vi "RF_NCS_ThoraxAbdomen_USRP_B200.vi"() -> (2 "Resp Amp":dbl[](graph), 3 "Heart Amp":dbl[](graph), 4 "# queue 2":i32)   [LabVIEW 2016]
uses:
  <instrlib>/niUSRP/niUSRP Timestamp.ctl
  <vilib>/Utility/miscctls.llb/LVDateTimeRec.ctl
  <vilib>/sound2/lvsound2.llb/Sound File Position.ctl
  <vilib>/Analysis/3filter.llb/Filter Passband Type.ctl
  <vilib>/sound2/lvsound2.llb/Sampling Mode.ctl
  <instrlib>/niUSRP/niUSRP Configure Time Start Trigger.vi
  <vilib>/Platform/browser.llb/Open URL in Default Browser (string).vi
  <instrlib>/niUSRP/niUSRP Write Tx Data (CDB).vi
  <instrlib>/niUSRP/niUSRP Fetch Rx Data (CDB).vi
  <vilib>/Analysis/3filter.llb/Butterworth Filter (DBL).vi
  <vilib>/sound2/lvsound2.llb/Sound File Info (path).vi
  <vilib>/sound2/lvsound2.llb/Sound File Read Open.vi
  <vilib>/sound2/lvsound2.llb/Sound File Read (DBL).vi
  <vilib>/sound2/lvsound2.llb/Sound Output Write (DBL).vi
  <vilib>/Analysis/3filter.llb/Butterworth Filter (CDB).vi
  <vilib>/measure/NI_MABase.lvlib
  <vilib>/Analysis/NI_AALBase.lvlib
  <vilib>/Analysis/NI_AALPro.lvlib
panel:
  in  "SDR1\nInitPhase":i32
  in  "Flush Rx2":bool
  out "String 3":string
  out "element":dbl[][](array[numeric])
  out "appended array":dbl[][](array[numeric])
  in  "SDR2 Carrier \nfrequency (Hz)":dbl=1900000000.0
  out "String 2":string
  out "size(s)":i32[](array[numeric])
  in  "Tab Control 7":enum32{"Amp2 @50kHz", "Ph2 @50kHz"}(tab)
  out "Amp2 @50 kHz":dbl[](graph)
  out "Ph2 @50 kHz":dbl[](graph)
  in  "Tab Control 6":enum32{"Amp1 @500Hz", "Ph1 @500Hz"}(tab)
  out "Amp1 @500Hz":dbl[](graph)
  out "Ph1 @500Hz":dbl[](graph)
  out "String":string
  out "#queue 3":i32
  out "#queue 2":i32
  out "# Rx2DS_Queue":i32=1
  in  "FlushSDR2":bool
  out "error out 2":errorcluster
  in  "Tab Control 8":enum32{"Rx1", "Rx2"}(tab)
  out "IQ Graph":dbl[][](graph)
  out "IQ Graph 2":dbl[][](graph)
  in  "Tab Control 5":enum32{"Amp2 @500Hz", "Ph2 @500Hz"}(tab)
  out "Amp2 @500Hz":dbl[](graph)
  out "Ph2 @500Hz":dbl[](graph)
  in  "Tab Control 4":enum32{"Tx1", "Tx2"}(tab)
  out "Tx1 Waveform Graph":waveform(dbl)[](graph)
  out "Tx2 Waveform graph":waveform(dbl)[](graph)
  in  "Stop 2":bool
  out "Tx2 Waveform":cdb[](array[numeric])
  out "Read:Tx2 IQ Rate":dbl=5000000.0
  out "Read:Rx2 IQ Rate":dbl=5000000.0
  in  "Device2 Name":refnum<k15>="MyB200_2"
  in  "Tx2 Gain":dbl=26.0 format="%#_6f"
  in  "Rx2 Gain":dbl=20.0 format="%#_6f"
  in  "Routine 3,4":T1=2 items=["Absolute"=0, "Relative"=2]
  in  "(2b) Attn Test":T1=2 items=["Absolute"=0, "Relative"=2]
  in  "Routine 5":T1=2 items=["Absolute"=0, "Relative"=2]
  in  "OpenHTML":bool=TRUE
  in  "Play sound":u16(ring) items=["No sound", "Demo normal breathing", "Demo deep breathing", "Demo fast shallow breathing", "Demo breath hold", "Demo cough", "Demo abdomen movement", "Calibration", "Routine 1", "(2a) Calm music", "(2b) Stress test", "Routine 3/4", "Routine 5"]
  in  "Demo cough":T1=2 items=["Absolute"=0, "Relative"=2]
  in  "Demo breath-hold":T1=2 items=["Absolute"=0, "Relative"=2]
  in  "Demo abdomen":T1=2 items=["Absolute"=0, "Relative"=2]
  in  "Demo fast shallow":T1=2 items=["Absolute"=0, "Relative"=2]
  in  "Play/Stop":bool
  in  "Demo normal":T1=2 items=["Absolute"=0, "Relative"=2]
  in  "Demo deep":T1=2 items=["Absolute"=0, "Relative"=2]
  out "Next Task":string
  out "Calib 5":bool caption="Time has Elapsed"
  out "Calib 4":bool caption="Time has Elapsed"
  out "Calib 3":bool caption="Time has Elapsed"
  in  "Calibration":T1=2 items=["Absolute"=0, "Relative"=2]
  out "Calib 1":bool caption="Time has Elapsed"
  out "Current Task time":dbl(slide) scale=0.0..240.0
  in  "(2a) Calm Music":T1=2 items=["Absolute"=0, "Relative"=2]
  out "#2b":bool caption="Time has Elapsed"
  in  "Routine 1":T1=2 items=["Absolute"=0, "Relative"=2]
  in  "number of samples/ch":i32=5000
  out "#5":bool caption="Time has Elapsed"
  out "#2a":bool caption="Time has Elapsed"
  out "#4":bool caption="Time has Elapsed"
  out "#3":bool caption="Time has Elapsed"
  in  "Comments":string
  in  "Tab Control 3":enum32{"Amp Heart", "Ph Heart"}(tab)
  in  "fh 1":dbl=26.0 format="%0.2f"
  in  "fl 1":dbl=0.7 format="%0.4f"
  out "Heart Ph":dbl[](graph)
  in  "fl 3":dbl=0.7 format="%0.4f"
  in  "fh 3":dbl=26.0 format="%0.2f"
  in  "Tab Control 2":enum32{"Amp1 @50kHz", "Ph1 @50kHz"}(tab)
  out "Amp1 @50 kHz":dbl[](graph)
  out "Ph1 @50 kHz":dbl[](graph)
  in  "Tab Control":enum32{"Amp Resp", "Ph Resp"}(tab)
  in  "fl 2":dbl=15.0 format="%0.4f"
  out "Resp Ph":dbl[](graph)
  in  "fl 4":dbl=15.0 format="%0.4f"
  out "ArraySz":i32[](array[numeric])
  in  "Stop Test":bool
  out "#1":bool caption="Time has Elapsed"
  out "Elapsed Time (s)":dbl
  in  "Routine":u16(ring) items=["Not Running", "Test Run", "Routine1", "Routine2a", "Routine2b", "Routine3", "Routine4", "Routine5", "Calib1", "calib3", "Calib4", "Calib5"]
  out "Read:Tx IQ Rate":dbl=5000000.0
  out "Read:Rx IQ Rate":dbl=5000000.0
  out "date time rec":T2
  out "Total Routine Time":dbl(slide) scale=0.0..240.0
  out "Current Task":string
  in  "Case Number":string="0"
  out "CaseNum":i32=1
  out "Save":bool
  out "Flush":bool
  out "Buffer":bool
  out "Output":i32=1
  out "Ch2 Amplitude":dbl step=0.05 format="%#.6g"
  out "Ch1 Amplitude":dbl step=0.05 format="%#.6g"
  out "Dis Sampling Rate":dbl=500.0 format="%#_6p"
  in  "DownSamplingRatio 2":i32=100
  out "Sampling Rate":dbl=50000.0 format="%#_6p"
  out "aapp":dbl[][](array[numeric])
  out "IterationNum":i32=1009
  in  "DownSamplingRatio":i32=40
  out "# elements in queue":i32
  out "BW/2":dbl=1000.0
  out "# queue 1":i32
  in  "Dis1":bool=TRUE
  out "Tx1 Waveform":cdb[](array[numeric])
  in  "SDR1 Carrier\nfrequency [Hz]":dbl=1820000000.0 format="%#_6p"
  out "error out":errorcluster
  in  "Start Trigger Time":T3={"whole seconds"=1, "fractional seconds"=0.0}
  in  "Stop":bool
  in  "Channel 2\nTone Amplitude":dbl=0.25000000000000006 step=0.05 format="%#.6g"
  in  "SDR2\nTone Frequency":dbl=51000.0 format="%#_6p"
  in  "Channel 1\nTone Amplitude":dbl=0.30000000000000004 step=0.05 format="%#.6g"
  in  "SDR1 \nTone Frequency":dbl=51000.0 format="%#_6p"
  in  "Waveform Size":dbl=20000.0
  in  "Device1 Name":refnum<k15>="MyB200"
  in  "Tx1 Gain":dbl=25.0 format="%#_6f"
  in  "Tx IQ Rate":dbl=2000000.0 format="%#_6p"
  in  "Rx1 Gain 1":dbl=26.0 format="%#_6f"
  in  "Rx IQ Rate":dbl=2000000.0 format="%#_6p"
  # "User Instructions"
  # "User Information"
  # "Routine Selection"
  # "Demo \nSounds"
  # "First Tx-Rx: filtered to get heartbeat signal"
  # "Second Tx-Rx: filtered to get respiration signal"
  # "SDR1"
  # "SDR2"
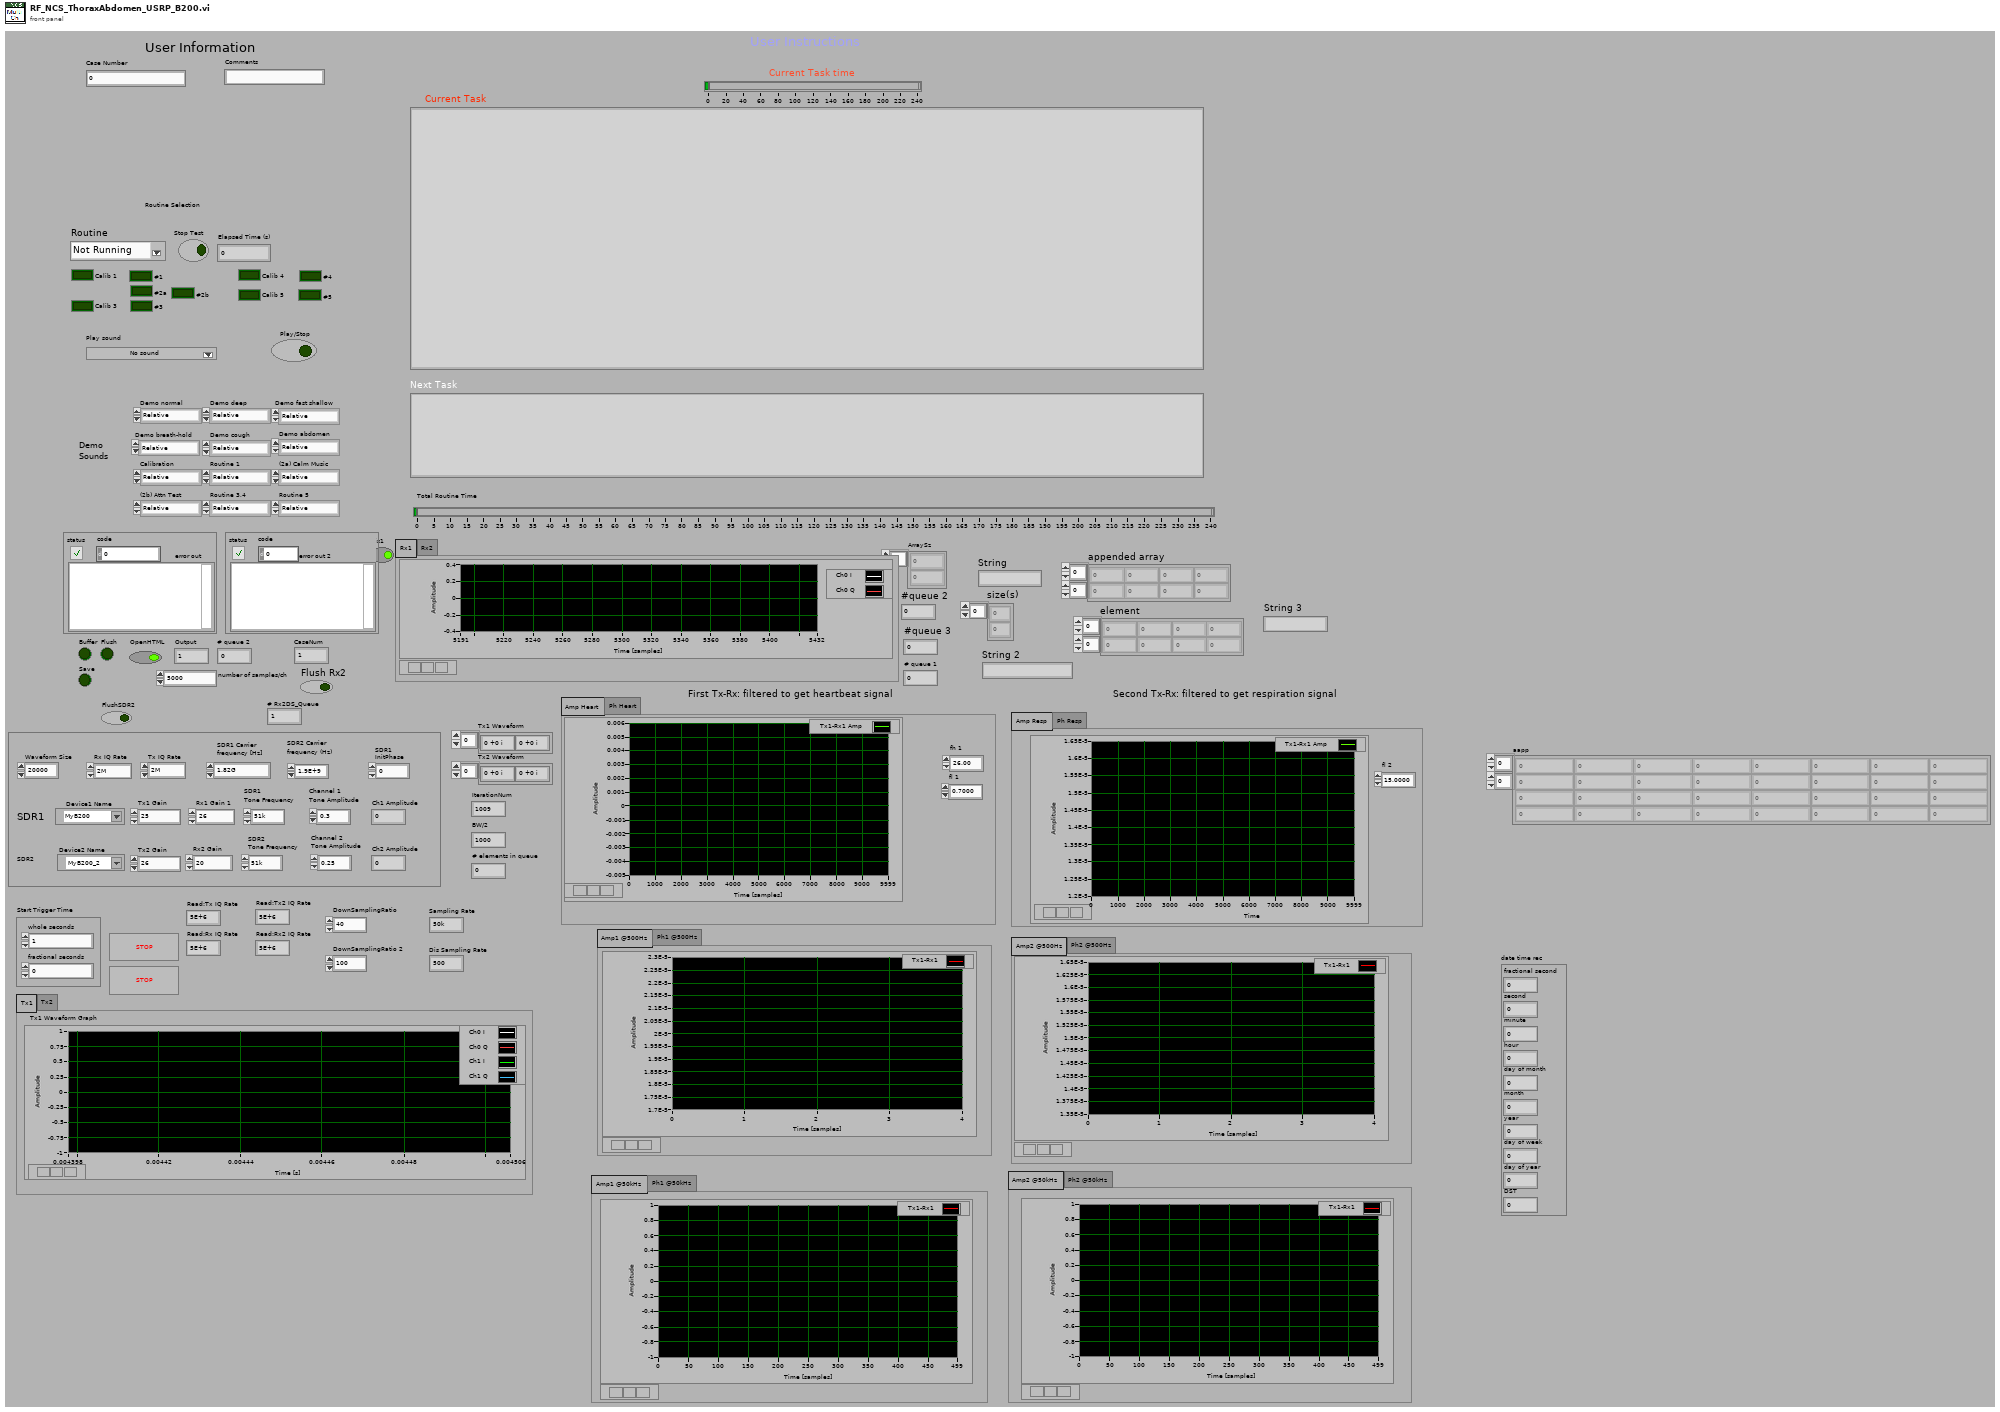
[diagram p1: front panel]
types:
  T1 = typedef "Sound File Position.ctl" = u16
  T2 = typedef "LVDateTimeRec.ctl" = cluster{"fractional second":dbl, "second":i32, "minute":i32, "hour":i32, "day of month":i32, "month":i32, "year":i32, "day of week":i32, "day of year":i32, "DST":i32}
  T3 = typedef "niUSRP Timestamp.ctl" = cluster{"whole seconds":u64, "fractional seconds":dbl}
  T4 = enum16{"Default", "Test", "Routine 1", "Routine 2a", "Routine 2b", "Routine 3", "Routine 4", "Routine 5", "Calib1", "Calib3", "Calib4", "Calib5"}
  T5 = typedef "Sampling Mode.ctl" = i32
  T6 = typedef "Sound Data Format.ctl" = cluster{"sample rate (S/s)":dbl, "number of channels":i32, "bits per sample":i32}
  T7 = typedef "Sound File Refnum.ctl" = refnum<file>
  T8 = typedef "Sound Output Task ID.ctl" = u32
  T9 = typedef "NI_AALBase.lvlib/Filter Passband Type.ctl" = enum32{"Lowpass", "Highpass", "Bandpass", "Bandstop"}
  T10 = enum16{"Default", "Test", "Routine 1", "Routine 2", "Routine 3"}
  T11 = enum16{"Default", "Test", "Routine 1", "Routine 2a", "Routine 2b", "Routine 3a", "Routine 3b", "Routine 4", "Routine 5", "Routine 6", "Routine 7", "Calib1", "Calib3", "Calib4", "Calib5", "Calib7"}
  T12 = enum16{"open", "open or create", "create or replace", "create", "open (read-only)"}
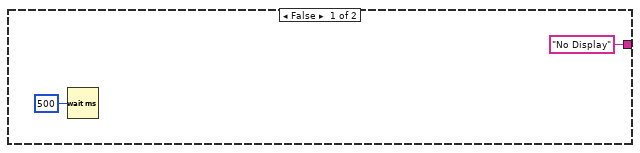
[diagram p2: hidden frame]
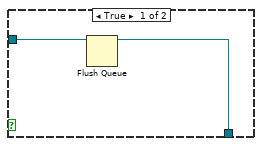
[diagram p3: hidden frame]
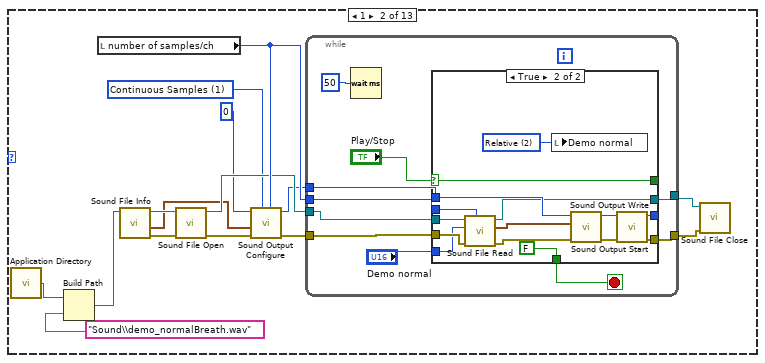
[diagram p5: hidden frame]
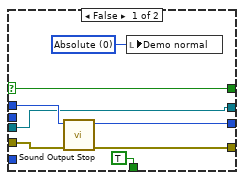
[diagram p6: hidden frame]
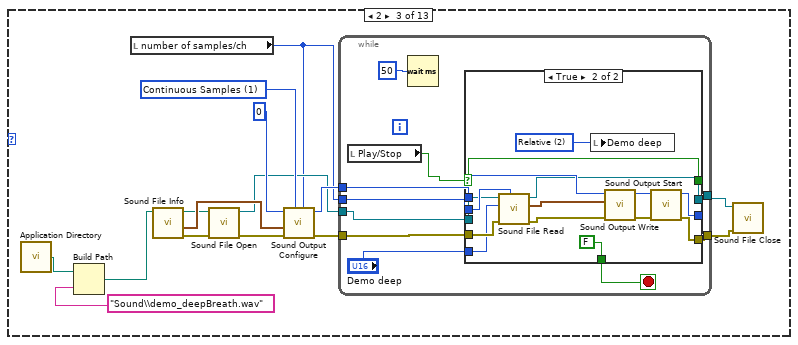
[diagram p7: hidden frame]
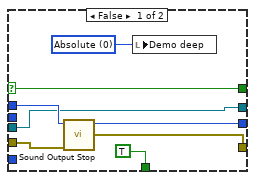
[diagram p8: hidden frame]
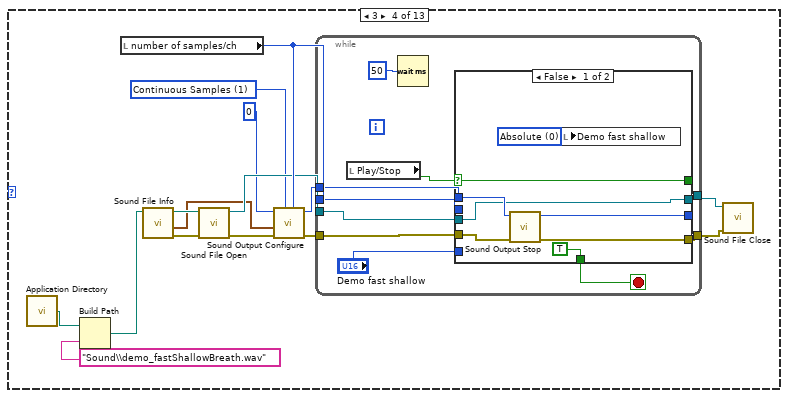
[diagram p9: hidden frame]
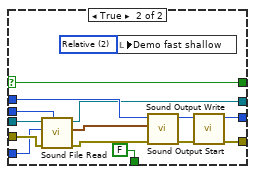
[diagram p10: hidden frame]
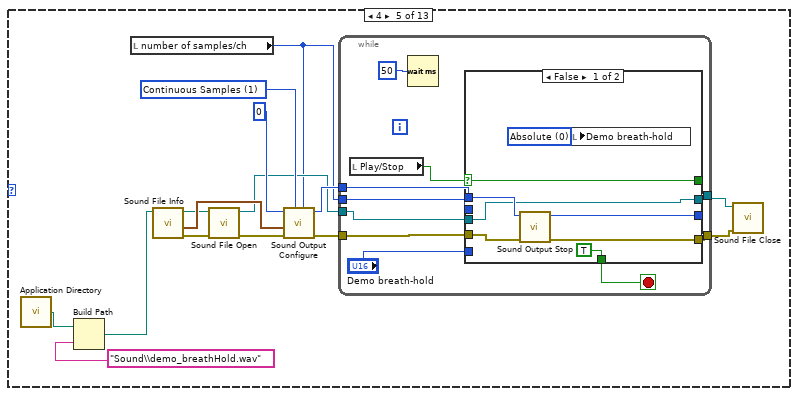
[diagram p11: hidden frame]
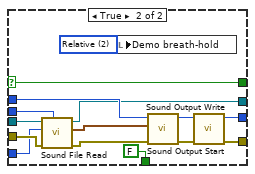
[diagram p12: hidden frame]
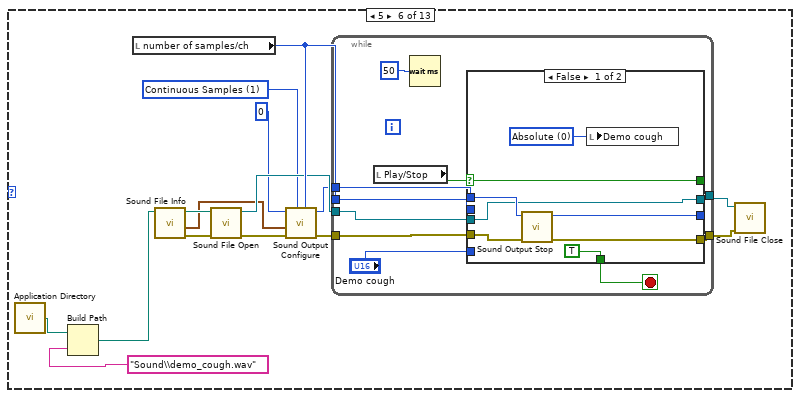
[diagram p13: hidden frame]
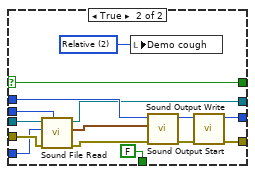
[diagram p14: hidden frame]
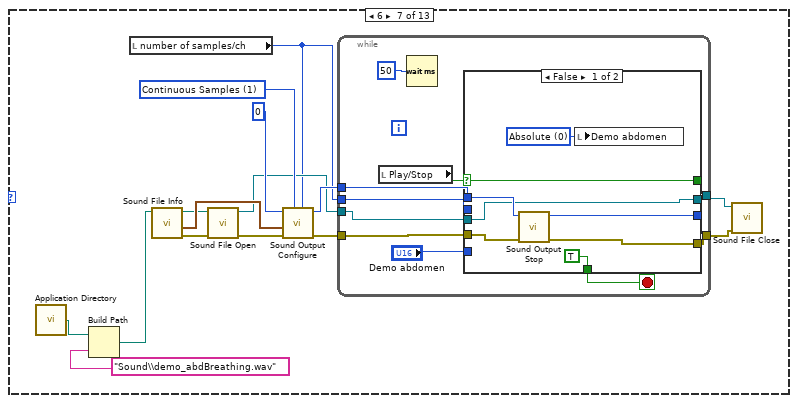
[diagram p15: hidden frame]
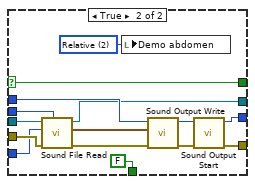
[diagram p16: hidden frame]
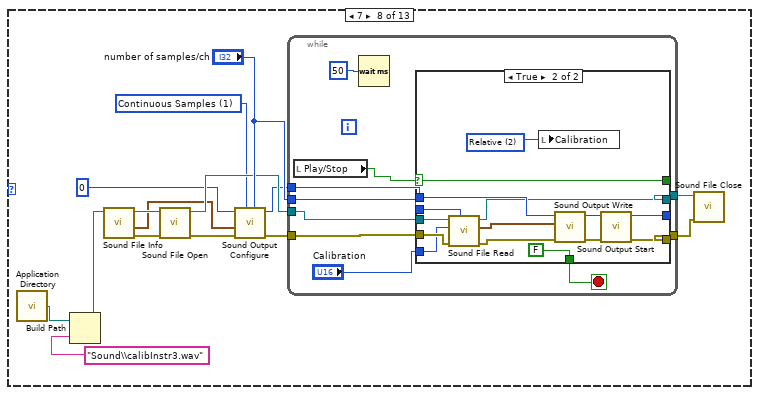
[diagram p17: hidden frame]
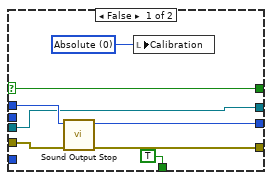
[diagram p18: hidden frame]
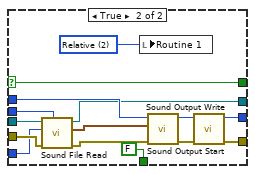
[diagram p19: hidden frame]
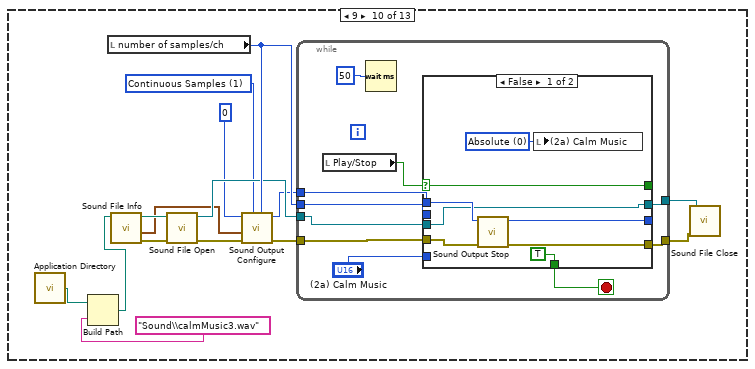
[diagram p20: hidden frame]
diagram:
  w29 = 1 items=["Now", "Next Timebase Edge"] ("apply timestamp")
  w37 = "RX2"  # Rx2 active antenna
  w95 = 0.0 ("element")
  w96 = 2000 ("dimension size")
  w103 = 4 ("dimension size")
  w130 = "RX2"  # Rx1 active antenna
  w164 = 1 items=["Now", "Next Timebase Edge"] ("apply timestamp")
  w78 = "TX1"  # Tx active antenna
  w85 = "0"  # Enabled Channels
  # "Tx2 Chain"
  # "Rx2 chain"
  # "Set the attributes \nspecific to channel 0."
  # "Set the attributes \nused by all Rx channels"
  # "Set the attributes \nspecific to Rx channel 0."
  # "Tx1 Chain"
  # "Rx1 chain"
  # "DownSamplingRatio"
  # "Set the attributes \nspecific to channel 0."
  # "Set the attributes \nused by both Rx channels"
  # "Set the attributes \nspecific to Rx channel 0."
  n1 = while {
    stop <- FALSE stop-if-true
    n2 = local read "Output"() -> (w174:i32)
    n3 = case shown="1" w174 {
      tunnel: [w179 "Channel 1\nTone Amplitude"] -> w176
      tunnel: [w179 "Channel 2\nTone Amplitude"] -> w175
      frame 0, Default {
        w179 = 0.0 ("Channel 1\nTone Amplitude")
      }
      frame 1 {
      }
    }
    "Ch1 Amplitude" <- w176
    "Ch2 Amplitude" <- w175
    n4 = Wait (ms)(milliseconds to wait=u32 50) -> ()  [unwired: 1 out]
  }
  n5 = local read "Device2 Name"() -> (w60:refnum<k15>)
  n6 = local read "Device1 Name"() -> (w169:refnum<k15>)
  n7 = call <instrlib>:"niUSRP Open Rx Session.vi"("device names"="Device2 Name") -> ("session handle out"=w59:refnum<k15>, "error out"=w58:errorcluster)  [unwired: 13 in]
  n8 = property class="niUSRP"(reference=w59, error in=w58, "Enabled Channels"=w85) -> (reference out=w57:refnum<k15>, error out=w56:errorcluster)
  n9 = call <instrlib>:"niUSRP Open Rx Session.vi"("device names"="Device1 Name") -> ("session handle out"=w163:refnum<k15>, "error out"=w162:errorcluster)  [unwired: 13 in]
  n10 = property class="niUSRP"(reference=w163, error in=w162, "Enabled Channels"=w85) -> (reference out=w161:refnum<k15>, error out=w160:errorcluster)
  n11 = call-poly <instrlib>:"niUSRP Configure Trigger.vi"("session handle"=w57, "start trigger time"="Start Trigger Time", "error in (no error)"=w56) -> ("session handle out"=w53:refnum<k15>, "error out"=w52:errorcluster)  [unwired: 11 in]
  n12 = call-poly <instrlib>:"niUSRP Configure Trigger.vi"("session handle"=w161, "start trigger time"="Start Trigger Time", "error in (no error)"=w160) -> ("session handle out"=w157:refnum<k15>, "error out"=w156:errorcluster)  [unwired: 11 in]
  n13 = property class="niUSRP"(reference=w53, error in=w52, "IQ Rate"="Rx IQ Rate") -> (reference out=w50:refnum<k15>, error out=w51:errorcluster)
  n14 = property class="niUSRP"(reference=w157, error in=w156, "IQ Rate"="Rx IQ Rate") -> (reference out=w154:refnum<k15>, error out=w155:errorcluster)
  n15 = property class="niUSRP" props=["Model"](reference=w50, error in=w51) -> (reference out=w48:refnum<k15>, error out=w49:errorcluster)  [unwired: 1 out]
  n16 = property class="niUSRP" props=["Model"](reference=w154, error in=w155) -> (reference out=w152:refnum<k15>, error out=w153:errorcluster)  [unwired: 1 out]
  n17 = property class="niUSRP"(reference=w48, error in=w49, "Carrier Frequency"="SDR2 Carrier \nfrequency (Hz)") -> (reference out=w42:refnum<k15>, error out=w41:errorcluster, "IQ Rate"=→"Read:Rx2 IQ Rate":dbl)
  n18 = property class="niUSRP"(reference=w152, error in=w153, "Carrier Frequency"="SDR1 Carrier\nfrequency [Hz]") -> (reference out=w135:refnum<k15>, error out=w134:errorcluster, "IQ Rate"=→"Read:Rx IQ Rate":dbl)
  n19 = property class="niUSRP"(reference=w42, error in=w41, "Active Channel"="0", "Gain"="Rx2 Gain", "Active Antenna"=w37) -> (reference out=w25:refnum<k15>, error out=w26:errorcluster)
  n20 = call <instrlib>:"niUSRP Open Tx Session.vi"("device names"=w60, "error in (no error)"=w26) -> ("session handle out"=w55:refnum<k15>, "error out"=w54:errorcluster)  [unwired: 12 in]
  n21 = property class="niUSRP"(reference=w55, error in=w54, "Enabled Channels"=w85) -> (reference out=w46:refnum<k15>, error out=w45:errorcluster)
  n22 = property class="niUSRP" props=["IQ Rate", "IQ Rate"](reference=w46, error in=w45, "IQ Rate"="Tx IQ Rate") -> (reference out=w35:refnum<k15>, error out=w34:errorcluster)  [unwired: 1 out]
  n23 = property class="niUSRP"(reference=w35, error in=w34, "Carrier Frequency"="SDR2 Carrier \nfrequency (Hz)") -> (reference out=w39:refnum<k15>, error out=w38:errorcluster, "IQ Rate"=w10:dbl)
  "Read:Tx2 IQ Rate" <- w10
  n24 = property class="niUSRP"(reference=w39, error in=w38, "Active Channel"="0", "Gain"="Tx2 Gain", "Active Antenna"=w78) -> (reference out=w33:refnum<k15>, error out=w32:errorcluster)
  n25 = property class="niUSRP"(reference=w135, error in=w134, "Active Channel"="0", "Gain"="Rx1 Gain 1", "Active Antenna"=w130) -> (reference out=w81:refnum<k15>, error out=w80:errorcluster)
  n26 = call <instrlib>:"niUSRP Open Tx Session.vi"("device names"=w169, "error in (no error)"=w80) -> ("session handle out"=w159:refnum<k15>, "error out"=w158:errorcluster)  [unwired: 12 in]
  n27 = property class="niUSRP"(reference=w159, error in=w158, "Enabled Channels"=w85) -> (reference out=w150:refnum<k15>, error out=w149:errorcluster)
  n28 = property class="niUSRP"(reference=w150, error in=w149, "IQ Rate"="Tx IQ Rate") -> (reference out=w87:refnum<k15>, error out=w86:errorcluster, "IQ Rate"=w148:dbl)
  n29 = property class="niUSRP"(reference=w87, error in=w86, "Carrier Frequency"="SDR1 Carrier\nfrequency [Hz]") -> (reference out=w132:refnum<k15>, error out=w131:errorcluster, "IQ Rate"=→"Read:Tx IQ Rate":dbl)
  n30 = property class="niUSRP"(reference=w132, error in=w131, "Active Channel"="0", "Gain"="Tx1 Gain", "Active Antenna"=w78) -> (reference out=w82:refnum<k15>, error out=w83:errorcluster)
  n31 = call <instrlib>:"niUSRP Commit.vi"("session handle"=w33, "error in (no error)"=w32) -> ("session handle out"=w7:refnum<k15>, "error out"=w24:errorcluster)  [unwired: 12 in]
  n32 = call <instrlib>:"niUSRP Commit.vi"("session handle"=w82, "error in (no error)"=w83) -> ("session handle out"=w171:refnum<k15>, "error out"=w172:errorcluster)  [unwired: 12 in]
  n33 = Merge Errors(w26, w24) -> (w27:errorcluster)
  n34 = call <instrlib>:"niUSRP Set Time.vi"("session handle"=w25, "apply timestamp"=w29, "timestamp"=T3 {"whole seconds"=0, "fractional seconds"=0.0}, "error in (no error)"=w27) -> ("session handle out"=w31:refnum<k15>, "error out"=w30:errorcluster)  [unwired: 10 in]
  n35 = call <instrlib>:"niUSRP Initiate.vi"("session handle"=w31, "error in (no error)"=w30) -> ("session handle out"=w11:refnum<k15>, "error out"=w1:errorcluster)  [unwired: 12 in]
  n36 = Merge Errors(w80, w172) -> (w100:errorcluster)
  n37 = local read "Waveform Size"() -> (w12:dbl)
  n38 = Initialize Array(cdb 0.0+0.0i ("element"), w12) -> (w14:cdb[])
  n39 = call <instrlib>:"niUSRP Set Time.vi"("session handle"=w81, "apply timestamp"=w164, "timestamp"=T3 {"whole seconds"=0, "fractional seconds"=0.0}, "error in (no error)"=w100) -> ("session handle out"=w166:refnum<k15>, "error out"=w165:errorcluster)  [unwired: 10 in]
  n40 = Obtain Queue(max queue size (-1, unlimited)=-1, name (unnamed)="Rx2Queue", element data type=w14) -> (queue out=w71:refnum<queue>)  [unwired: 2 in, 2 out]
  n41 = local read "Waveform Size"() -> (w90:dbl)
  n42 = call <instrlib>:"niUSRP Initiate.vi"("session handle"=w166, "error in (no error)"=w165) -> ("session handle out"=w173:refnum<k15>, "error out"=w88:errorcluster)  [unwired: 12 in]
  n43 = while {
    tunnel: w148 -> [w192]
    tunnel: w88 -> [w187]
    stop <- FALSE stop-if-true
    # "Generate I and Q waveforms."
    n44 = Wait (ms)(milliseconds to wait=u32 100) -> ()  [unwired: 1 out]
    n45 = local read "Ch1 Amplitude"() -> (w186:dbl)
    n46 = Bundle By Name(cluster=cluster{"Fs":dbl, "#s":dbl} {"Fs"=1000.0, "#s"=1000.0} ("sampling info"), "Fs"=w192, "#s"="Waveform Size") -> (w193:cluster{"Fs":dbl, "#s":dbl})
    n47 = Add(x=90.0 ("phase"), y="SDR1\nInitPhase") -> (x+y=w183:dbl)
    n48 = call <vilib>:"Sine Waveform.vi"("sampling info"=w193, "error in (no error)"=w187, "phase"=w183, "amplitude"=w186, "frequency"="SDR1 \nTone Frequency") -> ("error out"=w190:errorcluster, "signal out"=w197:waveform(dbl))  [unwired: 5 in]
    n49 = call <vilib>:"Sine Waveform.vi"("sampling info"=w193, "error in (no error)"=w187, "phase"="SDR1\nInitPhase", "amplitude"=w186, "frequency"="SDR1 \nTone Frequency") -> ("error out"=w191:errorcluster, "signal out"=w198:waveform(dbl))  [unwired: 5 in]
    n50 = Merge Errors(w190, w191) -> ()  [unwired: 1 out]
    n51 = Build Array(w197, w198) -> (→"Tx1 Waveform Graph":waveform(dbl)[])
    n52 = Unbundle By Name(w197) -> ("Y"=w196:dbl[])
    n53 = Unbundle By Name(w198) -> ("Y"=w195:dbl[])
    n54 = Re/Im To Complex(1:w195, 2:w196) -> (0:→"Tx1 Waveform":cdb[])
  }
  n55 = while {
    tunnel: w71 -> [w204]
    stop <- FALSE stop-if-true
    n56 = local read "Dis1"() -> (w203:bool)
    n57 = Wait (ms)(milliseconds to wait=u32 5) -> ()  [unwired: 1 out]
    n58 = case shown="True" w203 {
      tunnel: w204 -> [_ w211]
      tunnel: ["No Display" "Displaying Rx2 "] -> w202
      frame False {
        n59 = Wait (ms)(milliseconds to wait=u32 500) -> ()  [unwired: 1 out]
      }
      frame True {
        n60 = Preview Queue Element(queue=w211) -> (element=w213:cdb[])  [unwired: 2 in, 3 out]
        n61 = for {
          N: 1 -> [_]
          tunnel: w213 -> [w219]
          shift-right: [w216] -> w212
          shift-left: dbl[][] [] -> [w215]
          n62 = Complex To Re/Im(x + iy=w219) -> (x=w218:dbl[], y=w217:dbl[])
          n63 = Build Array (concatenate)(w215, w218, w217) -> (w216:dbl[][])
        }
        "IQ Graph 2" <- w212
      }
    }
    "String" <- w202
  }
  n64 = while {
    tunnel: w11 -> [w231]
    tunnel: w1 -> [w230]
    tunnel: [w226] -> w21
    tunnel: [w229] -> w18
    shift-right: [w222] -> _
    shift-left: w71 -> [w223]
    stop <- w225 stop-if-true
    # "Rx2"
    n65 = local read "Waveform Size"() -> (w224:dbl)
    n66 = call-poly <instrlib>:"niUSRP Fetch Rx Data (poly).vi"("session handle"=w231, "number of samples"=w224, "error in (no error)"=w230) -> ("session handle out"=w229:refnum<k15>, "data"=w220:cdb[], "timestamp"=w221:T3, "error out"=w226:errorcluster)  [unwired: 9 in]
    n67 = call <instrlib>:"niUSRP USRP Timestamp to LV Timestamp.vi"("USRP Timestamp"=w221) -> ()  [unwired: 13 in, 2 out]
    n68 = Enqueue Element(queue=w223, element=w220) -> (queue out=w222:refnum<queue>)  [unwired: 2 in, 2 out]
    n69 = Unbundle By Name(w226) -> ("status"=w228:bool)
    n70 = Or(x=w228, y="Stop 2") -> (x .or. y?=w225:bool)
  }
  n71 = while {
    tunnel: w10 -> [w241]
    tunnel: w1 -> [w232]
    stop <- FALSE stop-if-true
    # "Generate I and Q waveforms."
    n72 = local read "Waveform Size"() -> (w233:dbl)
    n73 = Wait (ms)(milliseconds to wait=u32 100) -> ()  [unwired: 1 out]
    n74 = Bundle By Name(cluster=cluster{"Fs":dbl, "#s":dbl} {"Fs"=1000.0, "#s"=1000.0} ("sampling info"), "Fs"=w241, "#s"=w233) -> (w242:cluster{"Fs":dbl, "#s":dbl})
    n75 = local read "Ch2 Amplitude"() -> (w236:dbl)
    n76 = call <vilib>:"Sine Waveform.vi"("sampling info"=w242, "error in (no error)"=w232, "phase"=90.0, "amplitude"=w236, "frequency"="SDR2\nTone Frequency") -> ("error out"=w239:errorcluster, "signal out"=w247:waveform(dbl))  [unwired: 5 in]
    n77 = call <vilib>:"Sine Waveform.vi"("sampling info"=w242, "error in (no error)"=w232, "amplitude"=w236, "frequency"="SDR2\nTone Frequency") -> ("error out"=w240:errorcluster, "signal out"=w248:waveform(dbl))  [unwired: 6 in]
    n78 = Merge Errors(w239, w240) -> ()  [unwired: 1 out]
    n79 = Build Array(w247, w248) -> (→"Tx2 Waveform graph":waveform(dbl)[])
    n80 = Unbundle By Name(w247) -> ("Y"=w246:dbl[])
    n81 = Unbundle By Name(w248) -> ("Y"=w245:dbl[])
    n82 = Re/Im To Complex(1:w245, 2:w246) -> (0:→"Tx2 Waveform":cdb[])
  }
  n83 = Initialize Array(cdb 0.0+0.0i ("element"), w90) -> (w127:cdb[])
  n84 = Obtain Queue(max queue size (-1, unlimited)=-1, name (unnamed)="Rx1Queue", element data type=w127) -> (queue out=w91:refnum<queue>)  [unwired: 2 in, 2 out]
  n85 = while {
    tunnel: w173 -> [w261]
    tunnel: w88 -> [w260]
    tunnel: [w256] -> w144
    tunnel: [w259] -> w141
    shift-right: [w252] -> _
    shift-left: w91 -> [w253]
    stop <- w255 stop-if-true
    # "Rx"
    n86 = local read "Waveform Size"() -> (w254:dbl)
    n87 = call-poly <instrlib>:"niUSRP Fetch Rx Data (poly).vi"("session handle"=w261, "number of samples"=w254, "error in (no error)"=w260) -> ("session handle out"=w259:refnum<k15>, "data"=w250:cdb[], "timestamp"=w251:T3, "error out"=w256:errorcluster)  [unwired: 9 in]
    n88 = call <instrlib>:"niUSRP USRP Timestamp to LV Timestamp.vi"("USRP Timestamp"=w251) -> ()  [unwired: 13 in, 2 out]
    n89 = Enqueue Element(queue=w253, element=w250) -> (queue out=w252:refnum<queue>)  [unwired: 2 in, 2 out]
    n90 = Unbundle By Name(w256) -> ("status"=w258:bool)
    n91 = Or(x=w258, y="Stop") -> (x .or. y?=w255:bool)
  }
  n92 = while {
    tunnel: w91 -> [w263]
    stop <- FALSE stop-if-true
    n93 = Wait (ms)(milliseconds to wait=u32 5) -> ()  [unwired: 1 out]
    n94 = case shown="True" "Dis1" {
      tunnel: w263 -> [_ w268]
      frame False {
        n95 = Wait (ms)(milliseconds to wait=u32 500) -> ()  [unwired: 1 out]
      }
      frame True {
        n96 = Preview Queue Element(queue=w268) -> (element=w270:cdb[])  [unwired: 2 in, 3 out]
        n97 = for {
          N: 1 -> [_]
          tunnel: w270 -> [w276]
          shift-right: [w273] -> w269
          shift-left: dbl[][] [] -> [w272]
          n98 = Complex To Re/Im(x + iy=w276) -> (x=w275:dbl[], y=w274:dbl[])
          n99 = Build Array (concatenate)(w272, w275, w274) -> (w273:dbl[][])
        }
        "IQ Graph" <- w269
      }
    }
  }
  n100 = while {
    tunnel: w171 -> [w284]
    tunnel: w88 -> [w283]
    tunnel: [w281] -> w146
    tunnel: [w279] -> w139
    stop <- w280 stop-if-true
    # "Tx on SDR1"
    n101 = local read "Tx1 Waveform"() -> (w277:cdb[])
    n102 = local read "Stop"() -> (w278:bool)
    n103 = call-poly <instrlib>:"niUSRP Write Tx Data (poly).vi"("session handle"=w284, "data"=w277, "end of data?"=w278, "error in (no error)"=w283) -> ("session handle out"=w279:refnum<k15>, "error out"=w281:errorcluster)  [unwired: 10 in]
    n104 = Unbundle By Name(w281) -> ("status"=w282:bool)
    n105 = Compound Arithmetic op=OR(w282, w278) -> (w280:bool)
  }
  n106 = while {
    tunnel: w7 -> [w292]
    tunnel: w1 -> [w291]
    tunnel: [w289] -> w5
    tunnel: [w287] -> w6
    stop <- w288 stop-if-true
    # "Tx on SDR2"
    n107 = local read "Tx2 Waveform"() -> (w285:cdb[])
    n108 = local read "Stop 2"() -> (w286:bool)
    n109 = call-poly <instrlib>:"niUSRP Write Tx Data (poly).vi"("session handle"=w292, "data"=w285, "end of data?"=w286, "error in (no error)"=w291) -> ("session handle out"=w287:refnum<k15>, "error out"=w289:errorcluster)  [unwired: 10 in]
    n110 = Unbundle By Name(w289) -> ("status"=w290:bool)
    n111 = Compound Arithmetic op=OR(w290, w286) -> (w288:bool)
  }
  n112 = flat-sequence {
    tunnel: [w294] -> w20
    tunnel: w21 -> [w294]
    tunnel: [w293] -> w19
    tunnel: w18 -> [w293]
    frame #0 {
      n113 = local write "Stop 2"(TRUE ("STOP")) -> ()
    }
  }
  n114 = call <instrlib>:"niUSRP Abort.vi"("session handle"=w19, "error in (no error)"=w20) -> ("session handle out"=w23:refnum<k15>, "error out"=w22:errorcluster)  [unwired: 12 in]
  n115 = flat-sequence {
    tunnel: [w297] -> w145
    tunnel: w146 -> [w297]
    tunnel: [w296] -> w140
    tunnel: w139 -> [w296]
    frame #0 {
      n116 = local write "Stop"(TRUE ("STOP")) -> ()
    }
  }
  n117 = call <instrlib>:"niUSRP Close Session.vi"("session handle"=w23, "error in (no error)"=w22) -> ("error out"=w17:errorcluster)  [unwired: 13 in]
  n118 = flat-sequence {
    tunnel: [w300] -> w143
    tunnel: w144 -> [w300]
    tunnel: [w299] -> w142
    tunnel: w141 -> [w299]
    frame #0 {
      n119 = local write "Stop"(TRUE ("STOP")) -> ()
    }
  }
  n120 = flat-sequence {
    tunnel: w17 -> [w304]
    tunnel: w2 -> [w303]
    tunnel: [w302] -> w75
    frame #0 {
      n121 = Merge Errors(w304, w303) -> (w302:errorcluster)
      n122 = local write "Stop 2"(FALSE ("STOP")) -> ()
    }
  }
  n123 = flat-sequence {
    tunnel: [w307] -> w3
    tunnel: w5 -> [w307]
    tunnel: [w306] -> w4
    tunnel: w6 -> [w306]
    frame #0 {
      n124 = local write "Stop 2"(TRUE ("STOP")) -> ()
    }
  }
  n125 = call <instrlib>:"niUSRP Abort.vi"("session handle"=w142, "error in (no error)"=w143) -> ("session handle out"=w168:refnum<k15>, "error out"=w167:errorcluster)  [unwired: 12 in]
  n126 = call <instrlib>:"niUSRP Close Session.vi"("session handle"=w168, "error in (no error)"=w167) -> ("error out"=w138:errorcluster)  [unwired: 13 in]
  n127 = while {
    stop <- FALSE stop-if-true
    n128 = Wait (ms)(milliseconds to wait=u32 50) -> ()  [unwired: 1 out]
    n129 = case shown="8" "Play sound" {
      frame 0, Default {
      }
      frame 1 {
        w315 = T5 1 items=["Finite Samples", "Continuous Samples"] ("sample mode")
        n130 = call <vilib>:"Application Directory.vi"() -> ("Application Directory"=w314:path)
        n131 = Build Path(base path=w314, name or relative path="Sound\\demo_normalBreath.wav" ("path")) -> (appended path=w312:path)
        n132 = local read "number of samples/ch"() -> (w326:i32)
        n133 = call-poly <vilib>:"Sound File Info.vi"("path"=w312) -> ("error out"=w319:errorcluster, "sound format"=w318:T6, "path out"=w320:path)  [unwired: 7 in, 1 out]
        n134 = call-poly <vilib>:"Sound File Open.vi"("error in (no error)"=w319, "path"=w320) -> ("error out"=w316:errorcluster, "sound file refnum"=w323:T7)  [unwired: 8 in]
        n135 = call <vilib>:"Sound Output Configure.vi"("number of samples/ch"=w326, "sample mode"=w315, "error in (no error)"=w316, "sound format"=w318, "device ID"=u32 0) -> ("error out"=w324:errorcluster, "task ID"=w322:T8)  [unwired: 5 in]
        n136 = while {
          tunnel: w322 -> [w336]
          tunnel: [w335] -> w321
          tunnel: w323 -> [w330]
          tunnel: w324 -> [w329]
          tunnel: w326 -> [w331]
          tunnel: [w334] -> w325
          stop <- w327 stop-if-true
          n137 = Wait (ms)(milliseconds to wait=u32 50) -> ()  [unwired: 1 out]
          n138 = case shown="True" "Play/Stop" {
            selector: "Play/Stop" -> [w341 w359]
            tunnel: w336 -> [w344 w356]
            tunnel: [w342 w358] -> w335
            tunnel: [w343 w357] -> _
            tunnel: [w341 w359] -> _
            tunnel: [w339 w353] -> w334
            tunnel: w331 -> [_ w350]
            tunnel: w330 -> [w339 w349]
            tunnel: w329 -> [w340 w348]
            tunnel: "Demo normal" -> [_ w347]
            tunnel: [TRUE FALSE] -> w327
            frame False {
              w338 = T1 0 items=["Absolute"=0, "Relative"=2] ("position mode")
              n139 = call <vilib>:"Sound Output Stop.vi"("error in (no error)"=w340, "task ID"=w344) -> ("error out"=w342:errorcluster, "task ID out"=w343:T8)  [unwired: 8 in]
              n140 = local write "Demo normal"(w338) -> ()
            }
            frame True {
              w346 = T1 2 items=["Absolute"=0, "Relative"=2] ("position mode")
              n141 = call-poly <vilib>:"Sound File Read.vi"("number of samples/ch (-1: all)"=w350, "error in (no error)"=w348, "position mode"=w347, "sound file refnum"=w349) -> ("error out"=w352:errorcluster, "data"=w351:waveform(dbl)[], "sound file refnum out"=w353:T7)  [unwired: 3 in, 2 out]
              n142 = local write "Demo normal"(w346) -> ()
              n143 = call-poly <vilib>:"Sound Output Write.vi"("error in (no error)"=w352, "data"=w351, "task ID"=w356) -> ("error out"=w354:errorcluster, "task ID out"=w355:T8)  [unwired: 7 in]
              n144 = call <vilib>:"Sound Output Start.vi"("error in (no error)"=w354, "task ID"=w355) -> ("error out"=w358:errorcluster, "task ID out"=w357:T8)  [unwired: 8 in]
            }
          }
        }
        n145 = call <vilib>:"Sound File Close.vi"("error in (no error)"=w321, "sound file refnum"=w325) -> ()  [unwired: 9 in, 1 out]
      }
      frame 2 {
        w374 = T5 1 items=["Finite Samples", "Continuous Samples"] ("sample mode")
        n146 = call <vilib>:"Application Directory.vi"() -> ("Application Directory"=w362:path)
        n147 = Build Path(base path=w362, name or relative path="Sound\\demo_deepBreath.wav" ("path")) -> (appended path=w360:path)
        n148 = local read "number of samples/ch"() -> (w363:i32)
        n149 = call-poly <vilib>:"Sound File Info.vi"("path"=w360) -> ("error out"=w370:errorcluster, "sound format"=w371:T6, "path out"=w369:path)  [unwired: 7 in, 1 out]
        n150 = call-poly <vilib>:"Sound File Open.vi"("error in (no error)"=w370, "path"=w369) -> ("error out"=w373:errorcluster, "sound file refnum"=w366:T7)  [unwired: 8 in]
        n151 = call <vilib>:"Sound Output Configure.vi"("number of samples/ch"=w363, "sample mode"=w374, "error in (no error)"=w373, "sound format"=w371, "device ID"=u32 0) -> ("error out"=w365:errorcluster, "task ID"=w367:T8)  [unwired: 5 in]
        n152 = while {
          tunnel: w367 -> [w384]
          tunnel: [w383] -> w368
          tunnel: w366 -> [w379]
          tunnel: w365 -> [w378]
          tunnel: w363 -> [w380]
          tunnel: [w382] -> w364
          stop <- w376 stop-if-true
          n153 = local read "Play/Stop"() -> (w375:bool)
          n154 = Wait (ms)(milliseconds to wait=u32 50) -> ()  [unwired: 1 out]
          n155 = case shown="True" w375 {
            selector: w375 -> [w389 w407]
            tunnel: w384 -> [w392 w404]
            tunnel: [w390 w406] -> w383
            tunnel: [w391 w405] -> _
            tunnel: [w389 w407] -> _
            tunnel: [w387 w401] -> w382
            tunnel: w380 -> [_ w398]
            tunnel: w379 -> [w387 w397]
            tunnel: w378 -> [w388 w396]
            tunnel: "Demo deep" -> [_ w395]
            tunnel: [TRUE FALSE] -> w376
            frame False {
              w386 = T1 0 items=["Absolute"=0, "Relative"=2] ("position mode")
              n156 = call <vilib>:"Sound Output Stop.vi"("error in (no error)"=w388, "task ID"=w392) -> ("error out"=w390:errorcluster, "task ID out"=w391:T8)  [unwired: 8 in]
              n157 = local write "Demo deep"(w386) -> ()
            }
            frame True {
              w394 = T1 2 items=["Absolute"=0, "Relative"=2] ("position mode")
              n158 = call-poly <vilib>:"Sound File Read.vi"("number of samples/ch (-1: all)"=w398, "error in (no error)"=w396, "position mode"=w395, "sound file refnum"=w397) -> ("error out"=w400:errorcluster, "data"=w399:waveform(dbl)[], "sound file refnum out"=w401:T7)  [unwired: 3 in, 2 out]
              n159 = local write "Demo deep"(w394) -> ()
              n160 = call-poly <vilib>:"Sound Output Write.vi"("error in (no error)"=w400, "data"=w399, "task ID"=w404) -> ("error out"=w402:errorcluster, "task ID out"=w403:T8)  [unwired: 7 in]
              n161 = call <vilib>:"Sound Output Start.vi"("error in (no error)"=w402, "task ID"=w403) -> ("error out"=w406:errorcluster, "task ID out"=w405:T8)  [unwired: 8 in]
            }
          }
        }
        n162 = call <vilib>:"Sound File Close.vi"("error in (no error)"=w368, "sound file refnum"=w364) -> ()  [unwired: 9 in, 1 out]
      }
      frame 3 {
        w411 = T5 1 items=["Finite Samples", "Continuous Samples"] ("sample mode")
        n163 = call <vilib>:"Application Directory.vi"() -> ("Application Directory"=w410:path)
        n164 = Build Path(base path=w410, name or relative path="Sound\\demo_fastShallowBreath.wav" ("path")) -> (appended path=w408:path)
        n165 = local read "number of samples/ch"() -> (w422:i32)
        n166 = call-poly <vilib>:"Sound File Info.vi"("path"=w408) -> ("error out"=w415:errorcluster, "sound format"=w414:T6, "path out"=w416:path)  [unwired: 7 in, 1 out]
        n167 = call-poly <vilib>:"Sound File Open.vi"("error in (no error)"=w415, "path"=w416) -> ("error out"=w412:errorcluster, "sound file refnum"=w419:T7)  [unwired: 8 in]
        n168 = call <vilib>:"Sound Output Configure.vi"("number of samples/ch"=w422, "sample mode"=w411, "error in (no error)"=w412, "sound format"=w414, "device ID"=u32 0) -> ("error out"=w420:errorcluster, "task ID"=w418:T8)  [unwired: 5 in]
        n169 = while {
          tunnel: w418 -> [w432]
          tunnel: [w431] -> w417
          tunnel: w419 -> [w427]
          tunnel: w420 -> [w426]
          tunnel: w422 -> [w428]
          tunnel: [w430] -> w421
          stop <- w424 stop-if-true
          n170 = local read "Play/Stop"() -> (w423:bool)
          n171 = Wait (ms)(milliseconds to wait=u32 50) -> ()  [unwired: 1 out]
          n172 = case shown="False" w423 {
            selector: w423 -> [w437 w455]
            tunnel: w432 -> [w440 w452]
            tunnel: [w438 w454] -> w431
            tunnel: [w439 w453] -> _
            tunnel: [w437 w455] -> _
            tunnel: [w435 w449] -> w430
            tunnel: w428 -> [_ w446]
            tunnel: w427 -> [w435 w445]
            tunnel: w426 -> [w436 w444]
            tunnel: "Demo fast shallow" -> [_ w443]
            tunnel: [TRUE FALSE] -> w424
            frame False {
              w434 = T1 0 items=["Absolute"=0, "Relative"=2] ("position mode")
              n173 = call <vilib>:"Sound Output Stop.vi"("error in (no error)"=w436, "task ID"=w440) -> ("error out"=w438:errorcluster, "task ID out"=w439:T8)  [unwired: 8 in]
              n174 = local write "Demo fast shallow"(w434) -> ()
            }
            frame True {
              w442 = T1 2 items=["Absolute"=0, "Relative"=2] ("position mode")
              n175 = call-poly <vilib>:"Sound File Read.vi"("number of samples/ch (-1: all)"=w446, "error in (no error)"=w444, "position mode"=w443, "sound file refnum"=w445) -> ("error out"=w448:errorcluster, "data"=w447:waveform(dbl)[], "sound file refnum out"=w449:T7)  [unwired: 3 in, 2 out]
              n176 = local write "Demo fast shallow"(w442) -> ()
              n177 = call-poly <vilib>:"Sound Output Write.vi"("error in (no error)"=w448, "data"=w447, "task ID"=w452) -> ("error out"=w450:errorcluster, "task ID out"=w451:T8)  [unwired: 7 in]
              n178 = call <vilib>:"Sound Output Start.vi"("error in (no error)"=w450, "task ID"=w451) -> ("error out"=w454:errorcluster, "task ID out"=w453:T8)  [unwired: 8 in]
            }
          }
        }
        n179 = call <vilib>:"Sound File Close.vi"("error in (no error)"=w417, "sound file refnum"=w421) -> ()  [unwired: 9 in, 1 out]
      }
      frame 4 {
        w470 = T5 1 items=["Finite Samples", "Continuous Samples"] ("sample mode")
        n180 = call <vilib>:"Application Directory.vi"() -> ("Application Directory"=w458:path)
        n181 = Build Path(base path=w458, name or relative path="Sound\\demo_breathHold.wav" ("path")) -> (appended path=w456:path)
        n182 = local read "number of samples/ch"() -> (w459:i32)
        n183 = call-poly <vilib>:"Sound File Info.vi"("path"=w456) -> ("error out"=w466:errorcluster, "sound format"=w467:T6, "path out"=w465:path)  [unwired: 7 in, 1 out]
        n184 = call-poly <vilib>:"Sound File Open.vi"("error in (no error)"=w466, "path"=w465) -> ("error out"=w469:errorcluster, "sound file refnum"=w462:T7)  [unwired: 8 in]
        n185 = call <vilib>:"Sound Output Configure.vi"("number of samples/ch"=w459, "sample mode"=w470, "error in (no error)"=w469, "sound format"=w467, "device ID"=u32 0) -> ("error out"=w461:errorcluster, "task ID"=w463:T8)  [unwired: 5 in]
        n186 = while {
          tunnel: w463 -> [w480]
          tunnel: [w479] -> w464
          tunnel: w462 -> [w475]
          tunnel: w461 -> [w474]
          tunnel: w459 -> [w476]
          tunnel: [w478] -> w460
          stop <- w472 stop-if-true
          n187 = local read "Play/Stop"() -> (w471:bool)
          n188 = Wait (ms)(milliseconds to wait=u32 50) -> ()  [unwired: 1 out]
          n189 = case shown="False" w471 {
            selector: w471 -> [w485 w503]
            tunnel: w480 -> [w488 w500]
            tunnel: [w486 w502] -> w479
            tunnel: [w487 w501] -> _
            tunnel: [w485 w503] -> _
            tunnel: [w483 w497] -> w478
            tunnel: w476 -> [_ w494]
            tunnel: w475 -> [w483 w493]
            tunnel: w474 -> [w484 w492]
            tunnel: "Demo breath-hold" -> [_ w491]
            tunnel: [TRUE FALSE] -> w472
            frame False {
              w482 = T1 0 items=["Absolute"=0, "Relative"=2] ("position mode")
              n190 = call <vilib>:"Sound Output Stop.vi"("error in (no error)"=w484, "task ID"=w488) -> ("error out"=w486:errorcluster, "task ID out"=w487:T8)  [unwired: 8 in]
              n191 = local write "Demo breath-hold"(w482) -> ()
            }
            frame True {
              w490 = T1 2 items=["Absolute"=0, "Relative"=2] ("position mode")
              n192 = call-poly <vilib>:"Sound File Read.vi"("number of samples/ch (-1: all)"=w494, "error in (no error)"=w492, "position mode"=w491, "sound file refnum"=w493) -> ("error out"=w496:errorcluster, "data"=w495:waveform(dbl)[], "sound file refnum out"=w497:T7)  [unwired: 3 in, 2 out]
              n193 = local write "Demo breath-hold"(w490) -> ()
              n194 = call-poly <vilib>:"Sound Output Write.vi"("error in (no error)"=w496, "data"=w495, "task ID"=w500) -> ("error out"=w498:errorcluster, "task ID out"=w499:T8)  [unwired: 7 in]
              n195 = call <vilib>:"Sound Output Start.vi"("error in (no error)"=w498, "task ID"=w499) -> ("error out"=w502:errorcluster, "task ID out"=w501:T8)  [unwired: 8 in]
            }
          }
        }
        n196 = call <vilib>:"Sound File Close.vi"("error in (no error)"=w464, "sound file refnum"=w460) -> ()  [unwired: 9 in, 1 out]
      }
      frame 5 {
        w507 = T5 1 items=["Finite Samples", "Continuous Samples"] ("sample mode")
        n197 = call <vilib>:"Application Directory.vi"() -> ("Application Directory"=w506:path)
        n198 = Build Path(base path=w506, name or relative path="Sound\\demo_cough.wav" ("path")) -> (appended path=w504:path)
        n199 = local read "number of samples/ch"() -> (w518:i32)
        n200 = call-poly <vilib>:"Sound File Info.vi"("path"=w504) -> ("error out"=w511:errorcluster, "sound format"=w510:T6, "path out"=w512:path)  [unwired: 7 in, 1 out]
        n201 = call-poly <vilib>:"Sound File Open.vi"("error in (no error)"=w511, "path"=w512) -> ("error out"=w508:errorcluster, "sound file refnum"=w515:T7)  [unwired: 8 in]
        n202 = call <vilib>:"Sound Output Configure.vi"("number of samples/ch"=w518, "sample mode"=w507, "error in (no error)"=w508, "sound format"=w510, "device ID"=u32 0) -> ("error out"=w516:errorcluster, "task ID"=w514:T8)  [unwired: 5 in]
        n203 = while {
          tunnel: w514 -> [w528]
          tunnel: [w527] -> w513
          tunnel: w515 -> [w523]
          tunnel: w516 -> [w522]
          tunnel: w518 -> [w524]
          tunnel: [w526] -> w517
          stop <- w520 stop-if-true
          n204 = local read "Play/Stop"() -> (w519:bool)
          n205 = Wait (ms)(milliseconds to wait=u32 50) -> ()  [unwired: 1 out]
          n206 = case shown="False" w519 {
            selector: w519 -> [w533 w551]
            tunnel: w528 -> [w536 w548]
            tunnel: [w534 w550] -> w527
            tunnel: [w535 w549] -> _
            tunnel: [w533 w551] -> _
            tunnel: [w531 w545] -> w526
            tunnel: w524 -> [_ w542]
            tunnel: w523 -> [w531 w541]
            tunnel: w522 -> [w532 w540]
            tunnel: "Demo cough" -> [_ w539]
            tunnel: [TRUE FALSE] -> w520
            frame False {
              w530 = T1 0 items=["Absolute"=0, "Relative"=2] ("position mode")
              n207 = call <vilib>:"Sound Output Stop.vi"("error in (no error)"=w532, "task ID"=w536) -> ("error out"=w534:errorcluster, "task ID out"=w535:T8)  [unwired: 8 in]
              n208 = local write "Demo cough"(w530) -> ()
            }
            frame True {
              w538 = T1 2 items=["Absolute"=0, "Relative"=2] ("position mode")
              n209 = call-poly <vilib>:"Sound File Read.vi"("number of samples/ch (-1: all)"=w542, "error in (no error)"=w540, "position mode"=w539, "sound file refnum"=w541) -> ("error out"=w544:errorcluster, "data"=w543:waveform(dbl)[], "sound file refnum out"=w545:T7)  [unwired: 3 in, 2 out]
              n210 = local write "Demo cough"(w538) -> ()
              n211 = call-poly <vilib>:"Sound Output Write.vi"("error in (no error)"=w544, "data"=w543, "task ID"=w548) -> ("error out"=w546:errorcluster, "task ID out"=w547:T8)  [unwired: 7 in]
              n212 = call <vilib>:"Sound Output Start.vi"("error in (no error)"=w546, "task ID"=w547) -> ("error out"=w550:errorcluster, "task ID out"=w549:T8)  [unwired: 8 in]
            }
          }
        }
        n213 = call <vilib>:"Sound File Close.vi"("error in (no error)"=w513, "sound file refnum"=w517) -> ()  [unwired: 9 in, 1 out]
      }
      frame 6 {
        w566 = T5 1 items=["Finite Samples", "Continuous Samples"] ("sample mode")
        n214 = call <vilib>:"Application Directory.vi"() -> ("Application Directory"=w554:path)
        n215 = Build Path(base path=w554, name or relative path="Sound\\demo_abdBreathing.wav" ("path")) -> (appended path=w552:path)
        n216 = local read "number of samples/ch"() -> (w555:i32)
        n217 = call-poly <vilib>:"Sound File Info.vi"("path"=w552) -> ("error out"=w562:errorcluster, "sound format"=w563:T6, "path out"=w561:path)  [unwired: 7 in, 1 out]
        n218 = call-poly <vilib>:"Sound File Open.vi"("error in (no error)"=w562, "path"=w561) -> ("error out"=w565:errorcluster, "sound file refnum"=w558:T7)  [unwired: 8 in]
        n219 = call <vilib>:"Sound Output Configure.vi"("number of samples/ch"=w555, "sample mode"=w566, "error in (no error)"=w565, "sound format"=w563, "device ID"=u32 0) -> ("error out"=w557:errorcluster, "task ID"=w559:T8)  [unwired: 5 in]
        n220 = while {
          tunnel: w559 -> [w576]
          tunnel: [w575] -> w560
          tunnel: w558 -> [w571]
          tunnel: w557 -> [w570]
          tunnel: w555 -> [w572]
          tunnel: [w574] -> w556
          stop <- w567 stop-if-true
          n221 = local read "Play/Stop"() -> (w568:bool)
          n222 = Wait (ms)(milliseconds to wait=u32 50) -> ()  [unwired: 1 out]
          n223 = case shown="False" w568 {
            selector: w568 -> [w581 w599]
            tunnel: w576 -> [w584 w596]
            tunnel: [w582 w598] -> w575
            tunnel: [w583 w597] -> _
            tunnel: [w581 w599] -> _
            tunnel: [w579 w593] -> w574
            tunnel: w572 -> [_ w590]
            tunnel: w571 -> [w579 w589]
            tunnel: w570 -> [w580 w588]
            tunnel: "Demo abdomen" -> [_ w587]
            tunnel: [TRUE FALSE] -> w567
            frame False {
              w578 = T1 0 items=["Absolute"=0, "Relative"=2] ("position mode")
              n224 = call <vilib>:"Sound Output Stop.vi"("error in (no error)"=w580, "task ID"=w584) -> ("error out"=w582:errorcluster, "task ID out"=w583:T8)  [unwired: 8 in]
              n225 = local write "Demo abdomen"(w578) -> ()
            }
            frame True {
              w586 = T1 2 items=["Absolute"=0, "Relative"=2] ("position mode")
              n226 = call-poly <vilib>:"Sound File Read.vi"("number of samples/ch (-1: all)"=w590, "error in (no error)"=w588, "position mode"=w587, "sound file refnum"=w589) -> ("error out"=w592:errorcluster, "data"=w591:waveform(dbl)[], "sound file refnum out"=w593:T7)  [unwired: 3 in, 2 out]
              n227 = local write "Demo abdomen"(w586) -> ()
              n228 = call-poly <vilib>:"Sound Output Write.vi"("error in (no error)"=w592, "data"=w591, "task ID"=w596) -> ("error out"=w594:errorcluster, "task ID out"=w595:T8)  [unwired: 7 in]
              n229 = call <vilib>:"Sound Output Start.vi"("error in (no error)"=w594, "task ID"=w595) -> ("error out"=w598:errorcluster, "task ID out"=w597:T8)  [unwired: 8 in]
            }
          }
        }
        n230 = call <vilib>:"Sound File Close.vi"("error in (no error)"=w560, "sound file refnum"=w556) -> ()  [unwired: 9 in, 1 out]
      }
      frame 7 {
        w603 = T5 1 items=["Finite Samples", "Continuous Samples"] ("sample mode")
        n231 = call <vilib>:"Application Directory.vi"() -> ("Application Directory"=w602:path)
        n232 = Build Path(base path=w602, name or relative path="Sound\\calibInstr3.wav" ("path")) -> (appended path=w600:path)
        n233 = call-poly <vilib>:"Sound File Info.vi"("path"=w600) -> ("error out"=w607:errorcluster, "sound format"=w606:T6, "path out"=w608:path)  [unwired: 7 in, 1 out]
        n234 = call-poly <vilib>:"Sound File Open.vi"("error in (no error)"=w607, "path"=w608) -> ("error out"=w604:errorcluster, "sound file refnum"=w611:T7)  [unwired: 8 in]
        n235 = call <vilib>:"Sound Output Configure.vi"("number of samples/ch"="number of samples/ch", "sample mode"=w603, "error in (no error)"=w604, "sound format"=w606, "device ID"=u32 0) -> ("error out"=w612:errorcluster, "task ID"=w610:T8)  [unwired: 5 in]
        n236 = while {
          tunnel: w610 -> [w624]
          tunnel: [w623] -> w609
          tunnel: w611 -> [w619]
          tunnel: w612 -> [w618]
          tunnel: "number of samples/ch" -> [w620]
          tunnel: [w622] -> w613
          stop <- w615 stop-if-true
          n237 = local read "Play/Stop"() -> (w616:bool)
          n238 = Wait (ms)(milliseconds to wait=u32 50) -> ()  [unwired: 1 out]
          n239 = case shown="True" w616 {
            selector: w616 -> [w629 w647]
            tunnel: w624 -> [w632 w644]
            tunnel: [w630 w646] -> w623
            tunnel: [w631 w645] -> _
            tunnel: [w629 w647] -> _
            tunnel: [w627 w641] -> w622
            tunnel: w620 -> [_ w638]
            tunnel: w619 -> [w627 w637]
            tunnel: w618 -> [w628 w636]
            tunnel: "Calibration" -> [_ w635]
            tunnel: [TRUE FALSE] -> w615
            frame False {
              w626 = T1 0 items=["Absolute"=0, "Relative"=2] ("position mode")
              n240 = call <vilib>:"Sound Output Stop.vi"("error in (no error)"=w628, "task ID"=w632) -> ("error out"=w630:errorcluster, "task ID out"=w631:T8)  [unwired: 8 in]
              n241 = local write "Calibration"(w626) -> ()
            }
            frame True {
              w634 = T1 2 items=["Absolute"=0, "Relative"=2] ("position mode")
              n242 = call-poly <vilib>:"Sound File Read.vi"("number of samples/ch (-1: all)"=w638, "error in (no error)"=w636, "position mode"=w635, "sound file refnum"=w637) -> ("error out"=w640:errorcluster, "data"=w639:waveform(dbl)[], "sound file refnum out"=w641:T7)  [unwired: 3 in, 2 out]
              n243 = local write "Calibration"(w634) -> ()
              n244 = call-poly <vilib>:"Sound Output Write.vi"("error in (no error)"=w640, "data"=w639, "task ID"=w644) -> ("error out"=w642:errorcluster, "task ID out"=w643:T8)  [unwired: 7 in]
              n245 = call <vilib>:"Sound Output Start.vi"("error in (no error)"=w642, "task ID"=w643) -> ("error out"=w646:errorcluster, "task ID out"=w645:T8)  [unwired: 8 in]
            }
          }
        }
        n246 = call <vilib>:"Sound File Close.vi"("error in (no error)"=w609, "sound file refnum"=w613) -> ()  [unwired: 9 in, 1 out]
      }
      frame 8 {
        w651 = T5 1 items=["Finite Samples", "Continuous Samples"] ("sample mode")
        n247 = call <vilib>:"Application Directory.vi"() -> ("Application Directory"=w649:path)
        n248 = Build Path(base path=w649, name or relative path="Sound\\NCS_massStudy_Instr_v3b_routine1.wav" ("path")) -> (appended path=w650:path)
        n249 = local read "number of samples/ch"() -> (w662:i32)
        n250 = call-poly <vilib>:"Sound File Info.vi"("path"=w650) -> ("error out"=w655:errorcluster, "sound format"=w654:T6, "path out"=w656:path)  [unwired: 7 in, 1 out]
        n251 = call-poly <vilib>:"Sound File Open.vi"("error in (no error)"=w655, "path"=w656) -> ("error out"=w652:errorcluster, "sound file refnum"=w659:T7)  [unwired: 8 in]
        n252 = call <vilib>:"Sound Output Configure.vi"("number of samples/ch"=w662, "sample mode"=w651, "error in (no error)"=w652, "sound format"=w654, "device ID"=u32 0) -> ("error out"=w660:errorcluster, "task ID"=w658:T8)  [unwired: 5 in]
        n253 = while {
          tunnel: w658 -> [w672]
          tunnel: [w671] -> w657
          tunnel: w659 -> [w667]
          tunnel: w660 -> [w666]
          tunnel: w662 -> [w668]
          tunnel: [w670] -> w661
          stop <- w663 stop-if-true
          n254 = local read "Play/Stop"() -> (w664:bool)
          n255 = Wait (ms)(milliseconds to wait=u32 50) -> ()  [unwired: 1 out]
          n256 = case shown="False" w664 {
            selector: w664 -> [w677 w695]
            tunnel: w672 -> [w680 w692]
            tunnel: [w678 w694] -> w671
            tunnel: [w679 w693] -> _
            tunnel: [w677 w695] -> _
            tunnel: [w675 w689] -> w670
            tunnel: w668 -> [_ w686]
            tunnel: w667 -> [w675 w685]
            tunnel: w666 -> [w676 w684]
            tunnel: "Routine 1" -> [_ w683]
            tunnel: [TRUE FALSE] -> w663
            frame False {
              w674 = T1 0 items=["Absolute"=0, "Relative"=2] ("position mode")
              n257 = call <vilib>:"Sound Output Stop.vi"("error in (no error)"=w676, "task ID"=w680) -> ("error out"=w678:errorcluster, "task ID out"=w679:T8)  [unwired: 8 in]
              n258 = local write "Routine 1"(w674) -> ()
            }
            frame True {
              w682 = T1 2 items=["Absolute"=0, "Relative"=2] ("position mode")
              n259 = call-poly <vilib>:"Sound File Read.vi"("number of samples/ch (-1: all)"=w686, "error in (no error)"=w684, "position mode"=w683, "sound file refnum"=w685) -> ("error out"=w688:errorcluster, "data"=w687:waveform(dbl)[], "sound file refnum out"=w689:T7)  [unwired: 3 in, 2 out]
              n260 = local write "Routine 1"(w682) -> ()
              n261 = call-poly <vilib>:"Sound Output Write.vi"("error in (no error)"=w688, "data"=w687, "task ID"=w692) -> ("error out"=w690:errorcluster, "task ID out"=w691:T8)  [unwired: 7 in]
              n262 = call <vilib>:"Sound Output Start.vi"("error in (no error)"=w690, "task ID"=w691) -> ("error out"=w694:errorcluster, "task ID out"=w693:T8)  [unwired: 8 in]
            }
          }
        }
        n263 = call <vilib>:"Sound File Close.vi"("error in (no error)"=w657, "sound file refnum"=w661) -> ()  [unwired: 9 in, 1 out]
      }
      frame 9 {
        w699 = T5 1 items=["Finite Samples", "Continuous Samples"] ("sample mode")
        n264 = call <vilib>:"Application Directory.vi"() -> ("Application Directory"=w698:path)
        n265 = Build Path(base path=w698, name or relative path="Sound\\calmMusic3.wav" ("path")) -> (appended path=w696:path)
        n266 = local read "number of samples/ch"() -> (w710:i32)
        n267 = call-poly <vilib>:"Sound File Info.vi"("path"=w696) -> ("error out"=w703:errorcluster, "sound format"=w702:T6, "path out"=w704:path)  [unwired: 7 in, 1 out]
        n268 = call-poly <vilib>:"Sound File Open.vi"("error in (no error)"=w703, "path"=w704) -> ("error out"=w700:errorcluster, "sound file refnum"=w707:T7)  [unwired: 8 in]
        n269 = call <vilib>:"Sound Output Configure.vi"("number of samples/ch"=w710, "sample mode"=w699, "error in (no error)"=w700, "sound format"=w702, "device ID"=u32 0) -> ("error out"=w708:errorcluster, "task ID"=w706:T8)  [unwired: 5 in]
        n270 = while {
          tunnel: w706 -> [w720]
          tunnel: [w719] -> w705
          tunnel: w707 -> [w715]
          tunnel: w708 -> [w714]
          tunnel: w710 -> [w716]
          tunnel: [w718] -> w709
          stop <- w711 stop-if-true
          n271 = local read "Play/Stop"() -> (w712:bool)
          n272 = Wait (ms)(milliseconds to wait=u32 50) -> ()  [unwired: 1 out]
          n273 = case shown="False" w712 {
            selector: w712 -> [w725 w743]
            tunnel: w720 -> [w728 w740]
            tunnel: [w726 w742] -> w719
            tunnel: [w727 w741] -> _
            tunnel: [w725 w743] -> _
            tunnel: [w723 w737] -> w718
            tunnel: w716 -> [_ w734]
            tunnel: w715 -> [w723 w733]
            tunnel: w714 -> [w724 w732]
            tunnel: "(2a) Calm Music" -> [_ w731]
            tunnel: [TRUE FALSE] -> w711
            frame False {
              w722 = T1 0 items=["Absolute"=0, "Relative"=2] ("position mode")
              n274 = call <vilib>:"Sound Output Stop.vi"("error in (no error)"=w724, "task ID"=w728) -> ("error out"=w726:errorcluster, "task ID out"=w727:T8)  [unwired: 8 in]
              n275 = local write "(2a) Calm Music"(w722) -> ()
            }
            frame True {
              w730 = T1 2 items=["Absolute"=0, "Relative"=2] ("position mode")
              n276 = call-poly <vilib>:"Sound File Read.vi"("number of samples/ch (-1: all)"=w734, "error in (no error)"=w732, "position mode"=w731, "sound file refnum"=w733) -> ("error out"=w736:errorcluster, "data"=w735:waveform(dbl)[], "sound file refnum out"=w737:T7)  [unwired: 3 in, 2 out]
              n277 = local write "(2a) Calm Music"(w730) -> ()
              n278 = call-poly <vilib>:"Sound Output Write.vi"("error in (no error)"=w736, "data"=w735, "task ID"=w740) -> ("error out"=w738:errorcluster, "task ID out"=w739:T8)  [unwired: 7 in]
              n279 = call <vilib>:"Sound Output Start.vi"("error in (no error)"=w738, "task ID"=w739) -> ("error out"=w742:errorcluster, "task ID out"=w741:T8)  [unwired: 8 in]
            }
          }
        }
        n280 = call <vilib>:"Sound File Close.vi"("error in (no error)"=w705, "sound file refnum"=w709) -> ()  [unwired: 9 in, 1 out]
      }
      frame 10 {
        w758 = T5 1 items=["Finite Samples", "Continuous Samples"] ("sample mode")
        n281 = call <vilib>:"Application Directory.vi"() -> ("Application Directory"=w746:path)
        n282 = Build Path(base path=w746, name or relative path="Sound\\attentionTestInstr.wav" ("path")) -> (appended path=w745:path)
        n283 = local read "number of samples/ch"() -> (w747:i32)
        n284 = call-poly <vilib>:"Sound File Info.vi"("path"=w745) -> ("error out"=w754:errorcluster, "sound format"=w755:T6, "path out"=w753:path)  [unwired: 7 in, 1 out]
        n285 = call-poly <vilib>:"Sound File Open.vi"("error in (no error)"=w754, "path"=w753) -> ("error out"=w757:errorcluster, "sound file refnum"=w750:T7)  [unwired: 8 in]
        n286 = call <vilib>:"Sound Output Configure.vi"("number of samples/ch"=w747, "sample mode"=w758, "error in (no error)"=w757, "sound format"=w755, "device ID"=u32 0) -> ("error out"=w749:errorcluster, "task ID"=w751:T8)  [unwired: 5 in]
        n287 = while {
          tunnel: w751 -> [w768]
          tunnel: [w767] -> w752
          tunnel: w750 -> [w763]
          tunnel: w749 -> [w762]
          tunnel: w747 -> [w764]
          tunnel: [w766] -> w748
          stop <- w759 stop-if-true
          n288 = local read "Play/Stop"() -> (w760:bool)
          n289 = Wait (ms)(milliseconds to wait=u32 50) -> ()  [unwired: 1 out]
          n290 = case shown="False" w760 {
            selector: w760 -> [w773 w791]
            tunnel: w768 -> [w776 w788]
            tunnel: [w774 w790] -> w767
            tunnel: [w775 w789] -> _
            tunnel: [w773 w791] -> _
            tunnel: [w771 w785] -> w766
            tunnel: w764 -> [_ w782]
            tunnel: w763 -> [w771 w781]
            tunnel: w762 -> [w772 w780]
            tunnel: "(2b) Attn Test" -> [_ w779]
            tunnel: [TRUE FALSE] -> w759
            frame False {
              w770 = T1 0 items=["Absolute"=0, "Relative"=2] ("position mode")
              n291 = call <vilib>:"Sound Output Stop.vi"("error in (no error)"=w772, "task ID"=w776) -> ("error out"=w774:errorcluster, "task ID out"=w775:T8)  [unwired: 8 in]
              n292 = local write "(2b) Attn Test"(w770) -> ()
            }
            frame True {
              w778 = T1 2 items=["Absolute"=0, "Relative"=2] ("position mode")
              n293 = call-poly <vilib>:"Sound File Read.vi"("number of samples/ch (-1: all)"=w782, "error in (no error)"=w780, "position mode"=w779, "sound file refnum"=w781) -> ("error out"=w784:errorcluster, "data"=w783:waveform(dbl)[], "sound file refnum out"=w785:T7)  [unwired: 3 in, 2 out]
              n294 = local write "(2b) Attn Test"(w778) -> ()
              n295 = call-poly <vilib>:"Sound Output Write.vi"("error in (no error)"=w784, "data"=w783, "task ID"=w788) -> ("error out"=w786:errorcluster, "task ID out"=w787:T8)  [unwired: 7 in]
              n296 = call <vilib>:"Sound Output Start.vi"("error in (no error)"=w786, "task ID"=w787) -> ("error out"=w790:errorcluster, "task ID out"=w789:T8)  [unwired: 8 in]
            }
          }
        }
        n297 = call <vilib>:"Sound File Close.vi"("error in (no error)"=w752, "sound file refnum"=w748) -> ()  [unwired: 9 in, 1 out]
      }
      frame 11 {
        w806 = T5 1 items=["Finite Samples", "Continuous Samples"] ("sample mode")
        n298 = call <vilib>:"Application Directory.vi"() -> ("Application Directory"=w794:path)
        n299 = Build Path(base path=w794, name or relative path="Sound\\NCS_massStudy_Instr_v3_routine3_4.wav" ("path")) -> (appended path=w792:path)
        n300 = local read "number of samples/ch"() -> (w795:i32)
        n301 = call-poly <vilib>:"Sound File Info.vi"("path"=w792) -> ("error out"=w802:errorcluster, "sound format"=w803:T6, "path out"=w801:path)  [unwired: 7 in, 1 out]
        n302 = call-poly <vilib>:"Sound File Open.vi"("error in (no error)"=w802, "path"=w801) -> ("error out"=w805:errorcluster, "sound file refnum"=w798:T7)  [unwired: 8 in]
        n303 = call <vilib>:"Sound Output Configure.vi"("number of samples/ch"=w795, "sample mode"=w806, "error in (no error)"=w805, "sound format"=w803, "device ID"=u32 0) -> ("error out"=w797:errorcluster, "task ID"=w799:T8)  [unwired: 5 in]
        n304 = while {
          tunnel: w799 -> [w816]
          tunnel: [w815] -> w800
          tunnel: w798 -> [w811]
          tunnel: w797 -> [w810]
          tunnel: w795 -> [w812]
          tunnel: [w814] -> w796
          stop <- w807 stop-if-true
          n305 = local read "Play/Stop"() -> (w808:bool)
          n306 = Wait (ms)(milliseconds to wait=u32 50) -> ()  [unwired: 1 out]
          n307 = case shown="False" w808 {
            selector: w808 -> [w821 w839]
            tunnel: w816 -> [w824 w836]
            tunnel: [w822 w838] -> w815
            tunnel: [w823 w837] -> _
            tunnel: [w821 w839] -> _
            tunnel: [w819 w833] -> w814
            tunnel: w812 -> [_ w830]
            tunnel: w811 -> [w819 w829]
            tunnel: w810 -> [w820 w828]
            tunnel: "Routine 3,4" -> [_ w827]
            tunnel: [TRUE FALSE] -> w807
            frame False {
              w818 = T1 0 items=["Absolute"=0, "Relative"=2] ("position mode")
              n308 = call <vilib>:"Sound Output Stop.vi"("error in (no error)"=w820, "task ID"=w824) -> ("error out"=w822:errorcluster, "task ID out"=w823:T8)  [unwired: 8 in]
              n309 = local write "Routine 3,4"(w818) -> ()
            }
            frame True {
              w826 = T1 2 items=["Absolute"=0, "Relative"=2] ("position mode")
              n310 = call-poly <vilib>:"Sound File Read.vi"("number of samples/ch (-1: all)"=w830, "error in (no error)"=w828, "position mode"=w827, "sound file refnum"=w829) -> ("error out"=w832:errorcluster, "data"=w831:waveform(dbl)[], "sound file refnum out"=w833:T7)  [unwired: 3 in, 2 out]
              n311 = local write "Routine 3,4"(w826) -> ()
              n312 = call-poly <vilib>:"Sound Output Write.vi"("error in (no error)"=w832, "data"=w831, "task ID"=w836) -> ("error out"=w834:errorcluster, "task ID out"=w835:T8)  [unwired: 7 in]
              n313 = call <vilib>:"Sound Output Start.vi"("error in (no error)"=w834, "task ID"=w835) -> ("error out"=w838:errorcluster, "task ID out"=w837:T8)  [unwired: 8 in]
            }
          }
        }
        n314 = call <vilib>:"Sound File Close.vi"("error in (no error)"=w800, "sound file refnum"=w796) -> ()  [unwired: 9 in, 1 out]
      }
      frame 12 {
        w844 = T5 1 items=["Finite Samples", "Continuous Samples"] ("sample mode")
        n315 = call <vilib>:"Application Directory.vi"() -> ("Application Directory"=w842:path)
        n316 = Build Path(base path=w842, name or relative path="Sound\\NCS_massStudy_Instr_v3_routine5.wav" ("path")) -> (appended path=w840:path)
        n317 = local read "number of samples/ch"() -> (w843:i32)
        n318 = call-poly <vilib>:"Sound File Info.vi"("path"=w840) -> ("error out"=w848:errorcluster, "sound format"=w847:T6, "path out"=w849:path)  [unwired: 7 in, 1 out]
        n319 = call-poly <vilib>:"Sound File Open.vi"("error in (no error)"=w848, "path"=w849) -> ("error out"=w845:errorcluster, "sound file refnum"=w852:T7)  [unwired: 8 in]
        n320 = call <vilib>:"Sound Output Configure.vi"("number of samples/ch"=w843, "sample mode"=w844, "error in (no error)"=w845, "sound format"=w847, "device ID"=u32 0) -> ("error out"=w853:errorcluster, "task ID"=w851:T8)  [unwired: 5 in]
        n321 = while {
          tunnel: w851 -> [w864]
          tunnel: [w863] -> w850
          tunnel: w852 -> [w859]
          tunnel: w853 -> [w858]
          tunnel: w843 -> [w860]
          tunnel: [w862] -> w854
          stop <- w855 stop-if-true
          n322 = local read "Play/Stop"() -> (w856:bool)
          n323 = Wait (ms)(milliseconds to wait=u32 50) -> ()  [unwired: 1 out]
          n324 = case shown="False" w856 {
            selector: w856 -> [w869 w887]
            tunnel: w864 -> [w872 w884]
            tunnel: [w870 w886] -> w863
            tunnel: [w871 w885] -> _
            tunnel: [w869 w887] -> _
            tunnel: [w867 w881] -> w862
            tunnel: w860 -> [_ w878]
            tunnel: w859 -> [w867 w877]
            tunnel: w858 -> [w868 w876]
            tunnel: "Routine 5" -> [_ w875]
            tunnel: [TRUE FALSE] -> w855
            frame False {
              w866 = T1 0 items=["Absolute"=0, "Relative"=2] ("position mode")
              n325 = call <vilib>:"Sound Output Stop.vi"("error in (no error)"=w868, "task ID"=w872) -> ("error out"=w870:errorcluster, "task ID out"=w871:T8)  [unwired: 8 in]
              n326 = local write "Routine 5"(w866) -> ()
            }
            frame True {
              w874 = T1 2 items=["Absolute"=0, "Relative"=2] ("position mode")
              n327 = call-poly <vilib>:"Sound File Read.vi"("number of samples/ch (-1: all)"=w878, "error in (no error)"=w876, "position mode"=w875, "sound file refnum"=w877) -> ("error out"=w880:errorcluster, "data"=w879:waveform(dbl)[], "sound file refnum out"=w881:T7)  [unwired: 3 in, 2 out]
              n328 = local write "Routine 5"(w874) -> ()
              n329 = call-poly <vilib>:"Sound Output Write.vi"("error in (no error)"=w880, "data"=w879, "task ID"=w884) -> ("error out"=w882:errorcluster, "task ID out"=w883:T8)  [unwired: 7 in]
              n330 = call <vilib>:"Sound Output Start.vi"("error in (no error)"=w882, "task ID"=w883) -> ("error out"=w886:errorcluster, "task ID out"=w885:T8)  [unwired: 8 in]
            }
          }
        }
        n331 = call <vilib>:"Sound File Close.vi"("error in (no error)"=w850, "sound file refnum"=w854) -> ()  [unwired: 9 in, 1 out]
      }
    }
  }
  n332 = call <instrlib>:"niUSRP Close Session.vi"("session handle"=w140, "error in (no error)"=w145) -> ("error out"=w137:errorcluster)  [unwired: 13 in]
  n333 = flat-sequence {
    tunnel: w138 -> [w890]
    tunnel: w137 -> [w889]
    tunnel: [w888] -> w76
    frame #0 {
      n334 = Merge Errors(w890, w889) -> (w888:errorcluster)
      n335 = local write "Stop"(FALSE ("STOP")) -> ()
    }
  }
  n336 = call <instrlib>:"niUSRP Close Session.vi"("session handle"=w4, "error in (no error)"=w3) -> ("error out"=w2:errorcluster)  [unwired: 13 in]
  n337 = local read "Rx IQ Rate"() -> (w107:dbl)
  n338 = Divide(x=2000.0, y=2.0) -> (x/y=→"BW/2":dbl)
  n339 = local read "Waveform Size"() -> (w119:dbl)
  n340 = Divide(x=w107, y="DownSamplingRatio") -> (x/y=→"Sampling Rate":dbl)
  n341 = Divide(x=w119, y="DownSamplingRatio") -> (x/y=w102:dbl)
  n342 = Initialize Array(0.0 ("element"), w103, w102) -> (w120:dbl[][])
  n343 = Initialize Array(0.0 ("element"), w103, w102) -> (w109:dbl[][])
  n344 = Obtain Queue "Display Queue"(name (unnamed)="DispQueue", element data type=w120) -> (queue out=w89:refnum<queue>)  [unwired: 3 in, 2 out]
  n345 = Obtain Queue "Saving Queue"(name (unnamed)="SaveBuffer", element data type=w109) -> (queue out=w108:refnum<queue>)  [unwired: 3 in, 2 out]
  n346 = local read "Rx IQ Rate"() -> (w72:dbl)
  n347 = local read "SDR1 \nTone Frequency"() -> (w97:dbl)
  n348 = local read "DownSamplingRatio"() -> (w65:i32)
  n349 = local read "Waveform Size"() -> (w74:dbl)
  n350 = local read "Waveform Size"() -> (w66:dbl)
  n351 = Divide(x=w66, y=w65) -> (x/y=w64:dbl)
  n352 = local read "SDR2\nTone Frequency"() -> (w73:dbl)
  n353 = Initialize Array(0.0 ("element"), 2 ("dimension size"), w64) -> (w69:dbl[][])
  n354 = Obtain Queue(max queue size (-1, unlimited)=-1, name (unnamed)="Rx2DS_Queue", element data type=w69) -> (queue out=w62:refnum<queue>)  [unwired: 2 in, 2 out]
  n355 = while {
    tunnel: w91 -> [w936]
    tunnel: w108 -> [w925]
    tunnel: w74 -> [w920]
    tunnel: w97 -> [w907]
    tunnel: w72 -> [w919]
    tunnel: w89 -> [w906]
    tunnel: w62 -> [w899]
    stop <- FALSE stop-if-true
    # "The order is changed to amp1 - amp2 - ph1 - ph2"
    # "Downsampling the NCS signal"
    # "Getting the amplitude and phase from I and Q"
    # "Rx 1 - Tx 1"
    # "Tx1 to Rx1 QueInd_0"
    # "100 times"
    n356 = call "NCS_IQ_OneTx.vi"("Coerced IQ rate"=w919, "Waveform Size"=w920, "Channel 0\nTone Frequency"=w907, "Channel 0\nTone Amplitude"=1) -> ("IQ waveform array"=w897:cdb[])  [unwired: 4 in, 2 out]
    n357 = Dequeue Element(queue=w936) -> (element=w905:cdb[])  [unwired: 2 in, 3 out]
    n358 = Get Queue Status(queue=w936) -> (# elements in queue=→"# queue 1":i32)  [unwired: 2 in, 7 out]
    n359 = local read "SDR1 \nTone Frequency"() -> (w933:dbl)
    n360 = local read "BW/2"() -> (w928:dbl)
    n361 = local read "Rx IQ Rate"() -> (w924:dbl)
    n362 = Get Queue Status(queue=w899) -> (queue out=w898:refnum<queue>, # elements in queue=→"# Rx2DS_Queue":i32)  [unwired: 2 in, 6 out]
    n363 = case shown="True" "Flush Rx2" {
      tunnel: [w943 w946] -> w895
      tunnel: [w941 w946] -> w894
      tunnel: w898 -> [w940 w951]
      tunnel: ["Dequeing Rx2" "Flushing Rx2"] -> w893
      frame False {
        n364 = Dequeue Element(queue=w940) -> (element=w939:dbl[][])  [unwired: 2 in, 3 out]
        "element" <- w939
        n365 = Index Array(array=w939, index (row)=0 ("index")) -> (element=w943:dbl[])  [unwired: 1 in]
        n366 = Index Array(array=w939, index (row)=1) -> (element=w941:dbl[])  [unwired: 1 in]
      }
      frame True {
        n367 = Flush Queue(queue=w951) -> ()  [unwired: 1 in, 3 out]
        n368 = local read "DownSamplingRatio"() -> (w948:i32)
        n369 = local read "Waveform Size"() -> (w949:dbl)
        n370 = Divide(x=w949, y=w948) -> (x/y=w947:dbl)
        n371 = Initialize Array(0.0, w947) -> (w946:dbl[])
      }
    }
    "String 3" <- w893
    n372 = Subtract(x=w933, y=w928) -> (x-y=w934:dbl)
    n373 = Add(x=w933, y=w928) -> (x+y=w935:dbl)
    n374 = Complex To Polar(r * e^(i*theta)=w897) -> (theta=w916:dbl[])  [unwired: 1 out]
    n375 = call-poly <vilib>:"Butterworth Filter.vi"("init/cont (init:F)"=TRUE, "order"=2, "filter type"=Filter_Passband_Type."Bandpass", "low cutoff freq: fl"=w934, "high cutoff freq: fh"=w935, "sampling freq: fs"=w924, "X"=w905) -> ("Filtered X"=w930:cdb[])  [unwired: 1 in, 1 out]
    n376 = Complex To Polar(r * e^(i*theta)=w930) -> (r=w927:dbl[], theta=w915:dbl[])
    n377 = Subtract(x=w915, y=w916) -> (x-y=w918:dbl[])
    n378 = call <vilib>:"Unwrap Phase.vi"("phase unit"=1 ("y"), "Phase"=w918) -> ("Unwrapped Phase"=w913:dbl[])  [unwired: 8 in, 1 out]
    n379 = local read "DownSamplingRatio"() -> (w909:i32)
    n380 = local read "Waveform Size"() -> (w923:dbl)
    n381 = Divide(x=w923, y=w909) -> (x/y=w912:dbl)
    n382 = Reshape Array(w927, w912, w909) -> (w914:dbl[][])
    n383 = Reshape Array(w913, w912, w909) -> (w911:dbl[][])
    n384 = for {
      tunnel: w914 -> [w964] mode=indexing
      tunnel: [w963] -> w926 mode=indexing
      tunnel: w911 -> [w962] mode=indexing
      tunnel: [w961] -> w910 mode=indexing
      n385 = Add Array Elements(numeric array=w964) -> (sum=w963:dbl)
      n386 = Add Array Elements(numeric array=w962) -> (sum=w961:dbl)
    }
    n387 = Divide(x=w926, y=w909) -> (x/y=w903:dbl[])
    n388 = Divide(x=w910, y=w909) -> (x/y=w902:dbl[])
    n389 = Build Array(w903, w895, w902, w894) -> (w904:dbl[][])
    n390 = disable-structure shown="Enabled" {
      disable-tunnel: w903 -> [w955 _]
      disable-tunnel: w902 -> [w954 _]
      disable-tunnel: w895 -> [w953 _]
      disable-tunnel: w894 -> [w952 _]
      frame Disabled {
        "Amp1 @50 kHz" <- w955
        "Ph1 @50 kHz" <- w954
        "Ph2 @50 kHz" <- w952
        "Amp2 @50 kHz" <- w953
      }
      frame Enabled {
      }
    }
    n391 = Array Size(array=w904) -> (size(s)=→"ArraySz":i32[])
    n392 = local read "Flush"() -> (w921:bool)
    n393 = local read "Buffer"() -> (w922:bool)
    n394 = Enqueue Element(queue=w906, element=w904) -> ()  [unwired: 2 in, 3 out]
    n395 = case shown="True" w922 {
      tunnel: w925 -> [w957 w960]
      tunnel: w904 -> [_ w959]
      tunnel: w921 -> [w956 _]
      frame False {
        n396 = case shown="False" w956 {
          tunnel: w957 -> [_ w958]
          frame False {
          }
          frame True {
            n397 = Flush Queue(queue=w958) -> ()  [unwired: 1 in, 3 out]
          }
        }
      }
      frame True {
        n398 = Enqueue Element(queue=w960, element=w959) -> ()  [unwired: 2 in, 3 out]
      }
    }
  }
  n399 = while {
    tunnel: w74 -> [w980]
    tunnel: w73 -> [w978]
    tunnel: w72 -> [w977]
    tunnel: w71 -> [w971]
    shift-right: [w969] -> _
    shift-left: w62 -> [w974]
    stop <- FALSE stop-if-true
    # "Rx 2 - Tx 2"
    # "Tx2 to Rx2 QueInd_0"
    # "100 times"
    n400 = call "NCS_IQ_OneTx.vi"("Coerced IQ rate"=w977, "Waveform Size"=w980, "Channel 0\nTone Frequency"=w978, "Channel 0\nTone Amplitude"=1) -> ("IQ waveform array"=w968:cdb[])  [unwired: 4 in, 2 out]
    n401 = Get Queue Status(queue=w971) -> (# elements in queue=→"#queue 3":i32)  [unwired: 2 in, 7 out]
    n402 = Dequeue Element(queue=w971) -> (element=w1003:cdb[])  [unwired: 2 in, 3 out]
    n403 = local read "SDR2\nTone Frequency"() -> (w983:dbl)
    n404 = local read "BW/2"() -> (w988:dbl)
    n405 = local read "Rx IQ Rate"() -> (w991:dbl)
    n406 = Subtract(x=w983, y=w988) -> (x-y=w982:dbl)
    n407 = Add(x=w983, y=w988) -> (x+y=w981:dbl)
    n408 = Complex To Polar(r * e^(i*theta)=w968) -> (theta=w995:dbl[])  [unwired: 1 out]
    n409 = call-poly <vilib>:"Butterworth Filter.vi"("init/cont (init:F)"=TRUE, "order"=2, "filter type"=Filter_Passband_Type."Bandpass", "low cutoff freq: fl"=w982, "high cutoff freq: fh"=w981, "sampling freq: fs"=w991, "X"=w1003) -> ("Filtered X"=w986:cdb[])  [unwired: 1 in, 1 out]
    n410 = Complex To Polar(r * e^(i*theta)=w986) -> (r=w989:dbl[], theta=w996:dbl[])
    n411 = Subtract(x=w996, y=w995) -> (x-y=w993:dbl[])
    n412 = call <vilib>:"Unwrap Phase.vi"("phase unit"=1 ("y"), "Phase"=w993) -> ("Unwrapped Phase"=w998:dbl[])  [unwired: 8 in, 1 out]
    n413 = local read "DownSamplingRatio"() -> (w1002:i32)
    n414 = local read "Waveform Size"() -> (w992:dbl)
    n415 = Divide(x=w992, y=w1002) -> (x/y=w999:dbl)
    n416 = Reshape Array(w989, w999, w1002) -> (w997:dbl[][])
    n417 = Reshape Array(w998, w999, w1002) -> (w1000:dbl[][])
    n418 = for {
      tunnel: w997 -> [w1013] mode=indexing
      tunnel: [w1012] -> w990 mode=indexing
      tunnel: w1000 -> [w1011] mode=indexing
      tunnel: [w1010] -> w1001 mode=indexing
      n419 = Add Array Elements(numeric array=w1013) -> (sum=w1012:dbl)
      n420 = Add Array Elements(numeric array=w1011) -> (sum=w1010:dbl)
    }
    n421 = Divide(x=w990, y=w1002) -> (x/y=w973:dbl[])
    n422 = Divide(x=w1001, y=w1002) -> (x/y=w972:dbl[])
    n423 = Build Array(w973, w972) -> (w967:dbl[][])
    "appended array" <- w967
    n424 = Array Size(array=w967) -> (size(s)=→"size(s)":i32[])
    n425 = case shown="False" "FlushSDR2" {
      tunnel: w974 -> [w1005 w1008]
      tunnel: w967 -> [_ w1009]
      tunnel: [w1004 w1006] -> w969
      frame True {
        n426 = Flush Queue(queue=w1005) -> (queue out=w1004:refnum<queue>)  [unwired: 1 in, 2 out]
      }
      frame False {
        n427 = Get Queue Status(queue=w1008) -> (# elements in queue=→"#queue 2":i32)  [unwired: 2 in, 7 out]
        n428 = Enqueue Element(queue=w1008, element=w1009) -> (queue out=w1006:refnum<queue>)  [unwired: 2 in, 2 out]
      }
    }
    "String 2" <- "Reading Rx2data"
  }
  n429 = while {
    shift-right: [w1021] -> _
    shift-left: T4."Default" -> [w1022]
    stop <- FALSE stop-if-true
    n430 = case shown="7" w1022 {
      tunnel: ["Routine" w1039 w1062 w1147 w1172 w1209 w1296 w1384 w1470 w1539 w1608 w1677] -> w1021
      tunnel: [0 1 2 3 4 5 6 7 8 9 10 11] -> w1020
      tunnel: [w1026 w1037 w1056 w1141 w1166 w1200 w1287 w1373 w1461 w1530 w1599 w1668] -> w1018
      tunnel: [w1029 w1044 w1052 "Relaxation phase.." "Perform the online attention test." w1198 w1286 w1374 w1460 w1529 w1598 w1667] -> w1019
      tunnel: [w1027 w1045 w1057 w1144 w1169 w1205 w1292 w1380 w1466 w1535 w1604 w1673] -> w1017
      tunnel: [w1026 w1037 w1053 w1141 w1166 w1199 w1285 w1375 w1459 w1528 w1597 w1666] -> w1016
      tunnel: ["" "" w1050 "" "" w1197 w1284 w1372 w1458 w1527 w1596 w1665] -> w1014
      frame 0, Default {
        w1029 = "Wait for instructions."  # Default
        w1026 = 0.0
        # "Waiting - intermediate state"
        n431 = Seconds To Date/Time(time stamp (now)=0.0) -> (date time rec=w1027:T2)  [unwired: 1 in]
        "Output" <- 0 ("Output")
        "Buffer" <- FALSE
        "Flush" <- FALSE ("Flush")
        "Save" <- FALSE ("Save")
      }
      frame 1 {
        w1037 = 0.0
        w1044 = "This is Test run. \nPress STOP TEST to exit and return to default."  # Default
        # "Test"
        n432 = Seconds To Date/Time(time stamp (now)=0.0) -> (date time rec=w1045:T2)  [unwired: 1 in]
        n433 = local write "Output"(1) -> ()
        n434 = local write "Buffer"(FALSE ("Buffer")) -> ()
        n435 = local write "Flush"(FALSE ("Flush")) -> ()
        n436 = local write "Save"(FALSE ("Save")) -> ()
        n437 = case shown="True" "Stop Test" {
          tunnel: [T10."Test" w1049] -> w1039
          frame False {
          }
          frame True {
            w1049 = T11."Default"
            n438 = local write "Routine"(w1049) -> ()
          }
        }
      }
      frame 2 {
        w1059 = 380.0  # Routine Time
        # "Routine 1"
        n439 = property on="Total Routine Time" class="Slide (strict)"("Scale.Maximum"=w1059) -> ()  [unwired: 2 in, 2 out]
        n440 = call "Elapsed Time5"("Time Target (s)"=w1059, "Auto Reset"=FALSE) -> ("Get Start Time (s)"=w1058:dbl, "Elapsed Time (s)"=w1056:dbl, "Time has Elapsed"=w1060:bool)  [unwired: 10 in, 5 out]
        "#1" <- w1060
        n441 = Seconds To Date/Time(time stamp (now)=w1058) -> (date time rec=w1057:T2)  [unwired: 1 in]
        n442 = Not(x=w1060) -> (.not. x?=w1063:bool)
        n443 = script code="t = [0,120,124,130,134,140,144,150,154,160,164,170,174,...\n       180,180.75,181.5,182.25,183,183.75,184.5,185.25,186,186.75,187.5,188.25,189,189.75,190.5,191.25,192,...\n       192.75,193.5,194.25,195,195.75,196.5,197.25,198,198.75,199.5,200.25,201,201.75,202.5,203.25,204,204.75,205.5,...\n       206.25,207,207.75,208.5,209.25,210,...\n        240,260,280,300,...\n        320,330,333,337,347,350,354,364,367,371,380];\n\nevent = [0,1,2,1,2,1,2,1,2,1,2,1,2,...\n               3,4,3,4,3,4,3,4,3,4,3,4,3,4,3,4,3,4,3,4,3,4,3,4,3,4,3,4,3,4,3,4,3,4,3,4,3,4,3,4,0,...\n               7,0,7,0,...\n               0,12,13,0,12,13,0,12,13,0,14];\n\nfor i = 2:length(t)\n    if ((x>=t(i-1)) &&  (x<t(i)))\n        y = event(i-1);\n        yNext = event(i);\n        dt = t(i) - t(i-1);\n        break;\n    end\nend"("x"=w1056) -> ("y"=w1051:dbl, "dt"=w1054:dbl, "yNext"=w1055:dbl)  [unwired: 1 in, 1 out]
        n444 = case shown="False" w1063 {
          tunnel: [w1122 w1134] -> w1062
          frame False {
            n445 = flat-sequence {
              tunnel: [w1130] -> w1122
              frame #0 {
                n446 = local write "Buffer"(FALSE ("Buffer")) -> ()
                n447 = local write "Play/Stop"(FALSE ("Play/Stop")) -> ()
              }
              frame #1 {
                n448 = local write "Output"(0 ("Output")) -> ()
                n449 = local write "Save"(TRUE ("Save")) -> ()
              }
              frame #2 {
                n450 = Wait (ms)(milliseconds to wait=u32 500) -> ()  [unwired: 1 out]
              }
              frame #3 {
                n451 = local write "Flush"(TRUE ("Flush")) -> ()
              }
              frame #4 {
                w1129 = u16 0 items=["No sound", "Demo deep breathing", "Demo fast shallow breathing", "Demo slow shallow breathing", "Demo breath hold", "Demo cough/ laugh", "Demo abdomen movement", "Calibration", "Routine 1", "Routine 3", "Routine 4/5/7", "Calm music"] ("Play sound")
                w1130 = u16 0 items=["Default"] ("Protocol")
                n452 = local write "Flush"(FALSE ("Flush")) -> ()
                n453 = local write "Save"(FALSE ("Save")) -> ()
                n454 = local write "Play sound"(w1129) -> ()
                n455 = local write "Routine"(w1130) -> ()
              }
            }
          }
          frame True {
            w1133 = u16 8 items=["No sound", "Demo normal breathing", "Demo deep breathing", "Demo fast shallow breathing", "Demo breath hold", "Demo cough", "Demo abdomen movement", "Calibration", "Routine 1", "(2a)Calm music", "(2b)Stress test", "Routine 3/4", "Routine 5", ""] ("Play sound")
            n456 = local write "Play sound"(w1133) -> ()
            n457 = flat-sequence {
              tunnel: [T4."Routine 1"] -> w1134
              frame #0 {
                n458 = local write "Output"(1 ("Open")) -> ()
                n459 = local write "Play/Stop"(TRUE ("Play/Stop")) -> ()
              }
              frame #1 {
                n460 = local write "Buffer"(TRUE ("Buffer")) -> ()
              }
              frame #2 {
              }
            }
          }
        }
        n461 = case shown="0, Default" w1051 {
          tunnel: ["\nPerform normal breathing. " "Inhale a slow deep breath." "\nExhale slowly." "Quick inhale.\n\n\n\nIf you cannot sustain for long, resume normal breathing." "\nQuick exhale.\n\n\nIf you cannot sustain for long, resume normal breathing." "Slow shallow inhale.\n\n\n\nIf you cannot sustain for long, resume normal breathing." "\nSlow exhale.\n\n\nIf you cannot sustain for long, resume normal breathing." "Exhale the current breath  and HOLD.\n\n\nIf you cannot sustain for long, resume normal breathing." "Perform voluntary coughing \n" "Perform voluntary laugh\n\n" "Read aloud the following text in between the lines:\n-----------------------------------------------------------------------\nFour score and seven years ago our fathers brought forth on this continent, a new nation, conceived in Liberty, and dedicated to the proposition that all men are created equal… That this nation, under God, shall have a new birth of freedom-and that government of the people, by the people, for the people, shall not perish from the earth.\n\n-----------------------------------------------------------------------\nWhen finished, take a deep breath and open mouth say \"Ah\" (like doctor checking your throat).\nPerform normal breathing until next instruction." "Exhale current breath and HOLD. Push abdomen inwards." "Relax abdomen back to normal and keep holding breath."] -> w1052
          frame 0, Default {
          }
          frame 1 {
          }
          frame 2 {
          }
          frame 3 {
          }
          frame 4 {
          }
          frame 5 {
          }
          frame 6 {
          }
          frame 7 {
          }
          frame 8 {
          }
          frame 9 {
          }
          frame 10 {
          }
          frame 12 {
          }
          frame 13 {
          }
        }
        n462 = case shown="0, Default" w1055 {
          tunnel: ["\nPerform normal breathing." "Inhale a slow deep breath." "\nExhale slowly." "Quick inhale.\n\n\n\nIf you cannot sustain for long, resume normal breathing." "\nQuick exhale.\n\n\nIf you cannot sustain for long, resume normal breathing." "Slow shallow inhale.\n\n\n\nIf you cannot sustain for long, resume normal breathing." "\nSlow exhale.\n\n\nIf you cannot sustain for long, resume normal breathing." "Exhale the current breath  and HOLD.\n\n\nIf you cannot sustain for long, resume normal breathing." "Perform voluntary coughing \n" "Perform voluntary laugh\n\n" "Read aloud the following text in between the lines:\n-----------------------------------------------------------------------\nFour score and seven years ago our fathers brought forth on this continent, a new nation, conceived in Liberty, and dedicated to the proposition that all men are created equal… That this nation, under God, shall have a new birth of freedom-and that government of the people, by the people, for the people, shall not perish from the earth.\n\n-----------------------------------------------------------------------\nWhen finished, take a deep breath and open mouth say \"Ah\" (like doctor checking your throat).\nPerform normal breathing until next instruction." "Exhale current breath and HOLD. Push abdomen inwards." "Relax abdomen back to normal and keep holding breath." "Wait for next routine!"] -> w1050
          frame 0, Default {
          }
          frame 1 {
          }
          frame 2 {
          }
          frame 3 {
          }
          frame 4 {
          }
          frame 5 {
          }
          frame 6 {
          }
          frame 7 {
          }
          frame 8 {
          }
          frame 9 {
          }
          frame 10 {
          }
          frame 12 {
          }
          frame 13 {
          }
          frame 14 {
          }
        }
        n463 = case shown="2" w1051 {
          tunnel: w1054 -> [w1067 w1069 w1071 w1073 w1075 w1077 w1079 w1081 w1083 w1085 w1087 w1089 w1091 w1094]
          tunnel: [w1066 w1068 w1070 w1072 w1074 w1076 w1078 w1080 w1082 w1084 w1086 w1088 w1090 w1093] -> w1053
          frame 1 {
            n464 = property on="Current Task time" class="Slide (strict)"("Scale.Maximum"=w1067) -> ()  [unwired: 2 in, 2 out]
            n465 = call "Elapsed Time11"("Time Target (s)"=w1067) -> ("Elapsed Time (s)"=w1066:dbl)  [unwired: 11 in, 7 out]
            n466 = property on="Current Task time" class="Slide (strict)"("Scale.Minimum"=0.0 ("Scale.Range:Minimum")) -> ()  [unwired: 2 in, 2 out]
          }
          frame 2 {
            n467 = property on="Current Task time" class="Slide (strict)"("Scale.Maximum"=w1069) -> ()  [unwired: 2 in, 2 out]
            n468 = call "Elapsed Time12"("Time Target (s)"=w1069) -> ("Elapsed Time (s)"=w1068:dbl)  [unwired: 11 in, 7 out]
          }
          frame 3 {
            n469 = property on="Current Task time" class="Slide (strict)"("Scale.Maximum"=w1071) -> ()  [unwired: 2 in, 2 out]
            n470 = call "Elapsed Time13"("Time Target (s)"=w1071) -> ("Elapsed Time (s)"=w1070:dbl)  [unwired: 11 in, 7 out]
          }
          frame 4 {
            n471 = property on="Current Task time" class="Slide (strict)"("Scale.Maximum"=w1073) -> ()  [unwired: 2 in, 2 out]
            n472 = call "Elapsed Time14"("Time Target (s)"=w1073) -> ("Elapsed Time (s)"=w1072:dbl)  [unwired: 11 in, 7 out]
          }
          frame 5 {
            n473 = property on="Current Task time" class="Slide (strict)"("Scale.Maximum"=w1075) -> ()  [unwired: 2 in, 2 out]
            n474 = call "Elapsed Time15"("Time Target (s)"=w1075) -> ("Elapsed Time (s)"=w1074:dbl)  [unwired: 11 in, 7 out]
          }
          frame 6 {
            n475 = property on="Current Task time" class="Slide (strict)"("Scale.Maximum"=w1077) -> ()  [unwired: 2 in, 2 out]
            n476 = call "Elapsed Time16"("Time Target (s)"=w1077) -> ("Elapsed Time (s)"=w1076:dbl)  [unwired: 11 in, 7 out]
          }
          frame 7 {
            n477 = property on="Current Task time" class="Slide (strict)"("Scale.Maximum"=w1079) -> ()  [unwired: 2 in, 2 out]
            n478 = call "Elapsed Time17"("Time Target (s)"=w1079) -> ("Elapsed Time (s)"=w1078:dbl)  [unwired: 11 in, 7 out]
          }
          frame 8 {
            n479 = property on="Current Task time" class="Slide (strict)"("Scale.Maximum"=w1081) -> ()  [unwired: 2 in, 2 out]
            n480 = call "Elapsed Time18"("Time Target (s)"=w1081) -> ("Elapsed Time (s)"=w1080:dbl)  [unwired: 11 in, 7 out]
          }
          frame 9 {
            n481 = property on="Current Task time" class="Slide (strict)"("Scale.Maximum"=w1083) -> ()  [unwired: 2 in, 2 out]
            n482 = call "Elapsed Time19"("Time Target (s)"=w1083) -> ("Elapsed Time (s)"=w1082:dbl)  [unwired: 11 in, 7 out]
          }
          frame 10 {
            n483 = property on="Current Task time" class="Slide (strict)"("Scale.Maximum"=w1085) -> ()  [unwired: 2 in, 2 out]
            n484 = call "Elapsed Time20"("Time Target (s)"=w1085) -> ("Elapsed Time (s)"=w1084:dbl)  [unwired: 11 in, 7 out]
          }
          frame 11 {
            n485 = property on="Current Task time" class="Slide (strict)"("Scale.Maximum"=w1087) -> ()  [unwired: 2 in, 2 out]
            n486 = call "Elapsed Time21"("Time Target (s)"=w1087) -> ("Elapsed Time (s)"=w1086:dbl)  [unwired: 11 in, 7 out]
          }
          frame 12 {
            n487 = property on="Current Task time" class="Slide (strict)"("Scale.Maximum"=w1089) -> ()  [unwired: 2 in, 2 out]
            n488 = call "Elapsed Time22"("Time Target (s)"=w1089) -> ("Elapsed Time (s)"=w1088:dbl)  [unwired: 11 in, 7 out]
          }
          frame 13 {
            n489 = property on="Current Task time" class="Slide (strict)"("Scale.Maximum"=w1091) -> ()  [unwired: 2 in, 2 out]
            n490 = call "Elapsed Time23"("Time Target (s)"=w1091) -> ("Elapsed Time (s)"=w1090:dbl)  [unwired: 11 in, 7 out]
          }
          frame 0, Default {
            n491 = property on="Current Task time" class="Slide (strict)"("Scale.Maximum"=w1094) -> ()  [unwired: 2 in, 2 out]
            n492 = call "Elapsed Time24"("Time Target (s)"=w1094) -> ("Elapsed Time (s)"=w1093:dbl)  [unwired: 11 in, 7 out]
            n493 = property on="Current Task time" class="Slide (strict)"("Scale.Minimum"=0.0 ("Scale.Range:Minimum")) -> ()  [unwired: 2 in, 2 out]
          }
        }
      }
      frame 3 {
        w1140 = 120.0  # Routine Time
        # "Routine 2a: Attention test - calm"
        n494 = property on="Total Routine Time" class="Slide (strict)"("Scale.Maximum"=w1140) -> ()  [unwired: 2 in, 2 out]
        n495 = property on="Current Task time" class="Slide (strict)"("Scale.Maximum"=w1140) -> ()  [unwired: 2 in, 2 out]
        n496 = call "Elapsed Time7"("Time Target (s)"=w1140, "Auto Reset"=FALSE ("Timer Reset")) -> ("Get Start Time (s)"=w1143:dbl, "Elapsed Time (s)"=w1141:dbl, "Time has Elapsed"=w1145:bool)  [unwired: 10 in, 5 out]
        "#2a" <- w1145
        n497 = Seconds To Date/Time(time stamp (now)=w1143) -> (date time rec=w1144:T2)  [unwired: 1 in]
        n498 = Not(x=w1145) -> (.not. x?=w1148:bool)
        n499 = case shown="False" w1148 {
          tunnel: [w1150 w1159] -> w1147
          frame False {
            n500 = flat-sequence {
              tunnel: [w1156] -> w1150
              frame #0 {
                n501 = local write "Buffer"(FALSE ("Buffer")) -> ()
              }
              frame #1 {
                n502 = local write "Output"(0 ("Output")) -> ()
                n503 = local write "Save"(TRUE ("Save")) -> ()
              }
              frame #2 {
                n504 = Wait (ms)(milliseconds to wait=u32 500) -> ()  [unwired: 1 out]
              }
              frame #3 {
                n505 = local write "Flush"(TRUE ("Flush")) -> ()
              }
              frame #4 {
                w1156 = enum16{"Default"}."Default"
                n506 = local write "Flush"(FALSE ("Flush")) -> ()
                n507 = local write "Save"(FALSE ("Save")) -> ()
                n508 = local write "Routine"(w1156) -> ()
              }
            }
          }
          frame True {
            n509 = flat-sequence {
              tunnel: [T4."Routine 2a"] -> w1159
              frame #0 {
                n510 = local write "Output"(1 ("Open")) -> ()
                n511 = local write "Play/Stop"(TRUE ("PlayMusic")) -> ()
              }
              frame #1 {
                n512 = local write "Buffer"(TRUE ("Buffer")) -> ()
              }
              frame #2 {
              }
            }
          }
        }
      }
      frame 4 {
        w1165 = 400.0  # Routine Time
        # "Routine 2b: Attention/Stress test"
        n513 = property on="Total Routine Time" class="Slide (strict)"("Scale.Maximum"=w1165) -> ()  [unwired: 2 in, 2 out]
        n514 = property on="Current Task time" class="Slide (strict)"("Scale.Maximum"=w1165) -> ()  [unwired: 2 in, 2 out]
        n515 = call "Elapsed Time9"("Time Target (s)"=w1165, "Auto Reset"=FALSE ("Timer Reset")) -> ("Get Start Time (s)"=w1168:dbl, "Elapsed Time (s)"=w1166:dbl, "Time has Elapsed"=w1170:bool)  [unwired: 10 in, 5 out]
        "#2b" <- w1170
        n516 = Seconds To Date/Time(time stamp (now)=w1168) -> (date time rec=w1169:T2)  [unwired: 1 in]
        n517 = Not(x=w1170) -> (.not. x?=w1173:bool)
        n518 = case shown="True" w1173 {
          tunnel: [w1175 w1187] -> w1172
          frame False {
            n519 = flat-sequence {
              tunnel: [w1182] -> w1175
              frame #0 {
                n520 = local write "Buffer"(FALSE ("Buffer")) -> ()
                n521 = local write "Play/Stop"(FALSE ("Play/Stop")) -> ()
              }
              frame #1 {
                n522 = local write "Output"(0 ("Output")) -> ()
                n523 = local write "Save"(TRUE ("Save")) -> ()
              }
              frame #2 {
                n524 = Wait (ms)(milliseconds to wait=u32 500) -> ()  [unwired: 1 out]
              }
              frame #3 {
                n525 = local write "Flush"(TRUE ("Flush")) -> ()
              }
              frame #4 {
                w1182 = enum16{"Default"}."Default"
                n526 = local write "Flush"(FALSE ("Flush")) -> ()
                n527 = local write "Save"(FALSE ("Save")) -> ()
                n528 = local write "Routine"(w1182) -> ()
              }
            }
          }
          frame True {
            w1185 = u16 10 items=["No sound", "Demo normal breathing", "Demo deep breathing", "Demo fast shallow breathing", "Demo breath hold", "Demo cough", "Demo abdomen movement", "Calibration", "Routine 1", "(2a)Calm music", "(2b)Stress test", "Routine 3/4", "Routine 5", ""] ("Play sound")
            n529 = local write "Play sound"(w1185) -> ()
            n530 = flat-sequence {
              tunnel: "OpenHTML" -> [w1189]
              tunnel: [T4."Routine 2b"] -> w1187
              frame #0 {
                n531 = And(x=TRUE, y=w1189) -> (x .and. y?=w1191:bool)
                n532 = case shown="True" w1191 {
                  frame False {
                  }
                  frame True {
                    n533 = local write "OpenHTML"(FALSE ("OpenHTML")) -> ()
                    n534 = call-poly <vilib>:"Open URL in Default Browser.vi"("URL"="\"E:\\NCS\\HumanStudyMarch2019\\StressTest\\mackworth\\vigilanceTest.html\"") -> ()  [unwired: 5 in, 2 out]
                  }
                }
                n535 = local write "Play/Stop"(TRUE ("Play/Stop")) -> ()
                n536 = local write "Output"(1 ("Open")) -> ()
              }
              frame #1 {
                n537 = local write "Buffer"(TRUE ("Buffer")) -> ()
              }
              frame #2 {
              }
            }
          }
        }
      }
      frame 5 {
        w1206 = 320.0  # Routine Time
        # "Routine 3: Lying on bed in supine"
        n538 = property on="Total Routine Time" class="Slide (strict)"("Scale.Maximum"=w1206) -> ()  [unwired: 2 in, 2 out]
        n539 = call "Elapsed Time"("Time Target (s)"=w1206, "Auto Reset"=FALSE ("Timer Reset")) -> ("Get Start Time (s)"=w1204:dbl, "Elapsed Time (s)"=w1200:dbl, "Time has Elapsed"=w1207:bool)  [unwired: 10 in, 5 out]
        "#3" <- w1207
        n540 = Seconds To Date/Time(time stamp (now)=w1204) -> (date time rec=w1205:T2)  [unwired: 1 in]
        n541 = Not(x=w1207) -> (.not. x?=w1210:bool)
        n542 = script code="t = [0,120,124,130,134,140,144,150,154,160,164,170,174,...\n       180,180.75,181.5,182.25,183,183.75,184.5,185.25,186,186.75,187.5,188.25,189,189.75,190.5,191.25,192,...\n       192.75,193.5,194.25,195,195.75,196.5,197.25,198,198.75,199.5,200.25,201,201.75,202.5,203.25,204,204.75,205.5,...\n       206.25,207,207.75,208.5,209.25,210,...\n        240,260,280,300,...\n        320];\n\nevent = [0,1,2,1,2,1,2,1,2,1,2,1,2,...\n               3,4,3,4,3,4,3,4,3,4,3,4,3,4,3,4,3,4,3,4,3,4,3,4,3,4,3,4,3,4,3,4,3,4,3,4,3,4,3,4,0,...\n               7,0,7,0,...\n               14];\n\nfor i = 2:length(t)\n    if ((x>=t(i-1)) &&  (x<t(i)))\n        y = event(i-1);\n        yNext = event(i);\n        dt = t(i) - t(i-1);\n        break;\n    end\nend"("x"=w1200) -> ("y"=w1201:dbl, "dt"=w1202:dbl, "yNext"=w1203:dbl)  [unwired: 1 in, 1 out]
        n543 = case shown="True" w1210 {
          tunnel: [w1267 w1279] -> w1209
          frame False {
            n544 = flat-sequence {
              tunnel: [w1275] -> w1267
              frame #0 {
                n545 = local write "Buffer"(FALSE ("Buffer")) -> ()
                n546 = local write "Play/Stop"(FALSE ("PlayInstr")) -> ()
              }
              frame #1 {
                n547 = local write "Output"(0 ("Output")) -> ()
                n548 = local write "Save"(TRUE ("Save")) -> ()
              }
              frame #2 {
                n549 = Wait (ms)(milliseconds to wait=u32 500) -> ()  [unwired: 1 out]
              }
              frame #3 {
                n550 = local write "Flush"(TRUE ("Flush")) -> ()
              }
              frame #4 {
                w1274 = u16 0 items=["No sound", "Demo deep breathing", "Demo fast shallow breathing", "Demo slow shallow breathing", "Demo breath hold", "Demo cough/ laugh", "Demo abdomen movement", "Calibration", "Routine 1", "Routine 3", "Routine 4/5/7", "Calm music"] ("Play sound")
                w1275 = enum16{"Default"}."Default"
                n551 = local write "Flush"(FALSE ("Flush")) -> ()
                n552 = local write "Save"(FALSE ("Save")) -> ()
                n553 = local write "Play sound"(w1274) -> ()
                n554 = local write "Routine"(w1275) -> ()
              }
            }
          }
          frame True {
            w1278 = u16 11 items=["No sound", "Demo normal breathing", "Demo deep breathing", "Demo fast shallow breathing", "Demo breath hold", "Demo cough", "Demo abdomen movement", "Calibration", "Routine 1", "(2a)Calm music", "(2b)Stress test", "Routine 3/4", "Routine 5", ""] ("Play sound")
            n555 = local write "Play sound"(w1278) -> ()
            n556 = flat-sequence {
              tunnel: [T4."Routine 3"] -> w1279
              frame #0 {
                n557 = local write "Output"(1 ("Open")) -> ()
                n558 = local write "Play/Stop"(TRUE ("PlayInstruction")) -> ()
              }
              frame #1 {
                n559 = local write "Buffer"(TRUE ("Buffer")) -> ()
              }
              frame #2 {
              }
            }
          }
        }
        n560 = case shown="0, Default" w1201 {
          tunnel: ["\nPerform normal breathing." "Inhale a slow deep breath." "\nExhale slowly." "Quick inhale.\n\n\n\nIf you cannot sustain for long, resume normal breathing." "\nQuick exhale.\n\n\nIf you cannot sustain for long, resume normal breathing." "Slow shallow inhale.\n\n\n\nIf you cannot sustain for long, resume normal breathing." "\nSlow exhale.\n\n\nIf you cannot sustain for long, resume normal breathing." "Exhale the current breath  and HOLD.\n\n\nIf you cannot sustain for long, resume normal breathing." "Perform voluntary coughing \n" "Perform voluntary laugh\n\n" "Read aloud the following text in between the lines:\n-----------------------------------------------------------------------\nFour score and seven years ago our fathers brought forth on this continent, a new nation, conceived in Liberty, and dedicated to the proposition that all men are created equal… That this nation, under God, shall have a new birth of freedom-and that government of the people, by the people, for the people, shall not perish from the earth.\n\n-----------------------------------------------------------------------\nWhen finished, take a deep breath and open mouth say \"Ah\" (like doctor checking your throat).\nPerform normal breathing until next instruction." "Exhale current breath and HOLD. Push abdomen inwards." "Relax abdomen back to normal and keep holding breath."] -> w1198
          frame 0, Default {
          }
          frame 1 {
          }
          frame 2 {
          }
          frame 3 {
          }
          frame 4 {
          }
          frame 5 {
          }
          frame 6 {
          }
          frame 7 {
          }
          frame 8 {
          }
          frame 9 {
          }
          frame 10 {
          }
          frame 12 {
          }
          frame 13 {
          }
        }
        n561 = case shown="14" w1203 {
          tunnel: ["\nPerform normal breathing." "Inhale a slow deep breath." "\nExhale slowly." "Quick inhale.\n\n\n\nIf you cannot sustain for long, resume normal breathing." "\nQuick exhale.\n\n\nIf you cannot sustain for long, resume normal breathing." "Slow shallow inhale.\n\n\n\nIf you cannot sustain for long, resume normal breathing." "\nSlow exhale.\n\n\nIf you cannot sustain for long, resume normal breathing." "Exhale the current breath  and HOLD.\n\n\nIf you cannot sustain for long, resume normal breathing." "Perform voluntary coughing \n" "Perform voluntary laugh\n\n" "Read aloud the following text in between the lines:\n-----------------------------------------------------------------------\nFour score and seven years ago our fathers brought forth on this continent, a new nation, conceived in Liberty, and dedicated to the proposition that all men are created equal… That this nation, under God, shall have a new birth of freedom-and that government of the people, by the people, for the people, shall not perish from the earth.\n\n-----------------------------------------------------------------------\nWhen finished, take a deep breath and open mouth say \"Ah\" (like doctor checking your throat).\nPerform normal breathing until next instruction." "Exhale current breath and HOLD. Push abdomen inwards." "Relax abdomen back to normal and keep holding breath." "Wait for next routine!"] -> w1197
          frame 0, Default {
          }
          frame 1 {
          }
          frame 2 {
          }
          frame 3 {
          }
          frame 4 {
          }
          frame 5 {
          }
          frame 6 {
          }
          frame 7 {
          }
          frame 8 {
          }
          frame 9 {
          }
          frame 10 {
          }
          frame 12 {
          }
          frame 13 {
          }
          frame 14 {
          }
        }
        n562 = case shown="5" w1201 {
          tunnel: w1202 -> [w1213 w1215 w1217 w1219 w1221 w1223 w1225 w1227 w1229 w1231 w1233 w1235 w1237 w1239]
          tunnel: [w1212 w1214 w1216 w1218 w1220 w1222 w1224 w1226 w1228 w1230 w1232 w1234 w1236 w1238] -> w1199
          frame 1 {
            n563 = property on="Current Task time" class="Slide (strict)"("Scale.Maximum"=w1213) -> ()  [unwired: 2 in, 2 out]
            n564 = call "Elapsed Time34"("Time Target (s)"=w1213) -> ("Elapsed Time (s)"=w1212:dbl)  [unwired: 11 in, 7 out]
          }
          frame 2 {
            n565 = property on="Current Task time" class="Slide (strict)"("Scale.Maximum"=w1215) -> ()  [unwired: 2 in, 2 out]
            n566 = call "Elapsed Time35"("Time Target (s)"=w1215) -> ("Elapsed Time (s)"=w1214:dbl)  [unwired: 11 in, 7 out]
          }
          frame 3 {
            n567 = property on="Current Task time" class="Slide (strict)"("Scale.Maximum"=w1217) -> ()  [unwired: 2 in, 2 out]
            n568 = call "Elapsed Time36"("Time Target (s)"=w1217) -> ("Elapsed Time (s)"=w1216:dbl)  [unwired: 11 in, 7 out]
          }
          frame 4 {
            n569 = property on="Current Task time" class="Slide (strict)"("Scale.Maximum"=w1219) -> ()  [unwired: 2 in, 2 out]
            n570 = call "Elapsed Time37"("Time Target (s)"=w1219) -> ("Elapsed Time (s)"=w1218:dbl)  [unwired: 11 in, 7 out]
          }
          frame 5 {
            n571 = property on="Current Task time" class="Slide (strict)"("Scale.Maximum"=w1221) -> ()  [unwired: 2 in, 2 out]
            n572 = call "Elapsed Time38"("Time Target (s)"=w1221) -> ("Elapsed Time (s)"=w1220:dbl)  [unwired: 11 in, 7 out]
          }
          frame 6 {
            n573 = property on="Current Task time" class="Slide (strict)"("Scale.Maximum"=w1223) -> ()  [unwired: 2 in, 2 out]
            n574 = call "Elapsed Time39"("Time Target (s)"=w1223) -> ("Elapsed Time (s)"=w1222:dbl)  [unwired: 11 in, 7 out]
          }
          frame 7 {
            n575 = property on="Current Task time" class="Slide (strict)"("Scale.Maximum"=w1225) -> ()  [unwired: 2 in, 2 out]
            n576 = call "Elapsed Time40"("Time Target (s)"=w1225) -> ("Elapsed Time (s)"=w1224:dbl)  [unwired: 11 in, 7 out]
          }
          frame 8 {
            n577 = property on="Current Task time" class="Slide (strict)"("Scale.Maximum"=w1227) -> ()  [unwired: 2 in, 2 out]
            n578 = call "Elapsed Time41"("Time Target (s)"=w1227) -> ("Elapsed Time (s)"=w1226:dbl)  [unwired: 11 in, 7 out]
          }
          frame 9 {
            n579 = property on="Current Task time" class="Slide (strict)"("Scale.Maximum"=w1229) -> ()  [unwired: 2 in, 2 out]
            n580 = call "Elapsed Time42"("Time Target (s)"=w1229) -> ("Elapsed Time (s)"=w1228:dbl)  [unwired: 11 in, 7 out]
          }
          frame 10 {
            n581 = property on="Current Task time" class="Slide (strict)"("Scale.Maximum"=w1231) -> ()  [unwired: 2 in, 2 out]
            n582 = call "Elapsed Time43"("Time Target (s)"=w1231) -> ("Elapsed Time (s)"=w1230:dbl)  [unwired: 11 in, 7 out]
          }
          frame 11 {
            n583 = property on="Current Task time" class="Slide (strict)"("Scale.Maximum"=w1233) -> ()  [unwired: 2 in, 2 out]
            n584 = call "Elapsed Time44"("Time Target (s)"=w1233) -> ("Elapsed Time (s)"=w1232:dbl)  [unwired: 11 in, 7 out]
          }
          frame 12 {
            n585 = property on="Current Task time" class="Slide (strict)"("Scale.Maximum"=w1235) -> ()  [unwired: 2 in, 2 out]
            n586 = call "Elapsed Time45"("Time Target (s)"=w1235) -> ("Elapsed Time (s)"=w1234:dbl)  [unwired: 11 in, 7 out]
          }
          frame 13 {
            n587 = property on="Current Task time" class="Slide (strict)"("Scale.Maximum"=w1237) -> ()  [unwired: 2 in, 2 out]
            n588 = call "Elapsed Time122"("Time Target (s)"=w1237) -> ("Elapsed Time (s)"=w1236:dbl)  [unwired: 11 in, 7 out]
          }
          frame 0, Default {
            n589 = property on="Current Task time" class="Slide (strict)"("Scale.Maximum"=w1239) -> ()  [unwired: 2 in, 2 out]
            n590 = call "Elapsed Time123"("Time Target (s)"=w1239) -> ("Elapsed Time (s)"=w1238:dbl)  [unwired: 11 in, 7 out]
          }
        }
      }
      frame 6 {
        w1293 = 320.0  # Routine Time
        # "Routine 4: Lying on bed turned"
        n591 = property on="Total Routine Time" class="Slide (strict)"("Scale.Maximum"=w1293) -> ()  [unwired: 2 in, 2 out]
        n592 = call "Elapsed Time2"("Time Target (s)"=w1293, "Auto Reset"=FALSE ("Timer Reset")) -> ("Get Start Time (s)"=w1291:dbl, "Elapsed Time (s)"=w1287:dbl, "Time has Elapsed"=w1294:bool)  [unwired: 10 in, 5 out]
        "#4" <- w1294
        n593 = Seconds To Date/Time(time stamp (now)=w1291) -> (date time rec=w1292:T2)  [unwired: 1 in]
        n594 = Not(x=w1294) -> (.not. x?=w1297:bool)
        n595 = script code="t = [0,120,124,130,134,140,144,150,154,160,164,170,174,...\n       180,180.75,181.5,182.25,183,183.75,184.5,185.25,186,186.75,187.5,188.25,189,189.75,190.5,191.25,192,...\n       192.75,193.5,194.25,195,195.75,196.5,197.25,198,198.75,199.5,200.25,201,201.75,202.5,203.25,204,204.75,205.5,...\n       206.25,207,207.75,208.5,209.25,210,...\n        240,260,280,300,...\n        320];\n\nevent = [0,1,2,1,2,1,2,1,2,1,2,1,2,...\n               3,4,3,4,3,4,3,4,3,4,3,4,3,4,3,4,3,4,3,4,3,4,3,4,3,4,3,4,3,4,3,4,3,4,3,4,3,4,3,4,0,...\n               7,0,7,0,...\n               14];\n\nfor i = 2:length(t)\n    if ((x>=t(i-1)) &&  (x<t(i)))\n        y = event(i-1);\n        yNext = event(i);\n        dt = t(i) - t(i-1);\n        break;\n    end\nend"("x"=w1287) -> ("y"=w1288:dbl, "dt"=w1289:dbl, "yNext"=w1290:dbl)  [unwired: 1 in, 1 out]
        n596 = case shown="True" w1297 {
          tunnel: [w1354 w1366] -> w1296
          frame False {
            n597 = flat-sequence {
              tunnel: [w1362] -> w1354
              frame #0 {
                n598 = local write "Buffer"(FALSE ("Buffer")) -> ()
                n599 = local write "Play/Stop"(FALSE ("PlayInstruction")) -> ()
              }
              frame #1 {
                n600 = local write "Output"(0 ("Output")) -> ()
                n601 = local write "Save"(TRUE ("Save")) -> ()
              }
              frame #2 {
                n602 = Wait (ms)(milliseconds to wait=u32 500) -> ()  [unwired: 1 out]
              }
              frame #3 {
                n603 = local write "Flush"(TRUE ("Flush")) -> ()
              }
              frame #4 {
                w1361 = u16 0 items=["No sound", "Demo deep breathing", "Demo fast shallow breathing", "Demo slow shallow breathing", "Demo breath hold", "Demo cough/ laugh", "Demo abdomen movement", "Calibration", "Routine 1", "Routine 3", "Routine 4/5/7", "Calm music"] ("Play sound")
                w1362 = enum16{"Default"}."Default"
                n604 = local write "Flush"(FALSE ("Flush")) -> ()
                n605 = local write "Save"(FALSE ("Save")) -> ()
                n606 = local write "Play sound"(w1361) -> ()
                n607 = local write "Routine"(w1362) -> ()
              }
            }
          }
          frame True {
            w1365 = u16 11 items=["No sound", "Demo normal breathing", "Demo deep breathing", "Demo fast shallow breathing", "Demo breath hold", "Demo cough", "Demo abdomen movement", "Calibration", "Routine 1", "(2a)Calm music", "(2b)Stress test", "Routine 3/4", "Routine 5", ""] ("Play sound")
            n608 = local write "Play sound"(w1365) -> ()
            n609 = flat-sequence {
              tunnel: [T4."Routine 4"] -> w1366
              frame #0 {
                n610 = local write "Output"(1 ("Open")) -> ()
                n611 = local write "Play/Stop"(TRUE ("PlayInstruction")) -> ()
              }
              frame #1 {
                n612 = local write "Buffer"(TRUE ("Buffer")) -> ()
              }
              frame #2 {
              }
            }
          }
        }
        n613 = case shown="0, Default" w1288 {
          tunnel: ["\nPerform normal breathing." "Inhale a slow deep breath." "\nExhale slowly." "Quick inhale.\n\n\n\nIf you cannot sustain for long, resume normal breathing." "\nQuick exhale.\n\n\nIf you cannot sustain for long, resume normal breathing." "Slow shallow inhale.\n\n\n\nIf you cannot sustain for long, resume normal breathing." "\nSlow exhale.\n\n\nIf you cannot sustain for long, resume normal breathing." "Exhale the current breath  and HOLD.\n\n\nIf you cannot sustain for long, resume normal breathing." "Perform voluntary coughing \n" "Perform voluntary laugh\n\n" "Read aloud the following text in between the lines:\n-----------------------------------------------------------------------\nFour score and seven years ago our fathers brought forth on this continent, a new nation, conceived in Liberty, and dedicated to the proposition that all men are created equal… That this nation, under God, shall have a new birth of freedom-and that government of the people, by the people, for the people, shall not perish from the earth.\n\n-----------------------------------------------------------------------\nWhen finished, take a deep breath and open mouth say \"Ah\" (like doctor checking your throat).\nPerform normal breathing until next instruction." "Exhale current breath and HOLD. Push abdomen inwards." "Relax abdomen back to normal and keep holding breath."] -> w1286
          frame 0, Default {
          }
          frame 1 {
          }
          frame 2 {
          }
          frame 3 {
          }
          frame 4 {
          }
          frame 5 {
          }
          frame 6 {
          }
          frame 7 {
          }
          frame 8 {
          }
          frame 9 {
          }
          frame 10 {
          }
          frame 12 {
          }
          frame 13 {
          }
        }
        n614 = case shown="14" w1290 {
          tunnel: ["\nPerform normal breathing." "Inhale a slow deep breath." "\nExhale slowly." "Quick inhale.\n\n\n\nIf you cannot sustain for long, resume normal breathing." "\nQuick exhale.\n\n\nIf you cannot sustain for long, resume normal breathing." "Slow shallow inhale.\n\n\n\nIf you cannot sustain for long, resume normal breathing." "\nSlow exhale.\n\n\nIf you cannot sustain for long, resume normal breathing." "Exhale the current breath  and HOLD.\n\n\nIf you cannot sustain for long, resume normal breathing." "Perform voluntary coughing \n" "Perform voluntary laugh\n\n" "Read aloud the following text in between the lines:\n-----------------------------------------------------------------------\nFour score and ...\n-----------------------------------------------------------------------\nWhen finished, take a deep breath and open mouth say \"Ah\" (like doctor checking your throat).\nPerform normal breathing until next instruction." "Exhale current breath and HOLD. Push abdomen inwards." "Relax abdomen back to normal and keep holding breath." "Wait for next routine!"] -> w1284
          frame 0, Default {
          }
          frame 1 {
          }
          frame 2 {
          }
          frame 3 {
          }
          frame 4 {
          }
          frame 5 {
          }
          frame 6 {
          }
          frame 7 {
          }
          frame 8 {
          }
          frame 9 {
          }
          frame 10 {
          }
          frame 12 {
          }
          frame 13 {
          }
          frame 14 {
          }
        }
        n615 = case shown="0, Default" w1288 {
          tunnel: w1289 -> [w1300 w1302 w1304 w1306 w1308 w1310 w1312 w1314 w1316 w1318 w1320 w1322 w1324 w1326]
          tunnel: [w1299 w1301 w1303 w1305 w1307 w1309 w1311 w1313 w1315 w1317 w1319 w1321 w1323 w1325] -> w1285
          frame 1 {
            n616 = property on="Current Task time" class="Slide (strict)"("Scale.Maximum"=w1300) -> ()  [unwired: 2 in, 2 out]
            n617 = call "Elapsed Time46"("Time Target (s)"=w1300) -> ("Elapsed Time (s)"=w1299:dbl)  [unwired: 11 in, 7 out]
          }
          frame 2 {
            n618 = property on="Current Task time" class="Slide (strict)"("Scale.Maximum"=w1302) -> ()  [unwired: 2 in, 2 out]
            n619 = call "Elapsed Time47"("Time Target (s)"=w1302) -> ("Elapsed Time (s)"=w1301:dbl)  [unwired: 11 in, 7 out]
          }
          frame 3 {
            n620 = property on="Current Task time" class="Slide (strict)"("Scale.Maximum"=w1304) -> ()  [unwired: 2 in, 2 out]
            n621 = call "Elapsed Time48"("Time Target (s)"=w1304) -> ("Elapsed Time (s)"=w1303:dbl)  [unwired: 11 in, 7 out]
          }
          frame 4 {
            n622 = property on="Current Task time" class="Slide (strict)"("Scale.Maximum"=w1306) -> ()  [unwired: 2 in, 2 out]
            n623 = call "Elapsed Time49"("Time Target (s)"=w1306) -> ("Elapsed Time (s)"=w1305:dbl)  [unwired: 11 in, 7 out]
          }
          frame 5 {
            n624 = property on="Current Task time" class="Slide (strict)"("Scale.Maximum"=w1308) -> ()  [unwired: 2 in, 2 out]
            n625 = call "Elapsed Time50"("Time Target (s)"=w1308) -> ("Elapsed Time (s)"=w1307:dbl)  [unwired: 11 in, 7 out]
          }
          frame 6 {
            n626 = property on="Current Task time" class="Slide (strict)"("Scale.Maximum"=w1310) -> ()  [unwired: 2 in, 2 out]
            n627 = call "Elapsed Time51"("Time Target (s)"=w1310) -> ("Elapsed Time (s)"=w1309:dbl)  [unwired: 11 in, 7 out]
          }
          frame 7 {
            n628 = property on="Current Task time" class="Slide (strict)"("Scale.Maximum"=w1312) -> ()  [unwired: 2 in, 2 out]
            n629 = call "Elapsed Time52"("Time Target (s)"=w1312) -> ("Elapsed Time (s)"=w1311:dbl)  [unwired: 11 in, 7 out]
          }
          frame 8 {
            n630 = property on="Current Task time" class="Slide (strict)"("Scale.Maximum"=w1314) -> ()  [unwired: 2 in, 2 out]
            n631 = call "Elapsed Time53"("Time Target (s)"=w1314) -> ("Elapsed Time (s)"=w1313:dbl)  [unwired: 11 in, 7 out]
          }
          frame 9 {
            n632 = property on="Current Task time" class="Slide (strict)"("Scale.Maximum"=w1316) -> ()  [unwired: 2 in, 2 out]
            n633 = call "Elapsed Time54"("Time Target (s)"=w1316) -> ("Elapsed Time (s)"=w1315:dbl)  [unwired: 11 in, 7 out]
          }
          frame 10 {
            n634 = property on="Current Task time" class="Slide (strict)"("Scale.Maximum"=w1318) -> ()  [unwired: 2 in, 2 out]
            n635 = call "Elapsed Time55"("Time Target (s)"=w1318) -> ("Elapsed Time (s)"=w1317:dbl)  [unwired: 11 in, 7 out]
          }
          frame 11 {
            n636 = property on="Current Task time" class="Slide (strict)"("Scale.Maximum"=w1320) -> ()  [unwired: 2 in, 2 out]
            n637 = call "Elapsed Time56"("Time Target (s)"=w1320) -> ("Elapsed Time (s)"=w1319:dbl)  [unwired: 11 in, 7 out]
          }
          frame 12 {
            n638 = property on="Current Task time" class="Slide (strict)"("Scale.Maximum"=w1322) -> ()  [unwired: 2 in, 2 out]
            n639 = call "Elapsed Time57"("Time Target (s)"=w1322) -> ("Elapsed Time (s)"=w1321:dbl)  [unwired: 11 in, 7 out]
          }
          frame 13 {
            n640 = property on="Current Task time" class="Slide (strict)"("Scale.Maximum"=w1324) -> ()  [unwired: 2 in, 2 out]
            n641 = call "Elapsed Time124"("Time Target (s)"=w1324) -> ("Elapsed Time (s)"=w1323:dbl)  [unwired: 11 in, 7 out]
          }
          frame 0, Default {
            n642 = property on="Current Task time" class="Slide (strict)"("Scale.Maximum"=w1326) -> ()  [unwired: 2 in, 2 out]
            n643 = call "Elapsed Time125"("Time Target (s)"=w1326) -> ("Elapsed Time (s)"=w1325:dbl)  [unwired: 11 in, 7 out]
          }
        }
      }
      frame 7 {
        w1381 = 240.0  # Routine Time
        # "Routine 5: In car seat"
        n644 = property on="Total Routine Time" class="Slide (strict)"("Scale.Maximum"=w1381) -> ()  [unwired: 2 in, 2 out]
        n645 = call "Elapsed Time8"("Time Target (s)"=w1381, "Reset"=FALSE) -> ("Get Start Time (s)"=w1379:dbl, "Elapsed Time (s)"=w1373:dbl, "Time has Elapsed"=w1382:bool)  [unwired: 10 in, 5 out]
        "#5" <- w1382
        n646 = Seconds To Date/Time(time stamp (now)=w1379) -> (date time rec=w1380:T2)  [unwired: 1 in]
        n647 = Not(x=w1382) -> (.not. x?=w1385:bool)
        n648 = script code="t = [0,120,124,130,134,140,144,150,154,160,164,170,174,...\n       180,180.75,181.5,182.25,183,183.75,184.5,185.25,186,186.75,187.5,188.25,189,189.75,190.5,191.25,192,...\n       192.75,193.5,194.25,195,195.75,196.5,197.25,198,198.75,199.5,200.25,201,201.75,202.5,203.25,204,204.75,205.5,...\n       206.25,207,207.75,208.5,209.25,210,...\n        240];\n\nevent = [0,1,2,1,2,1,2,1,2,1,2,1,2,...\n               3,4,3,4,3,4,3,4,3,4,3,4,3,4,3,4,3,4,3,4,3,4,3,4,3,4,3,4,3,4,3,4,3,4,3,4,3,4,3,4,0,...\n               14];\n\nfor i = 2:length(t)\n    if ((x>=t(i-1)) &&  (x<t(i)))\n        y = event(i-1);\n        yNext = event(i);\n        dt = t(i) - t(i-1);\n        break;\n    end\nend"("x"=w1373) -> ("y"=w1376:dbl, "dt"=w1377:dbl, "yNext"=w1378:dbl)  [unwired: 1 in, 1 out]
        n649 = case shown="True" w1385 {
          tunnel: [w1441 w1453] -> w1384
          frame False {
            n650 = flat-sequence {
              tunnel: [w1449] -> w1441
              frame #0 {
                n651 = local write "Buffer"(FALSE ("Buffer")) -> ()
                n652 = local write "Play/Stop"(FALSE ("PlayInstr")) -> ()
              }
              frame #1 {
                n653 = local write "Output"(0 ("Output")) -> ()
                n654 = local write "Save"(TRUE ("Save")) -> ()
              }
              frame #2 {
                n655 = Wait (ms)(milliseconds to wait=u32 500) -> ()  [unwired: 1 out]
              }
              frame #3 {
                n656 = local write "Flush"(TRUE ("Flush")) -> ()
              }
              frame #4 {
                w1448 = u16 0 items=["No sound", "Demo deep breathing", "Demo fast shallow breathing", "Demo slow shallow breathing", "Demo breath hold", "Demo cough/ laugh", "Demo abdomen movement", "Calibration", "Routine 1", "Routine 3", "Routine 4/5/7", "Calm music"] ("Play sound")
                w1449 = enum16{"Default"}."Default"
                n657 = local write "Flush"(FALSE ("Flush")) -> ()
                n658 = local write "Save"(FALSE ("Save")) -> ()
                n659 = local write "Play sound"(w1448) -> ()
                n660 = local write "Routine"(w1449) -> ()
              }
            }
          }
          frame True {
            w1452 = u16 12 items=["No sound", "Demo normal breathing", "Demo deep breathing", "Demo fast shallow breathing", "Demo breath hold", "Demo cough", "Demo abdomen movement", "Calibration", "Routine 1", "(2a)Calm music", "(2b)Stress test", "Routine 3/4", "Routine 5"] ("Play sound")
            n661 = local write "Play sound"(w1452) -> ()
            n662 = flat-sequence {
              tunnel: [T4."Routine 5"] -> w1453
              frame #0 {
                n663 = local write "Output"(1 ("Open")) -> ()
                n664 = local write "Play/Stop"(TRUE ("PlayInstr")) -> ()
              }
              frame #1 {
                n665 = local write "Buffer"(TRUE ("Buffer")) -> ()
              }
              frame #2 {
              }
            }
          }
        }
        n666 = case shown="0, Default" w1376 {
          tunnel: ["\nPerform normal breathing." "Inhale a slow deep breath." "\nExhale slowly." "Quick inhale.\n\n\n\nIf you cannot sustain for long, resume normal breathing." "\nQuick exhale.\n\n\nIf you cannot sustain for long, resume normal breathing." "Slow shallow inhale.\n\n\n\nIf you cannot sustain for long, resume normal breathing." "\nSlow exhale.\n\n\nIf you cannot sustain for long, resume normal breathing." "Exhale the current breath  and HOLD.\n\n\nIf you cannot sustain for long, resume normal breathing." "Perform voluntary coughing \n" "Perform voluntary laugh\n\n" "Read aloud the following text in between the lines:\n-----------------------------------------------------------------------\nFour score and seven years ago our fathers brought forth on this continent, a new nation, conceived in Liberty, and dedicated to the proposition that all men are created equal… That this nation, under God, shall have a new birth of freedom-and that government of the people, by the people, for the people, shall not perish from the earth.\n\n-----------------------------------------------------------------------\nWhen finished, take a deep breath and open mouth say \"Ah\" (like doctor checking your throat).\nPerform normal breathing until next instruction." "Exhale current breath and HOLD. Push abdomen inwards." "Relax abdomen back to normal and keep holding breath."] -> w1374
          frame 0, Default {
          }
          frame 1 {
          }
          frame 2 {
          }
          frame 3 {
          }
          frame 4 {
          }
          frame 5 {
          }
          frame 6 {
          }
          frame 7 {
          }
          frame 8 {
          }
          frame 9 {
          }
          frame 10 {
          }
          frame 12 {
          }
          frame 13 {
          }
        }
        n667 = case shown="0, Default" w1378 {
          tunnel: ["\nPerform normal breathing." "Inhale a slow deep breath." "\nExhale slowly." "Quick inhale.\n\n\n\nIf you cannot sustain for long, resume normal breathing." "\nQuick exhale.\n\n\nIf you cannot sustain for long, resume normal breathing." "Slow shallow inhale.\n\n\n\nIf you cannot sustain for long, resume normal breathing." "\nSlow exhale.\n\n\nIf you cannot sustain for long, resume normal breathing." "Exhale the current breath  and HOLD.\n\n\nIf you cannot sustain for long, resume normal breathing." "Perform voluntary coughing \n" "Perform voluntary laugh\n\n" "Read aloud the following text in between the lines:\n-----------------------------------------------------------------------\nFour score and ...\n-----------------------------------------------------------------------\nWhen finished, take a deep breath and open mouth say \"Ah\" (like doctor checking your throat).\nPerform normal breathing until next instruction." "Exhale current breath and HOLD. Push abdomen inwards." "Relax abdomen back to normal and keep holding breath." "Study Completed!"] -> w1372
          frame 0, Default {
          }
          frame 1 {
          }
          frame 2 {
          }
          frame 3 {
          }
          frame 4 {
          }
          frame 5 {
          }
          frame 6 {
          }
          frame 7 {
          }
          frame 8 {
          }
          frame 9 {
          }
          frame 10 {
          }
          frame 12 {
          }
          frame 13 {
          }
          frame 14 {
          }
        }
        n668 = case shown="0, Default" w1376 {
          tunnel: w1377 -> [w1387 w1389 w1391 w1393 w1395 w1397 w1399 w1401 w1403 w1405 w1407 w1409 w1411 w1413]
          tunnel: [w1386 w1388 w1390 w1392 w1394 w1396 w1398 w1400 w1402 w1404 w1406 w1408 w1410 w1412] -> w1375
          frame 1 {
            n669 = property on="Current Task time" class="Slide (strict)"("Scale.Maximum"=w1387) -> ()  [unwired: 2 in, 2 out]
            n670 = call "Elapsed Time58"("Time Target (s)"=w1387) -> ("Elapsed Time (s)"=w1386:dbl)  [unwired: 11 in, 7 out]
          }
          frame 2 {
            n671 = property on="Current Task time" class="Slide (strict)"("Scale.Maximum"=w1389) -> ()  [unwired: 2 in, 2 out]
            n672 = call "Elapsed Time59"("Time Target (s)"=w1389) -> ("Elapsed Time (s)"=w1388:dbl)  [unwired: 11 in, 7 out]
          }
          frame 3 {
            n673 = property on="Current Task time" class="Slide (strict)"("Scale.Maximum"=w1391) -> ()  [unwired: 2 in, 2 out]
            n674 = call "Elapsed Time60"("Time Target (s)"=w1391) -> ("Elapsed Time (s)"=w1390:dbl)  [unwired: 11 in, 7 out]
          }
          frame 4 {
            n675 = property on="Current Task time" class="Slide (strict)"("Scale.Maximum"=w1393) -> ()  [unwired: 2 in, 2 out]
            n676 = call "Elapsed Time61"("Time Target (s)"=w1393) -> ("Elapsed Time (s)"=w1392:dbl)  [unwired: 11 in, 7 out]
          }
          frame 5 {
            n677 = property on="Current Task time" class="Slide (strict)"("Scale.Maximum"=w1395) -> ()  [unwired: 2 in, 2 out]
            n678 = call "Elapsed Time62"("Time Target (s)"=w1395) -> ("Elapsed Time (s)"=w1394:dbl)  [unwired: 11 in, 7 out]
          }
          frame 6 {
            n679 = property on="Current Task time" class="Slide (strict)"("Scale.Maximum"=w1397) -> ()  [unwired: 2 in, 2 out]
            n680 = call "Elapsed Time63"("Time Target (s)"=w1397) -> ("Elapsed Time (s)"=w1396:dbl)  [unwired: 11 in, 7 out]
          }
          frame 7 {
            n681 = property on="Current Task time" class="Slide (strict)"("Scale.Maximum"=w1399) -> ()  [unwired: 2 in, 2 out]
            n682 = call "Elapsed Time64"("Time Target (s)"=w1399) -> ("Elapsed Time (s)"=w1398:dbl)  [unwired: 11 in, 7 out]
          }
          frame 8 {
            n683 = property on="Current Task time" class="Slide (strict)"("Scale.Maximum"=w1401) -> ()  [unwired: 2 in, 2 out]
            n684 = call "Elapsed Time65"("Time Target (s)"=w1401) -> ("Elapsed Time (s)"=w1400:dbl)  [unwired: 11 in, 7 out]
          }
          frame 9 {
            n685 = property on="Current Task time" class="Slide (strict)"("Scale.Maximum"=w1403) -> ()  [unwired: 2 in, 2 out]
            n686 = call "Elapsed Time66"("Time Target (s)"=w1403) -> ("Elapsed Time (s)"=w1402:dbl)  [unwired: 11 in, 7 out]
          }
          frame 10 {
            n687 = property on="Current Task time" class="Slide (strict)"("Scale.Maximum"=w1405) -> ()  [unwired: 2 in, 2 out]
            n688 = call "Elapsed Time67"("Time Target (s)"=w1405) -> ("Elapsed Time (s)"=w1404:dbl)  [unwired: 11 in, 7 out]
          }
          frame 11 {
            n689 = property on="Current Task time" class="Slide (strict)"("Scale.Maximum"=w1407) -> ()  [unwired: 2 in, 2 out]
            n690 = call "Elapsed Time68"("Time Target (s)"=w1407) -> ("Elapsed Time (s)"=w1406:dbl)  [unwired: 11 in, 7 out]
          }
          frame 12 {
            n691 = property on="Current Task time" class="Slide (strict)"("Scale.Maximum"=w1409) -> ()  [unwired: 2 in, 2 out]
            n692 = call "Elapsed Time69"("Time Target (s)"=w1409) -> ("Elapsed Time (s)"=w1408:dbl)  [unwired: 11 in, 7 out]
          }
          frame 13 {
            n693 = property on="Current Task time" class="Slide (strict)"("Scale.Maximum"=w1411) -> ()  [unwired: 2 in, 2 out]
            n694 = call "Elapsed Time126"("Time Target (s)"=w1411) -> ("Elapsed Time (s)"=w1410:dbl)  [unwired: 11 in, 7 out]
          }
          frame 0, Default {
            n695 = property on="Current Task time" class="Slide (strict)"("Scale.Maximum"=w1413) -> ()  [unwired: 2 in, 2 out]
            n696 = call "Elapsed Time127"("Time Target (s)"=w1413) -> ("Elapsed Time (s)"=w1412:dbl)  [unwired: 11 in, 7 out]
          }
        }
      }
      frame 8 {
        w1467 = 35.0  # Routine Time
        # "Calibration Routine 1"
        n697 = property on="Total Routine Time" class="Slide (strict)"("Scale.Maximum"=w1467) -> ()  [unwired: 2 in, 2 out]
        n698 = call "Elapsed Time71"("Time Target (s)"=w1467, "Auto Reset"=FALSE ("Timer Reset")) -> ("Get Start Time (s)"=w1465:dbl, "Elapsed Time (s)"=w1461:dbl, "Time has Elapsed"=w1468:bool)  [unwired: 10 in, 5 out]
        "Calib 1" <- w1468
        n699 = Seconds To Date/Time(time stamp (now)=w1465) -> (date time rec=w1466:T2)  [unwired: 1 in]
        n700 = Not(x=w1468) -> (.not. x?=w1471:bool)
        n701 = script code="t = [0,20,23,27.5,30.5,35];\n\nevent = [0,1,2,1,2,14];\n\nfor i = 2:length(t)\n    if ((x>=t(i-1)) &&  (x<t(i)))\n        y = event(i-1);\n        yNext = event(i);\n        dt = t(i) - t(i-1);\n        break;\n    end\nend"("x"=w1461) -> ("y"=w1462:dbl, "dt"=w1463:dbl, "yNext"=w1464:dbl)  [unwired: 1 in, 1 out]
        n702 = case shown="True" w1471 {
          tunnel: [w1510 w1522] -> w1470
          frame False {
            n703 = flat-sequence {
              tunnel: [w1518] -> w1510
              frame #0 {
                n704 = local write "Buffer"(FALSE ("Buffer")) -> ()
                n705 = local write "Play/Stop"(FALSE ("Play\nCalibration")) -> ()
              }
              frame #1 {
                n706 = local write "Output"(0 ("Output")) -> ()
                n707 = local write "Save"(TRUE ("Save")) -> ()
              }
              frame #2 {
                n708 = Wait (ms)(milliseconds to wait=u32 500) -> ()  [unwired: 1 out]
              }
              frame #3 {
                n709 = local write "Flush"(TRUE ("Flush")) -> ()
              }
              frame #4 {
                w1517 = u16 0 items=["No sound", "Demo deep breathing", "Demo fast shallow breathing", "Demo slow shallow breathing", "Demo breath hold", "Demo cough/ laugh", "Demo abdomen movement", "Calibration", "Routine 1", "Routine 3", "Routine 4/5/7", "Calm music"] ("Play sound")
                w1518 = enum16{"Default"}."Default"
                n710 = local write "Flush"(FALSE ("Flush")) -> ()
                n711 = local write "Save"(FALSE ("Save")) -> ()
                n712 = local write "Routine"(w1518) -> ()
                n713 = local write "Play sound"(w1517) -> ()
              }
            }
          }
          frame True {
            w1521 = u16 7 items=["No sound", "Demo normal breathing", "Demo deep breathing", "Demo fast shallow breathing", "Demo breath hold", "Demo cough", "Demo abdomen movement", "Calibration", "Routine 1", "(2a)Calm music", "(2b)Stress test", "Routine 3/4", "Routine 5", ""] ("Play sound")
            n714 = local write "Play sound"(w1521) -> ()
            n715 = flat-sequence {
              tunnel: [T4."Calib1"] -> w1522
              frame #0 {
                n716 = local write "Play/Stop"(TRUE ("Play\nCalibration")) -> ()
                n717 = local write "Output"(1 ("Open")) -> ()
              }
              frame #1 {
                n718 = local write "Buffer"(TRUE ("Buffer")) -> ()
              }
              frame #2 {
              }
            }
          }
        }
        n719 = case shown="0, Default" w1462 {
          tunnel: ["\nPerform normal breathing." "Inhale a slow deep breath." "\nExhale slowly." "Quick inhale.\n\n\n\nIf you cannot sustain for long, resume normal breathing." "\nQuick exhale.\n\n\nIf you cannot sustain for long, resume normal breathing." "Slow shallow inhale.\n\n\n\nIf you cannot sustain for long, resume normal breathing." "\nSlow exhale.\n\n\nIf you cannot sustain for long, resume normal breathing." "Exhale the current breath  and HOLD.\n\n\nIf you cannot sustain for long, resume normal breathing." "Perform voluntary coughing \n" "Perform voluntary laugh\n\n" "Read aloud the following text in between the lines:\n-----------------------------------------------------------------------\nFour score and seven years ago our fathers brought forth on this continent, a new nation, conceived in Liberty, and dedicated to the proposition that all men are created equal… That this nation, under God, shall have a new birth of freedom-and that government of the people, by the people, for the people, shall not perish from the earth.\n\n-----------------------------------------------------------------------\nWhen finished, take a deep breath and open mouth say \"Ah\" (like doctor checking your throat).\nPerform normal breathing until next instruction." "Exhale current breath and HOLD. Push abdomen inwards." "Relax abdomen back to normal and keep holding breath."] -> w1460
          frame 0, Default {
          }
          frame 1 {
          }
          frame 2 {
          }
          frame 3 {
          }
          frame 4 {
          }
          frame 5 {
          }
          frame 6 {
          }
          frame 7 {
          }
          frame 8 {
          }
          frame 9 {
          }
          frame 10 {
          }
          frame 12 {
          }
          frame 13 {
          }
        }
        n720 = case shown="14" w1464 {
          tunnel: ["\nPerform normal breathing." "Inhale a slow deep breath." "\nExhale slowly." "Quick inhale.\n\n\n\nIf you cannot sustain for long, resume normal breathing." "\nQuick exhale.\n\n\nIf you cannot sustain for long, resume normal breathing." "Slow shallow inhale.\n\n\n\nIf you cannot sustain for long, resume normal breathing." "\nSlow exhale.\n\n\nIf you cannot sustain for long, resume normal breathing." "Exhale the current breath  and HOLD.\n\n\nIf you cannot sustain for long, resume normal breathing." "Perform voluntary coughing \n" "Perform voluntary laugh\n\n" "Read aloud the following text in between the lines:\n-----------------------------------------------------------------------\nFour score and ...\n-----------------------------------------------------------------------\nWhen finished, take a deep breath and open mouth say \"Ah\" (like doctor checking your throat).\nPerform normal breathing until next instruction." "Exhale current breath and HOLD. Push abdomen inwards." "Relax abdomen back to normal and keep holding breath." "Wait for next routine. Please do not move."] -> w1458
          frame 0, Default {
          }
          frame 1 {
          }
          frame 2 {
          }
          frame 3 {
          }
          frame 4 {
          }
          frame 5 {
          }
          frame 6 {
          }
          frame 7 {
          }
          frame 8 {
          }
          frame 9 {
          }
          frame 10 {
          }
          frame 12 {
          }
          frame 13 {
          }
          frame 14 {
          }
        }
        n721 = case shown="0, Default" w1462 {
          tunnel: w1463 -> [w1474 w1476 w1478 w1480 w1482]
          tunnel: [w1473 w1475 w1477 w1479 w1481] -> w1459
          frame 1 {
            n722 = property on="Current Task time" class="Slide (strict)"("Scale.Maximum"=w1474) -> ()  [unwired: 2 in, 2 out]
            n723 = call "Elapsed Time72"("Time Target (s)"=w1474) -> ("Elapsed Time (s)"=w1473:dbl)  [unwired: 11 in, 7 out]
          }
          frame 2 {
            n724 = property on="Current Task time" class="Slide (strict)"("Scale.Maximum"=w1476) -> ()  [unwired: 2 in, 2 out]
            n725 = call "Elapsed Time73"("Time Target (s)"=w1476) -> ("Elapsed Time (s)"=w1475:dbl)  [unwired: 11 in, 7 out]
          }
          frame 3 {
            n726 = property on="Current Task time" class="Slide (strict)"("Scale.Maximum"=w1478) -> ()  [unwired: 2 in, 2 out]
            n727 = call "Elapsed Time74"("Time Target (s)"=w1478) -> ("Elapsed Time (s)"=w1477:dbl)  [unwired: 11 in, 7 out]
          }
          frame 4 {
            n728 = property on="Current Task time" class="Slide (strict)"("Scale.Maximum"=w1480) -> ()  [unwired: 2 in, 2 out]
            n729 = call "Elapsed Time75"("Time Target (s)"=w1480) -> ("Elapsed Time (s)"=w1479:dbl)  [unwired: 11 in, 7 out]
          }
          frame 0, Default {
            n730 = property on="Current Task time" class="Slide (strict)"("Scale.Maximum"=w1482) -> ()  [unwired: 2 in, 2 out]
            n731 = call "Elapsed Time134"("Time Target (s)"=w1482) -> ("Elapsed Time (s)"=w1481:dbl)  [unwired: 11 in, 7 out]
          }
        }
      }
      frame 9 {
        w1536 = 35.0  # Routine Time
        # "Calibration Routine 3"
        n732 = property on="Total Routine Time" class="Slide (strict)"("Scale.Maximum"=w1536) -> ()  [unwired: 2 in, 2 out]
        n733 = call "Elapsed Time76"("Time Target (s)"=w1536, "Auto Reset"=FALSE ("Timer Reset")) -> ("Get Start Time (s)"=w1534:dbl, "Elapsed Time (s)"=w1530:dbl, "Time has Elapsed"=w1537:bool)  [unwired: 10 in, 5 out]
        "Calib 3" <- w1537
        n734 = Seconds To Date/Time(time stamp (now)=w1534) -> (date time rec=w1535:T2)  [unwired: 1 in]
        n735 = Not(x=w1537) -> (.not. x?=w1540:bool)
        n736 = script code="t = [0,20,23,27.5,30.5,35];\n\nevent = [0,1,2,1,2,14];\n\nfor i = 2:length(t)\n    if ((x>=t(i-1)) &&  (x<t(i)))\n        y = event(i-1);\n        yNext = event(i);\n        dt = t(i) - t(i-1);\n        break;\n    end\nend"("x"=w1530) -> ("y"=w1531:dbl, "dt"=w1532:dbl, "yNext"=w1533:dbl)  [unwired: 1 in, 1 out]
        n737 = case shown="True" w1540 {
          tunnel: [w1579 w1591] -> w1539
          frame False {
            n738 = flat-sequence {
              tunnel: [w1587] -> w1579
              frame #0 {
                n739 = local write "Buffer"(FALSE ("Buffer")) -> ()
                n740 = local write "Play/Stop"(FALSE ("Play\nCalibration")) -> ()
              }
              frame #1 {
                n741 = local write "Output"(0 ("Output")) -> ()
                n742 = local write "Save"(TRUE ("Save")) -> ()
              }
              frame #2 {
                n743 = Wait (ms)(milliseconds to wait=u32 500) -> ()  [unwired: 1 out]
              }
              frame #3 {
                n744 = local write "Flush"(TRUE ("Flush")) -> ()
              }
              frame #4 {
                w1586 = u16 0 items=["No sound", "Demo deep breathing", "Demo fast shallow breathing", "Demo slow shallow breathing", "Demo breath hold", "Demo cough/ laugh", "Demo abdomen movement", "Calibration", "Routine 1", "Routine 3", "Routine 4/5/7", "Calm music"] ("Play sound")
                w1587 = enum16{"Default"}."Default"
                n745 = local write "Flush"(FALSE ("Flush")) -> ()
                n746 = local write "Save"(FALSE ("Save")) -> ()
                n747 = local write "Routine"(w1587) -> ()
                n748 = local write "Play sound"(w1586) -> ()
              }
            }
          }
          frame True {
            w1590 = u16 7 items=["No sound", "Demo normal breathing", "Demo deep breathing", "Demo fast shallow breathing", "Demo breath hold", "Demo cough", "Demo abdomen movement", "Calibration", "Routine 1", "(2a)Calm music", "(2b)Stress test", "Routine 3/4", "Routine 5", ""] ("Play sound")
            n749 = local write "Play sound"(w1590) -> ()
            n750 = flat-sequence {
              tunnel: [T4."Calib3"] -> w1591
              frame #0 {
                n751 = local write "Output"(1 ("Open")) -> ()
                n752 = local write "Play/Stop"(TRUE ("Play\nCalibration")) -> ()
              }
              frame #1 {
                n753 = local write "Buffer"(TRUE ("Buffer")) -> ()
              }
              frame #2 {
              }
            }
          }
        }
        n754 = case shown="0, Default" w1531 {
          tunnel: ["\nPerform normal breathing." "Inhale a slow deep breath." "\nExhale slowly." "Quick inhale.\n\n\n\nIf you cannot sustain for long, resume normal breathing." "\nQuick exhale.\n\n\nIf you cannot sustain for long, resume normal breathing." "Slow shallow inhale.\n\n\n\nIf you cannot sustain for long, resume normal breathing." "\nSlow exhale.\n\n\nIf you cannot sustain for long, resume normal breathing." "Exhale the current breath  and HOLD.\n\n\nIf you cannot sustain for long, resume normal breathing." "Perform voluntary coughing \n" "Perform voluntary laugh\n\n" "Read aloud the following text in between the lines:\n-----------------------------------------------------------------------\nFour score and seven years ago our fathers brought forth on this continent, a new nation, conceived in Liberty, and dedicated to the proposition that all men are created equal… That this nation, under God, shall have a new birth of freedom-and that government of the people, by the people, for the people, shall not perish from the earth.\n\n-----------------------------------------------------------------------\nWhen finished, take a deep breath and open mouth say \"Ah\" (like doctor checking your throat).\nPerform normal breathing until next instruction." "Exhale current breath and HOLD. Push abdomen inwards." "Relax abdomen back to normal and keep holding breath."] -> w1529
          frame 0, Default {
          }
          frame 1 {
          }
          frame 2 {
          }
          frame 3 {
          }
          frame 4 {
          }
          frame 5 {
          }
          frame 6 {
          }
          frame 7 {
          }
          frame 8 {
          }
          frame 9 {
          }
          frame 10 {
          }
          frame 12 {
          }
          frame 13 {
          }
        }
        n755 = case shown="14" w1533 {
          tunnel: ["\nPerform normal breathing." "Inhale a slow deep breath." "\nExhale slowly." "Quick inhale.\n\n\n\nIf you cannot sustain for long, resume normal breathing." "\nQuick exhale.\n\n\nIf you cannot sustain for long, resume normal breathing." "Slow shallow inhale.\n\n\n\nIf you cannot sustain for long, resume normal breathing." "\nSlow exhale.\n\n\nIf you cannot sustain for long, resume normal breathing." "Exhale the current breath  and HOLD.\n\n\nIf you cannot sustain for long, resume normal breathing." "Perform voluntary coughing \n" "Perform voluntary laugh\n\n" "Read aloud the following text in between the lines:\n-----------------------------------------------------------------------\nFour score and ...\n-----------------------------------------------------------------------\nWhen finished, take a deep breath and open mouth say \"Ah\" (like doctor checking your throat).\nPerform normal breathing until next instruction." "Exhale current breath and HOLD. Push abdomen inwards." "Relax abdomen back to normal and keep holding breath." "Wait for next routine. Please do not move."] -> w1527
          frame 0, Default {
          }
          frame 1 {
          }
          frame 2 {
          }
          frame 3 {
          }
          frame 4 {
          }
          frame 5 {
          }
          frame 6 {
          }
          frame 7 {
          }
          frame 8 {
          }
          frame 9 {
          }
          frame 10 {
          }
          frame 12 {
          }
          frame 13 {
          }
          frame 14 {
          }
        }
        n756 = case shown="0, Default" w1531 {
          tunnel: w1532 -> [w1543 w1545 w1547 w1549 w1551]
          tunnel: [w1542 w1544 w1546 w1548 w1550] -> w1528
          frame 1 {
            n757 = property on="Current Task time" class="Slide (strict)"("Scale.Maximum"=w1543) -> ()  [unwired: 2 in, 2 out]
            n758 = call "Elapsed Time77"("Time Target (s)"=w1543) -> ("Elapsed Time (s)"=w1542:dbl)  [unwired: 11 in, 7 out]
          }
          frame 2 {
            n759 = property on="Current Task time" class="Slide (strict)"("Scale.Maximum"=w1545) -> ()  [unwired: 2 in, 2 out]
            n760 = call "Elapsed Time78"("Time Target (s)"=w1545) -> ("Elapsed Time (s)"=w1544:dbl)  [unwired: 11 in, 7 out]
          }
          frame 3 {
            n761 = property on="Current Task time" class="Slide (strict)"("Scale.Maximum"=w1547) -> ()  [unwired: 2 in, 2 out]
            n762 = call "Elapsed Time79"("Time Target (s)"=w1547) -> ("Elapsed Time (s)"=w1546:dbl)  [unwired: 11 in, 7 out]
          }
          frame 4 {
            n763 = property on="Current Task time" class="Slide (strict)"("Scale.Maximum"=w1549) -> ()  [unwired: 2 in, 2 out]
            n764 = call "Elapsed Time80"("Time Target (s)"=w1549) -> ("Elapsed Time (s)"=w1548:dbl)  [unwired: 11 in, 7 out]
          }
          frame 0, Default {
            n765 = property on="Current Task time" class="Slide (strict)"("Scale.Maximum"=w1551) -> ()  [unwired: 2 in, 2 out]
            n766 = call "Elapsed Time81"("Time Target (s)"=w1551) -> ("Elapsed Time (s)"=w1550:dbl)  [unwired: 11 in, 7 out]
          }
        }
      }
      frame 10 {
        w1605 = 35.0  # Routine Time
        # "Calibration 4"
        n767 = property on="Total Routine Time" class="Slide (strict)"("Scale.Maximum"=w1605) -> ()  [unwired: 2 in, 2 out]
        n768 = call "Elapsed Time82"("Time Target (s)"=w1605, "Auto Reset"=FALSE ("Timer Reset")) -> ("Get Start Time (s)"=w1603:dbl, "Elapsed Time (s)"=w1599:dbl, "Time has Elapsed"=w1606:bool)  [unwired: 10 in, 5 out]
        "Calib 4" <- w1606
        n769 = Seconds To Date/Time(time stamp (now)=w1603) -> (date time rec=w1604:T2)  [unwired: 1 in]
        n770 = Not(x=w1606) -> (.not. x?=w1609:bool)
        n771 = script code="t = [0,20,23,27.5,30.5,35];\n\nevent = [0,1,2,1,2,14];\n\nfor i = 2:length(t)\n    if ((x>=t(i-1)) &&  (x<t(i)))\n        y = event(i-1);\n        yNext = event(i);\n        dt = t(i) - t(i-1);\n        break;\n    end\nend"("x"=w1599) -> ("y"=w1600:dbl, "dt"=w1601:dbl, "yNext"=w1602:dbl)  [unwired: 1 in, 1 out]
        n772 = case shown="True" w1609 {
          tunnel: [w1648 w1660] -> w1608
          frame False {
            n773 = flat-sequence {
              tunnel: [w1656] -> w1648
              frame #0 {
                n774 = local write "Buffer"(FALSE ("Buffer")) -> ()
                n775 = local write "Play/Stop"(FALSE ("Play\nCalibration")) -> ()
              }
              frame #1 {
                n776 = local write "Output"(0 ("Output")) -> ()
                n777 = local write "Save"(TRUE ("Save")) -> ()
              }
              frame #2 {
                n778 = Wait (ms)(milliseconds to wait=u32 500) -> ()  [unwired: 1 out]
              }
              frame #3 {
                n779 = local write "Flush"(TRUE ("Flush")) -> ()
              }
              frame #4 {
                w1655 = u16 0 items=["No sound", "Demo deep breathing", "Demo fast shallow breathing", "Demo slow shallow breathing", "Demo breath hold", "Demo cough/ laugh", "Demo abdomen movement", "Calibration", "Routine 1", "Routine 3", "Routine 4/5/7", "Calm music"] ("Play sound")
                w1656 = enum16{"Default", ""}."Default"
                n780 = local write "Flush"(FALSE ("Flush")) -> ()
                n781 = local write "Save"(FALSE ("Save")) -> ()
                n782 = local write "Routine"(w1656) -> ()
                n783 = local write "Play sound"(w1655) -> ()
              }
            }
          }
          frame True {
            w1659 = u16 7 items=["No sound", "Demo normal breathing", "Demo deep breathing", "Demo fast shallow breathing", "Demo breath hold", "Demo cough", "Demo abdomen movement", "Calibration", "Routine 1", "(2a)Calm music", "(2b)Stress test", "Routine 3/4", "Routine 5", ""] ("Play sound")
            n784 = local write "Play sound"(w1659) -> ()
            n785 = flat-sequence {
              tunnel: [T4."Calib4"] -> w1660
              frame #0 {
                n786 = local write "Output"(1 ("Open")) -> ()
                n787 = local write "Play/Stop"(TRUE ("Play\nCalibration")) -> ()
              }
              frame #1 {
                n788 = local write "Buffer"(TRUE ("Buffer")) -> ()
              }
              frame #2 {
              }
            }
          }
        }
        n789 = case shown="0, Default" w1600 {
          tunnel: ["\nPerform normal breathing." "Inhale a slow deep breath." "\nExhale slowly." "Quick inhale.\n\n\n\nIf you cannot sustain for long, resume normal breathing." "\nQuick exhale.\n\n\nIf you cannot sustain for long, resume normal breathing." "Slow shallow inhale.\n\n\n\nIf you cannot sustain for long, resume normal breathing." "\nSlow exhale.\n\n\nIf you cannot sustain for long, resume normal breathing." "Exhale the current breath  and HOLD.\n\n\nIf you cannot sustain for long, resume normal breathing." "Perform voluntary coughing \n" "Perform voluntary laugh\n\n" "Read aloud the following text in between the lines:\n-----------------------------------------------------------------------\nFour score and seven years ago our fathers brought forth on this continent, a new nation, conceived in Liberty, and dedicated to the proposition that all men are created equal… That this nation, under God, shall have a new birth of freedom-and that government of the people, by the people, for the people, shall not perish from the earth.\n\n-----------------------------------------------------------------------\nWhen finished, take a deep breath and open mouth say \"Ah\" (like doctor checking your throat).\nPerform normal breathing until next instruction." "Exhale current breath and HOLD. Push abdomen inwards." "Relax abdomen back to normal and keep holding breath."] -> w1598
          frame 0, Default {
          }
          frame 1 {
          }
          frame 2 {
          }
          frame 3 {
          }
          frame 4 {
          }
          frame 5 {
          }
          frame 6 {
          }
          frame 7 {
          }
          frame 8 {
          }
          frame 9 {
          }
          frame 10 {
          }
          frame 12 {
          }
          frame 13 {
          }
        }
        n790 = case shown="14" w1602 {
          tunnel: ["\nPerform normal breathing." "Inhale a slow deep breath." "\nExhale slowly." "Quick inhale.\n\n\n\nIf you cannot sustain for long, resume normal breathing." "\nQuick exhale.\n\n\nIf you cannot sustain for long, resume normal breathing." "Slow shallow inhale.\n\n\n\nIf you cannot sustain for long, resume normal breathing." "\nSlow exhale.\n\n\nIf you cannot sustain for long, resume normal breathing." "Exhale the current breath  and HOLD.\n\n\nIf you cannot sustain for long, resume normal breathing." "Perform voluntary coughing \n" "Perform voluntary laugh\n\n" "Read aloud the following text in between the lines:\n-----------------------------------------------------------------------\nFour score and ...\n-----------------------------------------------------------------------\nWhen finished, take a deep breath and open mouth say \"Ah\" (like doctor checking your throat).\nPerform normal breathing until next instruction." "Exhale current breath and HOLD. Push abdomen inwards." "Relax abdomen back to normal and keep holding breath." "Wait for next routine. Please do not move."] -> w1596
          frame 0, Default {
          }
          frame 1 {
          }
          frame 2 {
          }
          frame 3 {
          }
          frame 4 {
          }
          frame 5 {
          }
          frame 6 {
          }
          frame 7 {
          }
          frame 8 {
          }
          frame 9 {
          }
          frame 10 {
          }
          frame 12 {
          }
          frame 13 {
          }
          frame 14 {
          }
        }
        n791 = case shown="0, Default" w1600 {
          tunnel: w1601 -> [w1612 w1614 w1616 w1618 w1620]
          tunnel: [w1611 w1613 w1615 w1617 w1619] -> w1597
          frame 1 {
            n792 = property on="Current Task time" class="Slide (strict)"("Scale.Maximum"=w1612) -> ()  [unwired: 2 in, 2 out]
            n793 = call "Elapsed Time83"("Time Target (s)"=w1612) -> ("Elapsed Time (s)"=w1611:dbl)  [unwired: 11 in, 7 out]
          }
          frame 2 {
            n794 = property on="Current Task time" class="Slide (strict)"("Scale.Maximum"=w1614) -> ()  [unwired: 2 in, 2 out]
            n795 = call "Elapsed Time84"("Time Target (s)"=w1614) -> ("Elapsed Time (s)"=w1613:dbl)  [unwired: 11 in, 7 out]
          }
          frame 3 {
            n796 = property on="Current Task time" class="Slide (strict)"("Scale.Maximum"=w1616) -> ()  [unwired: 2 in, 2 out]
            n797 = call "Elapsed Time85"("Time Target (s)"=w1616) -> ("Elapsed Time (s)"=w1615:dbl)  [unwired: 11 in, 7 out]
          }
          frame 4 {
            n798 = property on="Current Task time" class="Slide (strict)"("Scale.Maximum"=w1618) -> ()  [unwired: 2 in, 2 out]
            n799 = call "Elapsed Time86"("Time Target (s)"=w1618) -> ("Elapsed Time (s)"=w1617:dbl)  [unwired: 11 in, 7 out]
          }
          frame 0, Default {
            n800 = property on="Current Task time" class="Slide (strict)"("Scale.Maximum"=w1620) -> ()  [unwired: 2 in, 2 out]
            n801 = call "Elapsed Time87"("Time Target (s)"=w1620) -> ("Elapsed Time (s)"=w1619:dbl)  [unwired: 11 in, 7 out]
          }
        }
      }
      frame 11 {
        w1674 = 35.0  # Routine Time
        # "Calibration Routine 5"
        n802 = property on="Total Routine Time" class="Slide (strict)"("Scale.Maximum"=w1674) -> ()  [unwired: 2 in, 2 out]
        n803 = call "Elapsed Time88"("Time Target (s)"=w1674, "Auto Reset"=FALSE ("Timer Reset")) -> ("Get Start Time (s)"=w1672:dbl, "Elapsed Time (s)"=w1668:dbl, "Time has Elapsed"=w1675:bool)  [unwired: 10 in, 5 out]
        "Calib 5" <- w1675
        n804 = Seconds To Date/Time(time stamp (now)=w1672) -> (date time rec=w1673:T2)  [unwired: 1 in]
        n805 = Not(x=w1675) -> (.not. x?=w1678:bool)
        n806 = script code="t = [0,20,23,27.5,30.5,35];\n\nevent = [0,1,2,1,2,14];\n\nfor i = 2:length(t)\n    if ((x>=t(i-1)) &&  (x<t(i)))\n        y = event(i-1);\n        yNext = event(i);\n        dt = t(i) - t(i-1);\n        break;\n    end\nend"("x"=w1668) -> ("y"=w1669:dbl, "dt"=w1670:dbl, "yNext"=w1671:dbl)  [unwired: 1 in, 1 out]
        n807 = case shown="True" w1678 {
          tunnel: [w1717 w1729] -> w1677
          frame False {
            n808 = flat-sequence {
              tunnel: [w1725] -> w1717
              frame #0 {
                n809 = local write "Buffer"(FALSE ("Buffer")) -> ()
                n810 = local write "Play/Stop"(FALSE ("Play\nCalibration")) -> ()
              }
              frame #1 {
                n811 = local write "Output"(0 ("Output")) -> ()
                n812 = local write "Save"(TRUE ("Save")) -> ()
              }
              frame #2 {
                n813 = Wait (ms)(milliseconds to wait=u32 500) -> ()  [unwired: 1 out]
              }
              frame #3 {
                n814 = local write "Flush"(TRUE ("Flush")) -> ()
              }
              frame #4 {
                w1724 = u16 0 items=["No sound", "Demo deep breathing", "Demo fast shallow breathing", "Demo slow shallow breathing", "Demo breath hold", "Demo cough/ laugh", "Demo abdomen movement", "Calibration", "Routine 1", "Routine 3", "Routine 4/5/7", "Calm music"] ("Play sound")
                w1725 = enum16{"Default"}."Default"
                n815 = local write "Flush"(FALSE ("Flush")) -> ()
                n816 = local write "Save"(FALSE ("Save")) -> ()
                n817 = local write "Play sound"(w1724) -> ()
                n818 = local write "Routine"(w1725) -> ()
              }
            }
          }
          frame True {
            w1728 = u16 7 items=["No sound", "Demo normal breathing", "Demo deep breathing", "Demo fast shallow breathing", "Demo breath hold", "Demo cough", "Demo abdomen movement", "Calibration", "Routine 1", "(2a)Calm music", "(2b)Stress test", "Routine 3/4", "Routine 5", ""] ("Play sound")
            n819 = local write "Play sound"(w1728) -> ()
            n820 = flat-sequence {
              tunnel: [T4."Calib4"] -> w1729
              frame #0 {
                n821 = local write "Output"(1 ("Open")) -> ()
                n822 = local write "Play/Stop"(TRUE ("Play\nCalibration")) -> ()
              }
              frame #1 {
                n823 = local write "Buffer"(TRUE ("Buffer")) -> ()
              }
              frame #2 {
              }
            }
          }
        }
        n824 = case shown="0, Default" w1669 {
          tunnel: ["\nPerform normal breathing." "Inhale a slow deep breath." "\nExhale slowly." "Quick inhale.\n\n\n\nIf you cannot sustain for long, resume normal breathing." "\nQuick exhale.\n\n\nIf you cannot sustain for long, resume normal breathing." "Slow shallow inhale.\n\n\n\nIf you cannot sustain for long, resume normal breathing." "\nSlow exhale.\n\n\nIf you cannot sustain for long, resume normal breathing." "Exhale the current breath  and HOLD.\n\n\nIf you cannot sustain for long, resume normal breathing." "Perform voluntary coughing \n" "Perform voluntary laugh\n\n" "Read aloud the following text in between the lines:\n-----------------------------------------------------------------------\nFour score and seven years ago our fathers brought forth on this continent, a new nation, conceived in Liberty, and dedicated to the proposition that all men are created equal… That this nation, under God, shall have a new birth of freedom-and that government of the people, by the people, for the people, shall not perish from the earth.\n\n-----------------------------------------------------------------------\nWhen finished, take a deep breath and open mouth say \"Ah\" (like doctor checking your throat).\nPerform normal breathing until next instruction." "Exhale current breath and HOLD. Push abdomen inwards." "Relax abdomen back to normal and keep holding breath."] -> w1667
          frame 0, Default {
          }
          frame 1 {
          }
          frame 2 {
          }
          frame 3 {
          }
          frame 4 {
          }
          frame 5 {
          }
          frame 6 {
          }
          frame 7 {
          }
          frame 8 {
          }
          frame 9 {
          }
          frame 10 {
          }
          frame 12 {
          }
          frame 13 {
          }
        }
        n825 = case shown="14" w1671 {
          tunnel: ["\nPerform normal breathing." "Inhale a slow deep breath." "\nExhale slowly." "Quick inhale.\n\n\n\nIf you cannot sustain for long, resume normal breathing." "\nQuick exhale.\n\n\nIf you cannot sustain for long, resume normal breathing." "Slow shallow inhale.\n\n\n\nIf you cannot sustain for long, resume normal breathing." "\nSlow exhale.\n\n\nIf you cannot sustain for long, resume normal breathing." "Exhale the current breath  and HOLD.\n\n\nIf you cannot sustain for long, resume normal breathing." "Perform voluntary coughing \n" "Perform voluntary laugh\n\n" "Read aloud the following text in between the lines:\n-----------------------------------------------------------------------\nFour score and ...\n-----------------------------------------------------------------------\nWhen finished, take a deep breath and open mouth say \"Ah\" (like doctor checking your throat).\nPerform normal breathing until next instruction." "Exhale current breath and HOLD. Push abdomen inwards." "Relax abdomen back to normal and keep holding breath." "Wait for next routine. Please do not move."] -> w1665
          frame 0, Default {
          }
          frame 1 {
          }
          frame 2 {
          }
          frame 3 {
          }
          frame 4 {
          }
          frame 5 {
          }
          frame 6 {
          }
          frame 7 {
          }
          frame 8 {
          }
          frame 9 {
          }
          frame 10 {
          }
          frame 12 {
          }
          frame 13 {
          }
          frame 14 {
          }
        }
        n826 = case shown="0, Default" w1669 {
          tunnel: w1670 -> [w1681 w1683 w1685 w1687 w1689]
          tunnel: [w1680 w1682 w1684 w1686 w1688] -> w1666
          frame 1 {
            n827 = property on="Current Task time" class="Slide (strict)"("Scale.Maximum"=w1681) -> ()  [unwired: 2 in, 2 out]
            n828 = call "Elapsed Time89"("Time Target (s)"=w1681) -> ("Elapsed Time (s)"=w1680:dbl)  [unwired: 11 in, 7 out]
          }
          frame 2 {
            n829 = property on="Current Task time" class="Slide (strict)"("Scale.Maximum"=w1683) -> ()  [unwired: 2 in, 2 out]
            n830 = call "Elapsed Time90"("Time Target (s)"=w1683) -> ("Elapsed Time (s)"=w1682:dbl)  [unwired: 11 in, 7 out]
          }
          frame 3 {
            n831 = property on="Current Task time" class="Slide (strict)"("Scale.Maximum"=w1685) -> ()  [unwired: 2 in, 2 out]
            n832 = call "Elapsed Time91"("Time Target (s)"=w1685) -> ("Elapsed Time (s)"=w1684:dbl)  [unwired: 11 in, 7 out]
          }
          frame 4 {
            n833 = property on="Current Task time" class="Slide (strict)"("Scale.Maximum"=w1687) -> ()  [unwired: 2 in, 2 out]
            n834 = call "Elapsed Time92"("Time Target (s)"=w1687) -> ("Elapsed Time (s)"=w1686:dbl)  [unwired: 11 in, 7 out]
          }
          frame 0, Default {
            n835 = property on="Current Task time" class="Slide (strict)"("Scale.Maximum"=w1689) -> ()  [unwired: 2 in, 2 out]
            n836 = call "Elapsed Time93"("Time Target (s)"=w1689) -> ("Elapsed Time (s)"=w1688:dbl)  [unwired: 11 in, 7 out]
          }
        }
      }
    }
    "CaseNum" <- w1020
    "Elapsed Time (s)" <- w1018
    "Current Task" <- w1019
    "Total Routine Time" <- w1018
    "date time rec" <- w1017
    "Current Task time" <- w1016
    "Next Task" <- w1014
    n837 = Wait (ms)(milliseconds to wait=u32 2 ("millisecond timer value")) -> ()  [unwired: 1 out]
    n838 = property on="Current Task time" class="Slide (strict)"("Scale.Minimum"=0.0 ("Scale.Range:Minimum")) -> ()  [unwired: 2 in, 2 out]
  }
  n839 = while {
    tunnel: w108 -> [w1737]
    tunnel: w102 -> [w1736]
    stop <- FALSE stop-if-true
    n840 = Get Queue Status(queue=w1737) -> (queue out=w1739:refnum<queue>, # elements in queue=w1740:i32)  [unwired: 2 in, 6 out]
    "# queue 2" <- w1740
    n841 = Wait (ms)(milliseconds to wait=u32 20) -> ()  [unwired: 1 out]
    n842 = local read "Save"() -> (w1734:bool)
    n843 = case shown="True" w1734 {
      tunnel: w1740 -> [_ w1774]
      tunnel: w1739 -> [_ w1776]
      tunnel: w1736 -> [_ w1773]
      frame False {
      }
      frame True {
        n844 = Multiply(x=w1774, y=w1773) -> (x*y=w1746:dbl)
        n845 = local read "date time rec"() -> (w1767:T2)
        n846 = for {
          N: w1774 -> [_]
          tunnel: [w1846] -> w1775 mode=indexing
          tunnel: [w1844] -> w1772 mode=indexing
          shift-right: [w1842] -> _
          shift-left: w1776 -> [w1848]
          tunnel: [w1838] -> w1748 mode=indexing
          tunnel: [w1837] -> w1747 mode=indexing
          i -> [w1843]
          n847 = Dequeue Element(queue=w1848) -> (queue out=w1842:refnum<queue>, element=w1839:dbl[][])  [unwired: 2 in, 2 out]
          n848 = Index Array(array=w1839, index (row)=2) -> (element=w1838:dbl[])  [unwired: 1 in]
          n849 = Index Array(array=w1839, index (row)=3) -> (element=w1837:dbl[])  [unwired: 1 in]
          n850 = Index Array(array=w1839, index (row)=1) -> (element=w1844:dbl[])  [unwired: 1 in]
          n851 = Index Array(array=w1839, index (row)=0) -> (element=w1846:dbl[])  [unwired: 1 in]
          "IterationNum" <- w1843
        }
        n852 = Unbundle By Name(w1767) -> ("fractional second"=w1760:dbl, "second"=w1761:i32, "minute"=w1762:i32, "hour"=w1763:i32, "day of month"=w1764:i32, "month"=w1765:i32, "year"=w1766:i32)
        n853 = property on="month" class="DigNum (strict)"() -> ("Label.Text"=w1757:string)  [unwired: 2 in, 2 out]
        n854 = property on="year" class="DigNum (strict)"() -> ("Label.Text"=w1758:string)  [unwired: 2 in, 2 out]
        n855 = property on="hour" class="DigNum (strict)"() -> ("Label.Text"=w1755:string)  [unwired: 2 in, 2 out]
        n856 = property on="day" class="DigNum (strict)"() -> ("Label.Text"=w1756:string)  [unwired: 2 in, 2 out]
        n857 = property on="fractionalSecond" class="DigNum (strict)"() -> ("Label.Text"=w1752:string)  [unwired: 2 in, 2 out]
        n858 = property on="second" class="DigNum (strict)"() -> ("Label.Text"=w1753:string)  [unwired: 2 in, 2 out]
        n859 = property on="minute" class="DigNum (strict)"() -> ("Label.Text"=w1754:string)  [unwired: 2 in, 2 out]
        n860 = Format Date/Time String(time format string (%c)="%m%d_%H%M%S") -> (date/time string=w1750:string)  [unwired: 2 in]
        n861 = call <vilib>:"Application Directory.vi"() -> ("Application Directory"=w1743:path)
        n862 = Build Path(base path=w1743, name or relative path="data") -> (appended path=w1741:path)
        n863 = property on="Routine" class="Ring (strict)"() -> ("RingText.Text"=w1769:string)  [unwired: 2 in, 2 out]
        n864 = Concatenate Strings(w1750, w1769) -> (w1768:string)
        n865 = flat-sequence {
          tunnel: w1768 -> [w1826]
          tunnel: w1741 -> [w1832]
          tunnel: "Case Number" -> [w1829]
          tunnel: w1771 -> [w1791]
          tunnel: w1770 -> [w1790]
          tunnel: w1766 -> [w1823]
          tunnel: w1765 -> [w1818]
          tunnel: w1764 -> [w1813]
          tunnel: w1763 -> [w1812]
          tunnel: w1762 -> [w1811]
          tunnel: w1761 -> [w1806]
          tunnel: w1760 -> [w1805]
          tunnel: w1758 -> [w1804]
          tunnel: w1757 -> [w1803]
          tunnel: w1756 -> [w1802]
          tunnel: w1755 -> [w1801]
          tunnel: w1754 -> [w1800]
          tunnel: w1753 -> [w1799]
          tunnel: w1752 -> [w1798]
          tunnel: "Comments" -> [w1793]
          tunnel: w1745 -> [w1782]
          tunnel: w1744 -> [w1781]
          frame #0 {
            n866 = Build Path(base path=w1832, name or relative path=w1826) -> (appended path=w1835:path)
            n867 = TDMS Open(6:FALSE ("disable buffering (T)"), 10:T12."open or create" ("operation"), 11:w1835) -> (0:w1830:errorcluster, 3:w1831:refnum<k34>)  [unwired: 4 in]
            n868 = TDMS Set Properties(5:w1829, 7:"CaseNumber" ("property names"), 8:w1830, 11:w1831) -> (0:w1777:errorcluster, 3:w1778:refnum<k34>)  [unwired: 2 in, 2 out]
            n869 = TDMS Set Properties(5:w1793, 7:"Comments" ("property names"), 8:w1777, 11:w1778) -> (0:w1794:errorcluster, 3:w1795:refnum<k34>)  [unwired: 2 in, 2 out]
            n870 = TDMS Set Properties(5:w1823, 7:w1804, 8:w1794, 11:w1795) -> (0:w1822:errorcluster, 3:w1821:refnum<k34>)  [unwired: 2 in, 2 out]
            n871 = TDMS Set Properties(5:w1818, 7:w1803, 8:w1822, 11:w1821) -> (0:w1820:errorcluster, 3:w1819:refnum<k34>)  [unwired: 2 in, 2 out]
            n872 = TDMS Set Properties(5:w1813, 7:w1802, 8:w1820, 11:w1819) -> (0:w1817:errorcluster, 3:w1816:refnum<k34>)  [unwired: 2 in, 2 out]
            n873 = TDMS Set Properties(5:w1812, 7:w1801, 8:w1817, 11:w1816) -> (0:w1815:errorcluster, 3:w1814:refnum<k34>)  [unwired: 2 in, 2 out]
            n874 = TDMS Set Properties(5:w1811, 7:w1800, 8:w1815, 11:w1814) -> (0:w1810:errorcluster, 3:w1809:refnum<k34>)  [unwired: 2 in, 2 out]
            n875 = TDMS Set Properties(5:w1806, 7:w1799, 8:w1810, 11:w1809) -> (0:w1807:errorcluster, 3:w1808:refnum<k34>)  [unwired: 2 in, 2 out]
            n876 = TDMS Set Properties(5:w1805, 7:w1798, 8:w1807, 11:w1808) -> (0:w1796:errorcluster, 3:w1797:refnum<k34>)  [unwired: 2 in, 2 out]
            n877 = TDMS Write(0:w1797, 7:"Tx1Rx1Amp" ("channel name(s) in (Untitled)"), 9:w1790, 11:w1796) -> (4:w1825:refnum<k34>, 15:w1824:errorcluster)  [unwired: 2 in, 2 out]
            n878 = TDMS Write(0:w1825, 7:"Tx2Rx2Amp" ("channel name(s) in (Untitled)"), 9:w1791, 11:w1824) -> (4:w1788:refnum<k34>, 15:w1785:errorcluster)  [unwired: 2 in, 2 out]
            n879 = TDMS Write(0:w1788, 7:"Tx1Rx1Ph" ("channel name(s) in (Untitled)"), 9:w1781, 11:w1785) -> (4:w1787:refnum<k34>, 15:w1784:errorcluster)  [unwired: 2 in, 2 out]
            n880 = TDMS Write(0:w1787, 7:"Tx2Rx2Ph" ("channel name(s) in (Untitled)"), 9:w1782, 11:w1784) -> (4:w1786:refnum<k34>, 15:w1783:errorcluster)  [unwired: 2 in, 2 out]
            n881 = TDMS Close(8:w1783, 11:w1786) -> ()  [unwired: 2 out]
          }
          frame #1 {
            n882 = local write "Save"(FALSE) -> ()
          }
        }
        n883 = Reshape Array(w1747, w1746) -> (w1745:dbl[])
        n884 = Reshape Array(w1748, w1746) -> (w1744:dbl[])
        n885 = Reshape Array(w1772, w1746) -> (w1771:dbl[])
        n886 = Reshape Array(w1775, w1746) -> (w1770:dbl[])
      }
    }
  }
  n887 = local read "DownSamplingRatio"() -> (w117:i32)
  n888 = local read "Waveform Size"() -> (w118:dbl)
  n889 = Divide(x=w118, y=w117) -> (x/y=w105:dbl)
  n890 = Divide(x=w105, y="DownSamplingRatio 2") -> (x/y=w94:dbl)
  n891 = Multiply(x=w96, y=w94) -> (x*y=w112:dbl)
  n892 = Initialize Array(w95, w96, w94) -> (w114:dbl[][])
  n893 = Initialize Array(w95, w96, w94) -> (w113:dbl[][])
  n894 = Initialize Array(w95, w96, w94) -> (w116:dbl[][])
  n895 = Initialize Array(w95, w96, w94) -> (w115:dbl[][])
  n896 = while {
    tunnel: w96 -> [w1920]
    tunnel: w89 -> [w1913]
    shift-right: [w1910] -> _
    shift-left: w116 -> [w1882]
    tunnel: w112 -> [w1871]
    shift-right: [w1901] -> _
    shift-left: w115 -> [w1916]
    shift-right: [w1900] -> _
    shift-left: w114 -> [w1915]
    shift-right: [w1899] -> _
    shift-left: w113 -> [w1914]
    tunnel: "DownSamplingRatio 2" -> [w1852]
    tunnel: w94 -> [w1853]
    tunnel: "DownSamplingRatio 2" -> [w1872]
    stop <- FALSE stop-if-true
    # "Amp2"
    # "Amp1"
    # "Downsampling only for viewing."
    n897 = local read "Sampling Rate"() -> (w1873:dbl)
    n898 = Get Queue Status(queue=w1913) -> (# elements in queue=→"# elements in queue":i32)  [unwired: 2 in, 7 out]
    n899 = Dequeue Element(queue=w1913) -> (element=w1854:dbl[][])  [unwired: 2 in, 3 out]
    n900 = Decrement(x=w1920) -> (x-1=w1869:i32)
    n901 = Divide(x=w1873, y=w1872) -> (x/y=→"Dis Sampling Rate":dbl)
    n902 = Index Array(array=w1854, index (row)=0 ("index")) -> (element=w1880:dbl[])  [unwired: 1 in]
    n903 = Index Array(array=w1854, index (row)=1 ("index")) -> (element=w1879:dbl[])  [unwired: 1 in]
    n904 = Index Array(array=w1854, index (row)=2 ("index")) -> (element=w1860:dbl[])  [unwired: 1 in]
    n905 = Index Array(array=w1854, index (row)=3 ("index")) -> (element=w1859:dbl[])  [unwired: 1 in]
    n906 = Reshape Array(w1879, w1853, w1852) -> (w1876:dbl[][])
    n907 = Reshape Array(w1880, w1853, w1852) -> (w1878:dbl[][])
    n908 = Reshape Array(w1860, w1853, w1852) -> (w1858:dbl[][])
    n909 = Reshape Array(w1859, w1853, w1852) -> (w1857:dbl[][])
    n910 = for {
      tunnel: w1876 -> [w1934] mode=indexing
      tunnel: [w1933] -> w1875 mode=indexing
      n911 = Add Array Elements(numeric array=w1934) -> (sum=w1933:dbl)
    }
    n912 = for {
      tunnel: w1858 -> [w1932] mode=indexing
      tunnel: [w1931] -> w1856 mode=indexing
      n913 = Add Array Elements(numeric array=w1932) -> (sum=w1931:dbl)
    }
    n914 = for {
      tunnel: w1857 -> [w1930] mode=indexing
      tunnel: [w1929] -> w1855 mode=indexing
      n915 = Add Array Elements(numeric array=w1930) -> (sum=w1929:dbl)
    }
    n916 = for {
      tunnel: w1878 -> [w1936] mode=indexing
      tunnel: [w1935] -> w1877 mode=indexing
      n917 = Add Array Elements(numeric array=w1936) -> (sum=w1935:dbl)
    }
    n918 = Array Subset(array=w1915, index (row)=0 ("index"), length (row)=w1869) -> (w1903:dbl[][])  [unwired: 2 in]
    n919 = Array Subset(array=w1914, index (row)=0 ("index"), length (row)=w1869) -> (w1902:dbl[][])  [unwired: 2 in]
    n920 = Array Subset(array=w1916, index (row)=0 ("index"), length (row)=w1869) -> (w1904:dbl[][])  [unwired: 2 in]
    n921 = Array Subset(array=w1882, index (row)=0 ("index"), length (row)=w1869) -> (w1911:dbl[][])  [unwired: 2 in]
    n922 = Divide(x=w1877, y=w1852) -> (x/y=w1863:dbl[])
    n923 = Divide(x=w1875, y=w1852) -> (x/y=w1850:dbl[])
    n924 = Divide(x=w1856, y=w1852) -> (x/y=w1851:dbl[])
    n925 = Divide(x=w1855, y=w1852) -> (x/y=w1849:dbl[])
    n926 = Build Array (concatenate)(w1849, w1902) -> (w1899:dbl[][])
    n927 = Build Array (concatenate)(w1851, w1903) -> (w1900:dbl[][])
    n928 = Build Array (concatenate)(w1850, w1904) -> (w1901:dbl[][])
    n929 = local read "Dis Sampling Rate"() -> (w1870:dbl)
    n930 = Build Array (concatenate)(w1863, w1911) -> (w1910:dbl[][])
    n931 = Reshape Array(w1899, w1871) -> (w1884:dbl[])
    n932 = Reshape Array(w1900, w1871) -> (w1883:dbl[])
    n933 = Reshape Array(w1901, w1871) -> (w1885:dbl[])
    n934 = disable-structure shown="Enabled" {
      disable-tunnel: w1863 -> [w1926 _]
      disable-tunnel: w1851 -> [w1925 _]
      disable-tunnel: w1850 -> [w1928 _]
      disable-tunnel: w1849 -> [w1927 _]
      frame Enabled {
        "Amp2 @500Hz" <- w1928
        "Ph2 @500Hz" <- w1927
        "Amp1 @500Hz" <- w1926
        "Ph1 @500Hz" <- w1925
      }
      frame Disabled {
      }
    }
    n935 = Reshape Array(w1910, w1871) -> (w1886:dbl[])
    n936 = call-poly <vilib>:"Butterworth Filter.vi"("init/cont (init:F)"=TRUE, "order"=3, "filter type"=Filter_Passband_Type."Bandpass", "low cutoff freq: fl"="fl 3", "high cutoff freq: fh"="fh 3", "sampling freq: fs"=w1870, "X"=w1883) -> ("Filtered X"=w1865:dbl[])  [unwired: 1 in, 1 out]
    n937 = call-poly <vilib>:"Butterworth Filter.vi"("init/cont (init:F)"=TRUE, "order"=3, "filter type"=Filter_Passband_Type."Lowpass", "low cutoff freq: fl"="fl 4", "sampling freq: fs"=w1870, "X"=w1884) -> ("Filtered X"=w1864:dbl[])  [unwired: 2 in, 1 out]
    n938 = call-poly <vilib>:"Butterworth Filter.vi"("init/cont (init:F)"=TRUE, "order"=3, "filter type"=Filter_Passband_Type."Lowpass", "low cutoff freq: fl"="fl 2", "sampling freq: fs"=w1870, "X"=w1885) -> ("Filtered X"=w1887:dbl[])  [unwired: 2 in, 1 out]
    n939 = call-poly <vilib>:"Butterworth Filter.vi"("init/cont (init:F)"=TRUE, "order"=3, "filter type"=Filter_Passband_Type."Bandpass", "low cutoff freq: fl"="fl 1", "high cutoff freq: fh"="fh 1", "sampling freq: fs"=w1870, "X"=w1886) -> ("Filtered X"=w1888:dbl[])  [unwired: 1 in, 1 out]
    n940 = Build Array(w1888, w1887, w1865, w1864) -> (→"aapp":dbl[][])
  }
  n941 = while {
    stop <- FALSE stop-if-true
    n942 = local read "aapp"() -> (w1940:dbl[][])
    n943 = Index Array(array=w1940, index (row)=0 ("index")) -> (element=→"Heart Amp":dbl[])  [unwired: 1 in]
    n944 = Index Array(array=w1940, index (row)=1 ("index")) -> (element=→"Resp Amp":dbl[])  [unwired: 1 in]
    n945 = Index Array(array=w1940, index (row)=2 ("index")) -> (element=→"Heart Ph":dbl[])  [unwired: 1 in]
    n946 = Index Array(array=w1940, index (row)=3 ("index")) -> (element=→"Resp Ph":dbl[])  [unwired: 1 in]
    n947 = Wait (ms)(milliseconds to wait=u32 20) -> ()  [unwired: 1 out]
  }
  "error out" <- w76
  "error out 2" <- w75
